vi "Gel Tugging Force Mode_Controller v16.20 DIC.vi"() -> ()   [LabVIEW 2015]
doc: "This example demonstrates how to continuously acquire voltage measurements from a DAQmx device using hardware timed, single point reads using a timed loop structure. The timed loop is controlled by the sample clock of the DAQ device. The device will read data on each tick of the sample clock. If an additional sample clock tick occurs before the current data point is read from the device or if the timed loop does not receive any sample clock ticks, a dialog will indicate that this has happened. \n\nHardware Timed Single Point acquisition works best when using a deterministic operating system (such as LabVIEW Real-Time). Because of the less deterministic nature of general purpose operating systems (such as Microsoft Windows), the software loop will not always take the exact same amount of time to execute, and this may lead to the occasional missed sample clock. \n\nFor instructions on how to connect your signals to the DAQ device, refer to your device documentation."
uses:
  <vilib>/Platform/TimedLoop/XDataNode/timing_clust.ctl
  <vilib>/Platform/TimedLoop/XDataNode/nitl_modes.ctl
  <vilib>/Platform/TimedLoop/XDataNode/wakeup.ctl
  <vilib>/dex/Flush And Wait Empty Condition.ctl
  <vilib>/DAQmx/read.llb/DAQmx Read (Analog 1D DBL NChan 1Samp).vi
  <vilib>/DAQmx/write.llb/DAQmx Write (Analog DBL 1Chan 1Samp).vi
  <vilib>/DAQmx/read.llb/DAQmx Read (Analog 2D DBL NChan NSamp).vi
  <vilib>/Analysis/baseanly.llb/Mean (DBL).vi
  <vilib>/DAQmx/create/channels.llb/DAQmx Create Channel (AI-Voltage-Basic).vi
  <vilib>/DAQmx/create/channels.llb/DAQmx Create Channel (AO-Voltage-Basic).vi
  <vilib>/DAQmx/configure/timing.llb/DAQmx Timing (Sample Clock).vi
  <vilib>/DAQmx/create/timing.llb/DAQmx Create Timing Source (Control Loop From Task).vi
  <vilib>/DAQmx/miscellaneous.llb/DAQmx Fill In Error Info.vi
  <vilib>/addons/control/pid/pid.llb/PID (DBL).vi
  <vilib>/addons/control/pid/pid.llb/PID Gain Schedule (DBL).vi
  <vilib>/platform/TimedLoop/XDataNode/XDataNode.xnode
  <vilib>/Analysis/NI_AALBase.lvlib
  <vilib>/addons/control/pid/NI_PID_pid.lvlib
  <vilib>/Platform/TimedLoop/XDataNode/XDNodeRunTimeDep.lvlib
  <vilib>/ptbypt/NI_PtbyPt.lvlib
panel:
  out "Zero Flux Observed GS":dbl
  in  "Start Null Flux Adjustment":bool=TRUE
  in  "3. Keep Null Flux Running \n       Until Next Step?":bool=TRUE
  in  "2. Adjust Magnetic Flux (GS):":dbl=3.0 min=-350.0 max=350.0 step=0.02 format="%#_13g"
  in  "4. Click Rocker to finish Null Flux Adjustment":bool
  out "Total seconds":dbl format="%.3f"
  out "Loop Index 2":dbl format="%.3f"
  out "Final AO (V)":dbl
  in  "1st OFF Length (s)":dbl=2.0
  out "Calibrating Sensor":bool
  out "Waveform Graph 2":dbl[](graph)
  in  "ON":dbl=3.0
  out "DigitalTrigger":bool
  out "Corrective \nNull Flux (Gs)":dbl
  out "# of Data Points":i64
  out "Loop Index":i32
  in  "Measure Flux Sensor Zero?":bool=TRUE
  out "PID gains ON Chosen":T1
  in  "Keep Null Flux Running \n       Until Next Step? 2":bool
  in  "Start Null Flux Adjustment 2":bool=TRUE
  out "PID gains OFF Chosen":T1
  in  "Tweaked PID gains ON":T1={"proportional gain (Kc)"=0.7, "integral time (Ti, min)"=3.5e-06, "derivative time (Td, min)"=0.0}
  in  "Tweaked PID gains OFF":T1={"proportional gain (Kc)"=0.078, "integral time (Ti, min)"=3.5e-06, "derivative time (Td, min)"=0.0}
  out "Ready?":bool
  in  "4. Aggressiveness:":i32(listbox)
  out "of":i32
  in  "3. PID Parameters:":i32(listbox)
  out "ON Absolute\nFlux Setpoint (Gs)":dbl
  out "Suggested PID gains OFF":T1
  out "Suggested PID gains ON":T1
  out "Measured Magnetic Sensor 1 Zero, Mean (V)":dbl format="%_7g"
  in  "2nd to last\n OFF (s)":dbl=7.0
  out "Round:":i32
  out "Ready?":bool
  out "Ready?":bool
  in  "Proceed with Parameters":bool=TRUE
  out "Final Flux Running at End?":bool
  out "Sensor Sensitivity \n(V/Gs)":dbl
  in  "1. Sensor:":i32(listbox)
  out "Ready?":bool
  in  "2. Needle:":i32(listbox)
  in  "Proceed with Selection":bool=TRUE
  in  "Ready?&\nData Logger Running":bool
  out "Null Flux \nCurrently\nRunning?":bool
  out "Real-Time Flux Control Currently Running?":bool
  out "Ready?":bool
  out "DeGaussing?":bool
  in  "Start DeGaussing":bool
  in  "1. Number of rounds":i32=3
  in  "Post-Wave Null Flux Interval (s)":dbl=7.5 format="%#_13g"
  in  "Pre-Wave Null Flux Interval (s)":dbl format="%#_13g"
  out "Flux Control Sequence Running & Uploading Data?":bool
  in  "Number of Cycles":i32=3
  in  "Flux ON relative setpoint (Gs)":dbl=-175.0 format="%#_13g"
  # "For Gel Tugging Experiments v16.20 (Controlled-Flux or Force Mode: DIC Part)"
  # "WARNING: This program can crash the first 2 or 3 times it runs after the target has been shut down. \nWARNING: Do NOT run the power supply unattended with the needle attached. Always check on the amount of current periodically."
  # "Step 0-1: Place the needle at Z ~ 7000 micron in the field of view. Inclincation Angle= 25º for HyMu80#1 Needle"
  # "(Hit \"Enter\" \nor Toggle)"
  # "Step 0-2: DeGauss Needle:"
  # "Step 0-3: Measure the Value of Flux Sensor \"Zero\"?"
  # "Yes"
  # "No"
  # "(Note: Check if it is around 2.47±0.02 (V)):"
  # "Step 1: Choose Sensor & \nNeedle/PID Parameters\nfor This Experiment:"
  # "Step 2: Adjust Flux: \n(in Real-Time)"
  # "(Hit \"Enter\" \nor Toggle)"
  # "Yes"
  # "No"
  # "Make sure upper side of Rocker\n is pressed down before Program Starts"
  # "Step 3: Specify Control \n     Sequence Parameters:"
  # "1. Pre-Wave Null Flux Interval (s) (choose 0 if none desired):"
  # "2. Length of 1st OFF"
  # "& ON"
  # "segments (s)."
  # "Length of 2nd to last OFF"
  # "Note 1: Use Negative Flux for waves in opposite direction\nNote 2: Linear Range is (±0-175 Gs) for Null Flux + Flux ON Setpoint\nNote 3: Check ON Absolute Flux Setpoint & PID Gains on first run.\nSometimes they can be glitchy. Abort & Re-run"
  # "3. Number of OFF & ON Square-Wave Cycles:"
  # "4. Flux ON relative setpoint (Gs):"
  # "5. Post-Wave Null Flux Inteval (s) (choose 0 if none desired):"
  # "No"
  # "Yes"
  # "Step 4: Do you want to tweak these PID parameters?"
  # "vs."
  # "Step 5: Run Data Logger: Gel Tugging Force Mode_Data Logger v16.10 DIC.vi\n            Needs to be running to start the control sequence"
  # "Step 6-1: Lower the needle to the desired level for the experiment. Z ~ 3400 microns with TI-SH-U stage.\nStep 6-2: Click TRGR or Run Macro in Nikon Elements"
  # "datapoints uploaded"
  # "out of"
  # "seconds elapsed"
  # "out of"
  # "Close the VI and start over. The VI sometimes freezes upon subsequent runs"
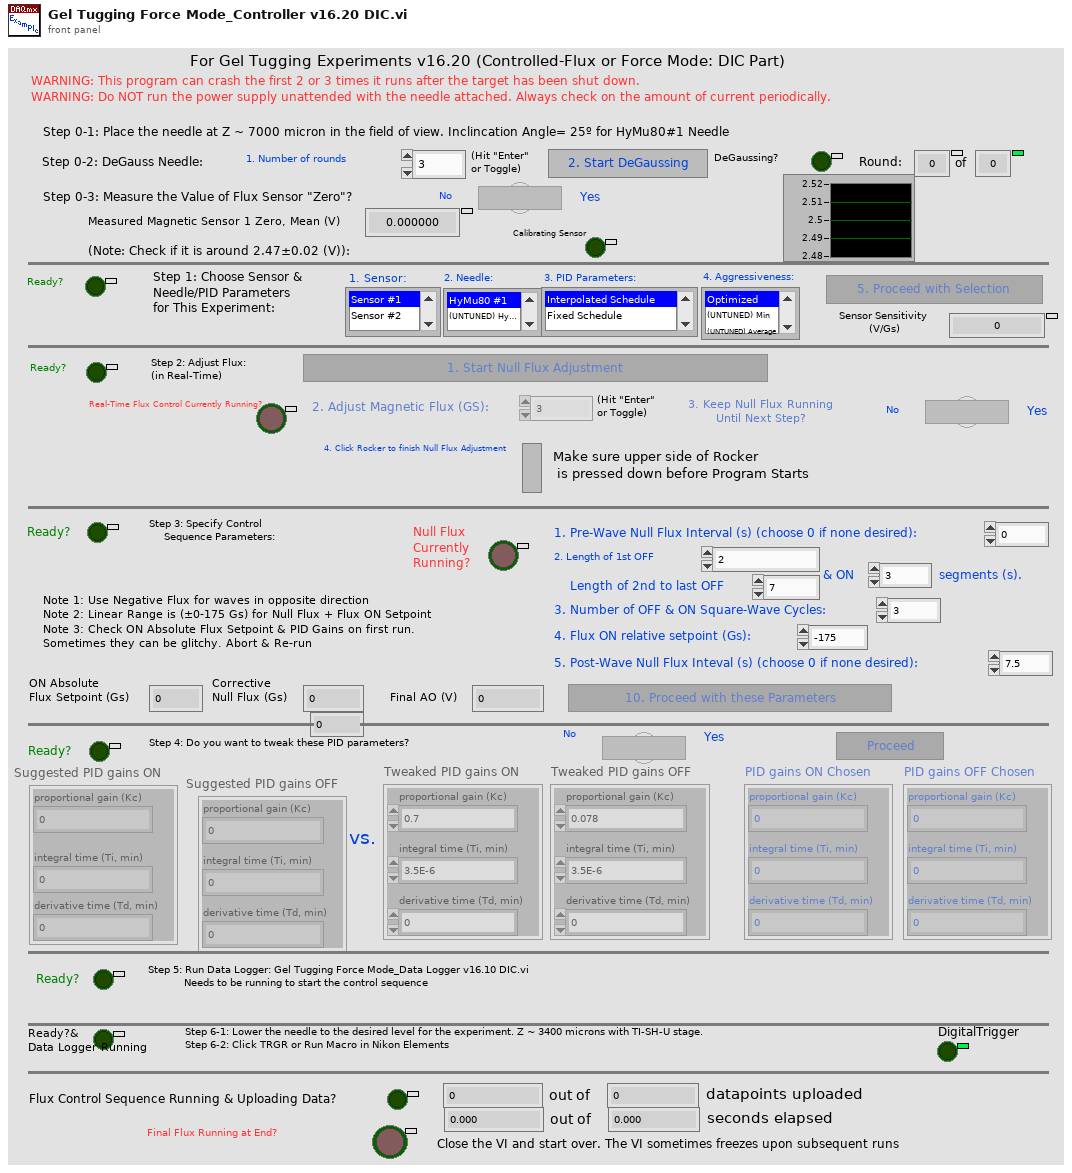
[diagram p1: front panel]
types:
  T1 = cluster{"proportional gain (Kc)":dbl, "integral time (Ti, min)":dbl, "derivative time (Td, min)":dbl}
  T2 = cluster{"PID gains":cluster{"proportional gain (Kc)":dbl, "integral time (Ti, min)":dbl, "derivative time (Td, min)":dbl}, "max value":dbl}[]
  T3 = typedef "XDNodeRunTimeDep.lvlib/timing_clust.ctl" = cluster{"Expected End [f-1]":u64, "Actual End [f-1]":u64, "Finished Late? [f-1]":bool, "Expected End [i-1]":u64, "Actual End [i-1]":u64, "Finished Late? [i-1]":bool, "Expected Start [i]":u64, "Actual Start [i]":u64, "Expected Start [f]":u64, "Actual Start [f]":u64, "Source Name":string, "Structure Name":string, "Period":i64, "Deadline":i64, "Offset":i64, "Start":i64, "Priority":i32, "Timeout":i32, "Mode":T4, "Wakeup Reason":T5, "Error":errorcluster, "Source Type":string, "Secondary Source Type":string, "Global End Time":u64, "Global Start Time":u64, "Frame Duration":u64, "Iteration Duration":u64, "Assigned CPU":i32, "I/O Scan Engine Mode":u32}
  T4 = typedef "XDNodeRunTimeDep.lvlib/nitl_modes.ctl" = enum32{"No Change", "Process missed periods, maintain original phase", "Discard missed periods, maintain original phase", "Process missed periods, ignore original phase", "Discard missed periods, ignore original phase"}
  T5 = typedef "XDNodeRunTimeDep.lvlib/wakeup.ctl" = enum32{"Normal", "Aborted", "Asynchronous wakeup", "Timing source error", "Timed loop error", "Timeout"}
  T6 = cluster{"Max/Min \ncontroller outputs":dbl, "output low":dbl}
  T7 = cluster{"PID gains":cluster{"proportional gain (Kc)":dbl, "integral time (Ti, min)":dbl, "derivative time (Td, min)":dbl}, "max value":dbl}
  T8 = typedef "Flush And Wait Empty Condition.ctl" = u8
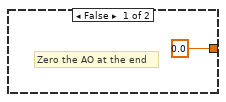
[diagram p2: hidden frame]
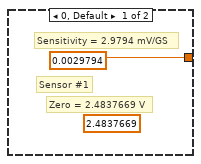
[diagram p4: hidden frame]
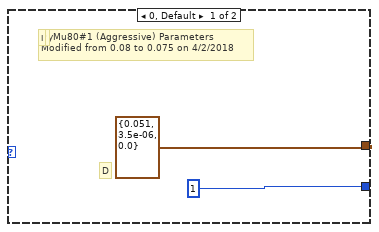
[diagram p5: hidden frame]
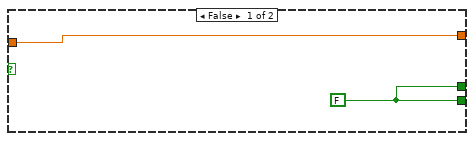
[diagram p6: hidden frame]
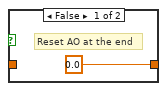
[diagram p7: hidden frame]
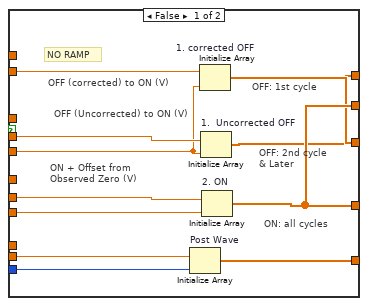
[diagram p9: hidden frame]
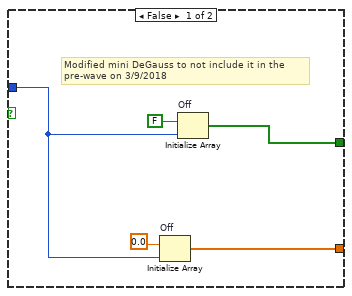
[diagram p11: hidden frame]
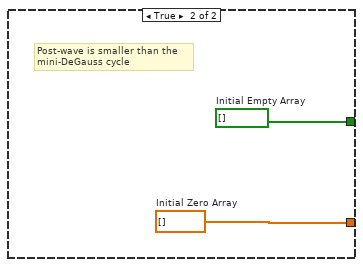
[diagram p12: hidden frame]
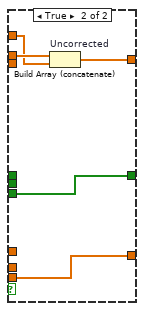
[diagram p14: hidden frame]
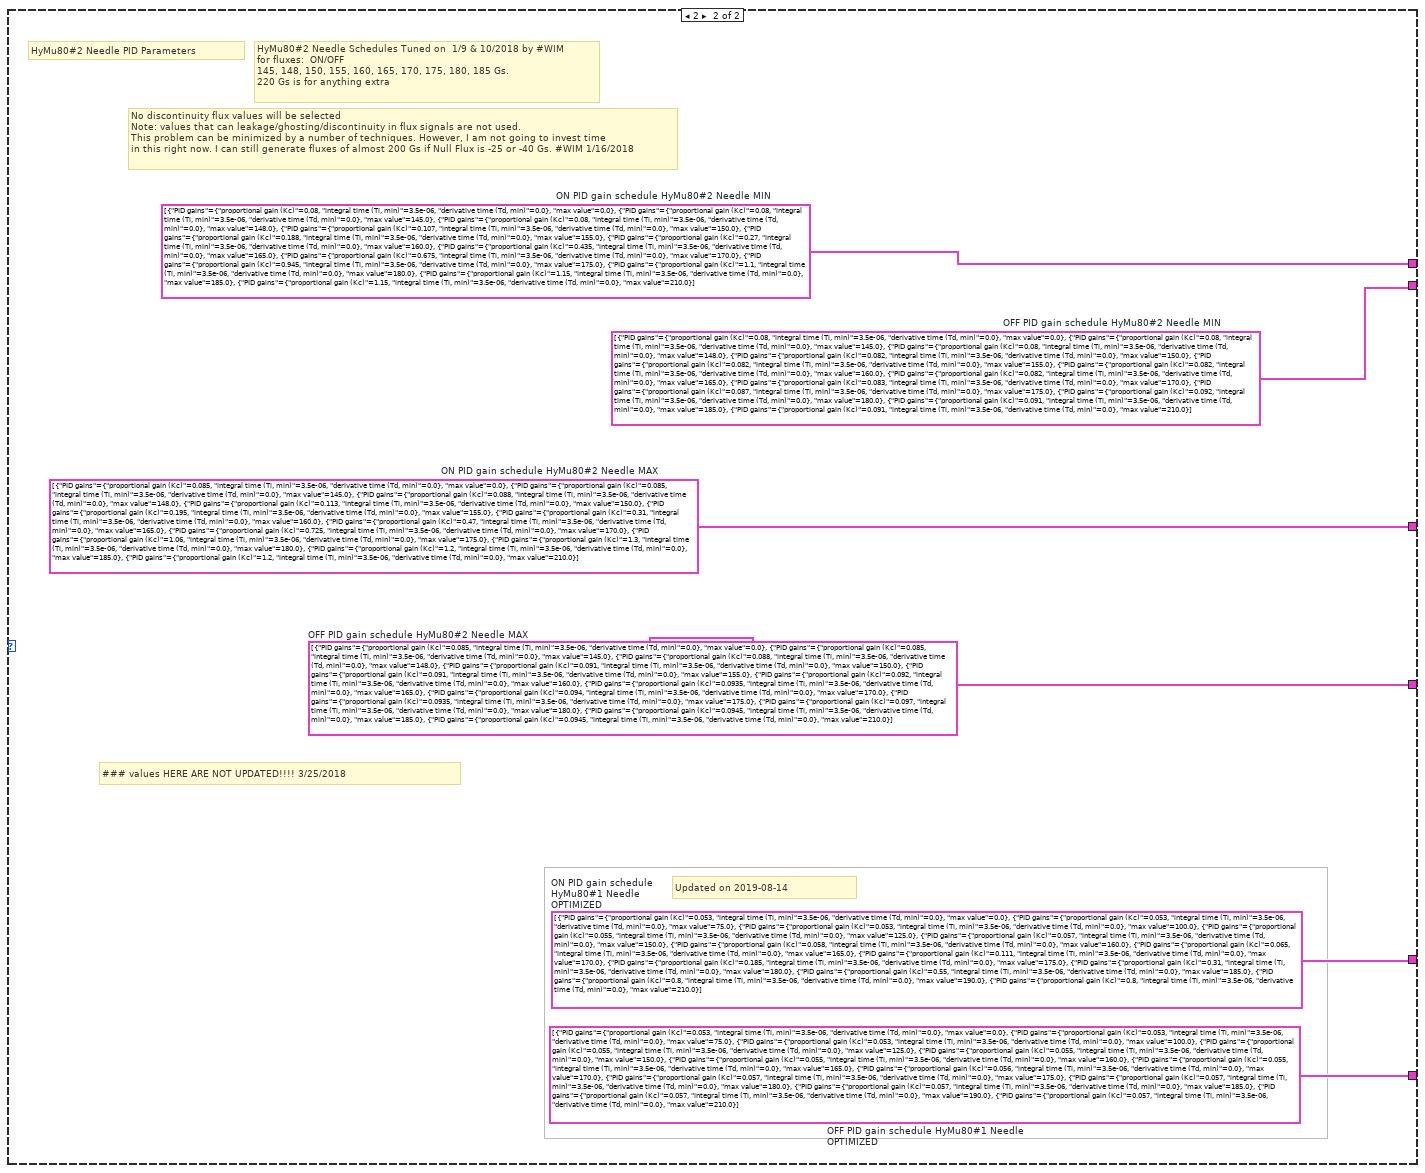
[diagram p18: hidden frame]
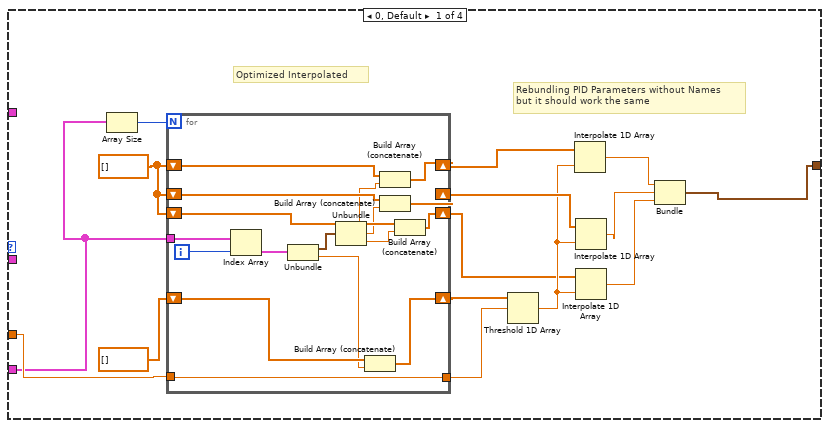
[diagram p19: hidden frame]
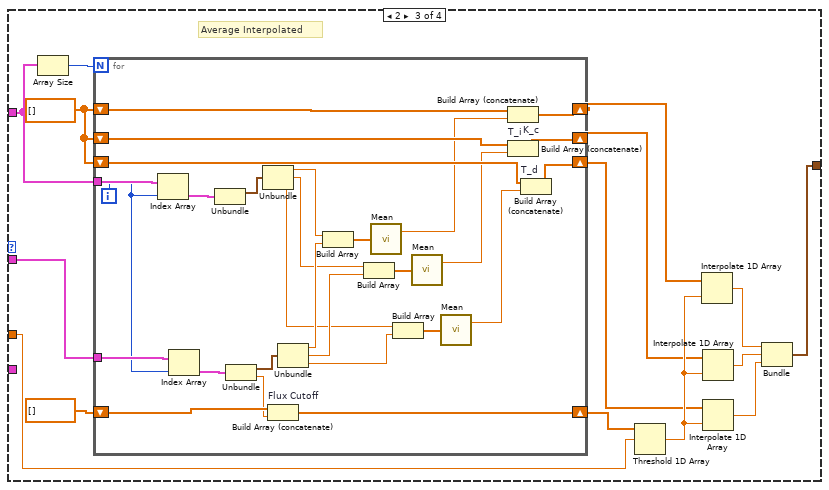
[diagram p20: hidden frame]
diagram:
  (unwired) T2 [{"PID gains"={"proportional gain (Kc)"=0.07, "integral time (Ti, min)"=3.5e-06, "derivative time (Td, min)"=0.0}, "max value"=0.0}, {"PID gains"={"proportional gain (Kc)"=0.07, "integral time (Ti, min)"=3.5e-06, "derivative time (Td, min)"=0.0}, "max value"=143.0}, {"PID gains"={"proportional gain (Kc)"=0.078, "integral time (Ti, min)"=3.5e-06, "derivative time (Td, min)"=0.0}, "max value"=148.0}, {"PID gains"={"proportional gain (Kc)"=0.078, "integral time (Ti, min)"=3.5e-06, "derivative time (Td, min)"=0.0}, "max value"=150.0}, {"PID gains"={"proportional gain (Kc)"=0.078, "integral time (Ti, min)"=3.5e-06, "derivative time (Td, min)"=0.0}, "max value"=155.0}, {"PID gains"={"proportional gain (Kc)"=0.078, "integral time (Ti, min)"=3.5e-06, "derivative time (Td, min)"=0.0}, "max value"=160.0}, {"PID gains"={"proportional gain (Kc)"=0.078, "integral time (Ti, min)"=3.5e-06, "derivative time (Td, min)"=0.0}, "max value"=165.0}, {"PID gains"={"proportional gain (Kc)"=0.078, "integral time (Ti, min)"=3.5e-06, "derivative time (Td, min)"=0.0}, "max value"=170.0}, {"PID gains"={"proportional gain (Kc)"=0.081, "integral time (Ti, min)"=3.5e-06, "derivative time (Td, min)"=0.0}, "max value"=175.0}, {"PID gains"={"proportional gain (Kc)"=0.081, "integral time (Ti, min)"=3.5e-06, "derivative time (Td, min)"=0.0}, "max value"=180.0}, {"PID gains"={"proportional gain (Kc)"=0.085, "integral time (Ti, min)"=3.5e-06, "derivative time (Td, min)"=0.0}, "max value"=185.0}, {"PID gains"={"proportional gain (Kc)"=0.086, "integral time (Ti, min)"=3.5e-06, "derivative time (Td, min)"=0.0}, "max value"=190.0}, {"PID gains"={"proportional gain (Kc)"=0.086, "integral time (Ti, min)"=0.01, "derivative time (Td, min)"=0.0}, "max value"=195.0}, {"PID gains"={"proportional gain (Kc)"=0.086, "integral time (Ti, min)"=0.01, "derivative time (Td, min)"=0.0}, "max value"=220.0}]  # OFF PID gain schedule HyMu80#1 Needle OPTIMIZED
  (unwired) T2 [{"PID gains"={"proportional gain (Kc)"=0.065, "integral time (Ti, min)"=3.5e-06, "derivative time (Td, min)"=0.0}, "max value"=0.0}, {"PID gains"={"proportional gain (Kc)"=0.065, "integral time (Ti, min)"=3.5e-06, "derivative time (Td, min)"=0.0}, "max value"=143.0}, {"PID gains"={"proportional gain (Kc)"=0.083, "integral time (Ti, min)"=3.5e-06, "derivative time (Td, min)"=0.0}, "max value"=148.0}, {"PID gains"={"proportional gain (Kc)"=0.084, "integral time (Ti, min)"=3.5e-06, "derivative time (Td, min)"=0.0}, "max value"=150.0}, {"PID gains"={"proportional gain (Kc)"=0.0875, "integral time (Ti, min)"=3.5e-06, "derivative time (Td, min)"=0.0}, "max value"=155.0}, {"PID gains"={"proportional gain (Kc)"=0.123, "integral time (Ti, min)"=3.5e-06, "derivative time (Td, min)"=0.0}, "max value"=160.0}, {"PID gains"={"proportional gain (Kc)"=0.187, "integral time (Ti, min)"=3.5e-06, "derivative time (Td, min)"=0.0}, "max value"=165.0}, {"PID gains"={"proportional gain (Kc)"=0.315, "integral time (Ti, min)"=3.5e-06, "derivative time (Td, min)"=0.0}, "max value"=170.0}, {"PID gains"={"proportional gain (Kc)"=0.46, "integral time (Ti, min)"=3.5e-06, "derivative time (Td, min)"=0.0}, "max value"=175.0}, {"PID gains"={"proportional gain (Kc)"=0.59, "integral time (Ti, min)"=3.5e-06, "derivative time (Td, min)"=0.0}, "max value"=180.0}, {"PID gains"={"proportional gain (Kc)"=0.8875, "integral time (Ti, min)"=3.5e-06, "derivative time (Td, min)"=0.0}, "max value"=185.0}, {"PID gains"={"proportional gain (Kc)"=1.04, "integral time (Ti, min)"=3.5e-06, "derivative time (Td, min)"=0.0}, "max value"=190.0}, {"PID gains"={"proportional gain (Kc)"=1.04, "integral time (Ti, min)"=0.01, "derivative time (Td, min)"=0.0}, "max value"=195.0}, {"PID gains"={"proportional gain (Kc)"=1.04, "integral time (Ti, min)"=0.01, "derivative time (Td, min)"=0.0}, "max value"=220.0}]  # ON PID gain schedule HyMu80#1 Needle OPTIMIZED
  (unwired) T2 [{"PID gains"={"proportional gain (Kc)"=0.07, "integral time (Ti, min)"=3.5e-06, "derivative time (Td, min)"=0.0}, "max value"=0.0}, {"PID gains"={"proportional gain (Kc)"=0.07, "integral time (Ti, min)"=3.5e-06, "derivative time (Td, min)"=0.0}, "max value"=116.0}, {"PID gains"={"proportional gain (Kc)"=0.078, "integral time (Ti, min)"=3.5e-06, "derivative time (Td, min)"=0.0}, "max value"=117.0}, {"PID gains"={"proportional gain (Kc)"=0.08, "integral time (Ti, min)"=3.5e-06, "derivative time (Td, min)"=0.0}, "max value"=120.0}, {"PID gains"={"proportional gain (Kc)"=0.08, "integral time (Ti, min)"=3.5e-06, "derivative time (Td, min)"=0.0}, "max value"=122.0}, {"PID gains"={"proportional gain (Kc)"=0.08, "integral time (Ti, min)"=3.5e-06, "derivative time (Td, min)"=0.0}, "max value"=125.0}, {"PID gains"={"proportional gain (Kc)"=0.08, "integral time (Ti, min)"=3.5e-06, "derivative time (Td, min)"=0.0}, "max value"=130.0}, {"PID gains"={"proportional gain (Kc)"=0.08, "integral time (Ti, min)"=3.5e-06, "derivative time (Td, min)"=0.0}, "max value"=135.0}, {"PID gains"={"proportional gain (Kc)"=0.08, "integral time (Ti, min)"=3.5e-06, "derivative time (Td, min)"=0.0}, "max value"=140.0}, {"PID gains"={"proportional gain (Kc)"=0.086, "integral time (Ti, min)"=3.5e-06, "derivative time (Td, min)"=0.0}, "max value"=145.0}, {"PID gains"={"proportional gain (Kc)"=0.096, "integral time (Ti, min)"=3.5e-06, "derivative time (Td, min)"=0.0}, "max value"=150.0}, {"PID gains"={"proportional gain (Kc)"=0.096, "integral time (Ti, min)"=3.5e-06, "derivative time (Td, min)"=0.0}, "max value"=200.0}]  # OFF PID gain schedule HyMu80#1 Needle OPTIMIZED
  (unwired) T2 [{"PID gains"={"proportional gain (Kc)"=0.07, "integral time (Ti, min)"=3.5e-06, "derivative time (Td, min)"=0.0}, "max value"=0.0}, {"PID gains"={"proportional gain (Kc)"=0.07, "integral time (Ti, min)"=3.5e-06, "derivative time (Td, min)"=0.0}, "max value"=116.0}, {"PID gains"={"proportional gain (Kc)"=0.08, "integral time (Ti, min)"=3.5e-06, "derivative time (Td, min)"=0.0}, "max value"=117.0}, {"PID gains"={"proportional gain (Kc)"=0.085, "integral time (Ti, min)"=3.5e-06, "derivative time (Td, min)"=0.0}, "max value"=120.0}, {"PID gains"={"proportional gain (Kc)"=0.115, "integral time (Ti, min)"=3.5e-06, "derivative time (Td, min)"=0.0}, "max value"=122.0}, {"PID gains"={"proportional gain (Kc)"=0.18, "integral time (Ti, min)"=3.5e-06, "derivative time (Td, min)"=0.0}, "max value"=125.0}, {"PID gains"={"proportional gain (Kc)"=0.31, "integral time (Ti, min)"=3.5e-06, "derivative time (Td, min)"=0.0}, "max value"=130.0}, {"PID gains"={"proportional gain (Kc)"=0.55, "integral time (Ti, min)"=3.5e-06, "derivative time (Td, min)"=0.0}, "max value"=135.0}, {"PID gains"={"proportional gain (Kc)"=0.95, "integral time (Ti, min)"=3.5e-06, "derivative time (Td, min)"=0.0}, "max value"=140.0}, {"PID gains"={"proportional gain (Kc)"=1.2, "integral time (Ti, min)"=3.5e-06, "derivative time (Td, min)"=0.0}, "max value"=145.0}, {"PID gains"={"proportional gain (Kc)"=1.3, "integral time (Ti, min)"=3.5e-06, "derivative time (Td, min)"=0.0}, "max value"=150.0}, {"PID gains"={"proportional gain (Kc)"=1.3, "integral time (Ti, min)"=3.5e-06, "derivative time (Td, min)"=0.0}, "max value"=200.0}]  # ON PID gain schedule HyMu80#1 Needle OPTIMIZED
  # "Note: Some quirks when running the program are: (as of 2/7/2018):\n1. First time you run it for the day, it will ask if you want to use the newer version instead of the old one already on the Remote Desktop computer\n2. Also, at the end of the first run, it will not stop. You will have to abort it. Some of the data points will be lost near the end. You might have to repeat that run.\n3. Do run the Data Reduction file or any other VIs in the DeGaussing stage. Otherwise, the program will crash."
  # "v15.20 Modified from v15.10 by Waddah Moghram on 2019-08-16 and thereafter:\n*Update based on Calibration_Core Flux Controller v11.00.vi\n\nv15.10 modified from v15.00 by  #Waddah #Moghram on 11/5/2018 and thereafter:\nTo be used with Data Logger v15.00 & Reduction v15.00: \n1. Modified it so that it can select PID gains from inside the loop\n2. Modified some PID gains at 170 Gs and higher.\n3.  Fixed the problem with the Post-wave zero Ramp 11/28/2019. WIM\n\nv 15.00 Modified from v12.00 by #Waddah #Moghram on 10/10/2018 and thereafter. To be used with Data Logger v1500 & Reduction v15.00: \n1. Replaced the Mini-DeGauss Routine with a Force Ramp (Linear vs. Steps?) since a step force function will be difficult to image-track. \n((Please refer to Linear and Step Ramps v1.00.vi for both linear and step ramps).\n*** Amount of step jump is assumed to be from ON-to-OFF and OFF-to-ON. That information is known\n2. Some of the parameters that will be used for the force ramp:\n*** Time interval: Assume that ON-to-OFF and OFF-to-ON ramps will have the same time frames.\n*** If discrete step are chosen. Choose the number of steps that it will take.\n\nv 11.00 Modified from v10.00 by #Waddah #Moghram on 4/26/2018 and thereafter. To be used with Data Logger v11.00 & Reduction v11.00: \n1. Resolve the issue of Digital Trigger automatically being released due to ground loop. Most likely due to construction that is happening around.\n* The Network digital trigger is released from the Master DAQ in the Data Logger, where it will be passed into here as a real-time global variable.\n2. For some reason, the first two runs usually crash, and the program still crashes a lot. I need to find a work around this one. \n\nv 10.00 Modified from v9.60 and v9.40 by #Waddah #Moghram on 4/4/2018 and thereafter: To be used with Data Logger v10.00 & Reduction v10.00\n1. Increased DeGauss Cycle to 2,000 milliseconds from 500 ms.\n2. Corrected the Dialog Boxes\n3. Added a switch for the Corrective Null Flux on the front panel, display it and send it to the Data Logger\n4. Corrected Mini-DeGauss Sampling Glitch where it was wired to the sampling rate directly instead of the one adjusted by the period 4/4/2018\n5. Based on a sigmoidal curve fit 4/18/2018.\nThe Equation is Y = Vmax * X^h /(K_prime + X^h), where Vmax = 10.7369, h = 1.91107, and Kprime = 3499.9. (and K_half = 71.5294))\n\n\nv 9.60 Modified from v9.50 by #Waddah #Moghram on 4/1/2018: \n1. It will correct for the Null Flux shift based on the Sigmoidal Fit that was collected from bead in front of the needle data,\nbased on a sigmoidal curve fit 4/2/2018. Experiments conducted 3/29/2018-4/2/2018. \nThe Equation is Y = Vmax * X^h /(K_prime + X^h), where Vmax = 11.4533, h = 1.69622, and Kprime = 1256.11)\n2. New Global Variable \"FluxObservedZeroGsCorrected\" to be inserted into the Data Logger v9.60\n\nv 9.50 Modified from v9.40 by #Waddah #Moghram on 3/29/2018:\n1. Used AI7 to hook up the 2nd Magnetic Sensor that will be placed in front of the sensor.\n2. Zero of 2nd Sensor is measured in the first step as well. The sensitivity is embedded in the data logger as well. \n3. Accompanies by v9.50 Data Logger.\n4. (GO BACK TO OLDER VERSION and add more details about modifications)\nFixed datapoints lost in the end due to the determinstic loop ending before the other loop. \n\nv 9.40 Modified from v9.20 by #Waddah #Moghram on 3/19/2018\n1. Removed Offset and kept amplitude +/- 10V for MiniDeGauss waveforms from inside the deterrministic loop.\n2. Shuffled the Suggested PID Loop parameters until before the \"Proceed button to allow the user to take a look at them. \n3. 3/22/2018. Reverted back to unshielded magnetic sensor, but with wire propped away from sensor.\nAlso, TI-SH-U is used and the needle is placed at Z~4600 microns for PID tuning with an inclination angle of 20 degrees\n(#OLD: 3. Re-optimized on 3/20/2018 for HyMu80#1 after shielding the sensor. The values were shifted down by 23 Gs   3/20/2018 )\n(#OLD: 4. Relocated PID Gains Selected on the front panel for more clarity 3/21/2018.)\n\nv 9.20 Modified from v9.05 and v9.10 by #Waddah #Moghram on 3/12/2018 and thereafter:\n1. It is back to OFF/ON Sequences, except first OFF segment and pre-waves have no DeGauss. It turns out to be an easy fix. \n2. Modified mini-DeGauss time \n3. Tied variables to make the wave sample properly. See notes for calculations.\n4. Turn OFF \"Null Flux Running Middle\" when control sequence starts. 3/17/2018 WIM \n5. Modified PID Parameters for #Interpolated #Optimized #HyMu80#1. Other parameters will need to be modified later on. \n6. Updated front panel to indicate inclination Angle, and Z-level for both Sensor Zero Measurement and Control Sequence.   3/18/2018\n****It turns out the PID parameters are sensitive to both z-level and inclination angle (which affect the Sensor Zero Measurement).*****\n***NOTE: First run usually does not end by itself. You will have to abort it. It will result in the loss of the last few hundred data points, but that is not too critical. Otherwise, run once, then run again. It should run smoothly every time afterwards. This is one of the quirks of working with LabVIEW. 3/18/2018\n\nv 9.05 Modified from v9.00 by #Waddah #Moghram on 3/12/2018:\n1. Modified Magnitude of Mini-DeGauss cycle from ** Maximum of (AO of Null Flux (AO_nf) or AO of ON (AO_on)) ** to **AO_nf + AO_on**\n2. The mini DeGauss oscillates about AO_nf instead of 0\n\nv 9.00 Modified from v8.40 by #Waddah #Moghram on 3/7/2018 and thereafter:\n1. It will include mini-DeGauss Cycles in the beginning of the OFF segments before PID control kicks back in. This is in an effort to minimize Magnetic Sensor hysteresis at Null Flux Observed\n(Sinusoidally Decaying Waveform Embedded in Control Sequence v1.0.vi is used for initially testing of mini-DeGauss waveforms).\n** So far, the selected waveform is about ~ 15 cycles that exponentially decay under 30 milliseconds. Used a Cosine waveform instead of sine (Sin with 90 degree phase shift).\n** Middle point is AO = 0, Magnitude between max and middle point is AO_last**    (3/12/2018)\n2. Sequence is created externally to minimize Loop calculation time. The AO Mini-DeGauss will only to be multiplied by the amplitude of the last AO out. \n3. Switched #AI6 to #AI3. Some errors with AI6 signal on the DAQ on 3/8/2018\n4. Fixed the glitch where the PID loop overreacted when the PID starts again and the Setpoint point is close to the Process variable. (Kudos to #Dr. #Selby for catching it!). on 3/8/2018\n5. Replaced \"Zero Flux\" with \"Null Flux\" for labels to avoid confusion since it is not really zero\n\nv 8.40 Modified from v8.30 by #Waddah #Moghram on 3/1/2018, and thereafter: \n1. Added a toggle to allow the re-calibration of magnetic sensor Zero or not\n2. Global Variables for DeGauss Cycles Total & Round\n3. Modified Tabbing order on 3/4/2018\n4. Fixed AO 0 initialized before PID loop to keep the value saved from \"keep Null Flux Running\" step on 3/5/2018. It was creating a blip in PID response. However, that does not seem to resolve the problem.\n\nv 8.30 Modified from v8.20 by #Waddah #Moghram on 2/22/2018:\n1. Using the measured magnetic sensor zero to create the control sequence after DeGaussing instead of the one recorded a while back inside a shielded data.\nThis is because it will change a lot over time with thermal drift and so forth. \n2. Reset the value of the sensor zero every time even no deGaussing was done.\n\nv 8.20 Modified from v8.10 by #Waddah #Moghram on 2/2/2018: \n1. This will allow the user to tweak the PID Parameters one more time before the actual experiment. This was found because it turns out that PID parameters can shift with time especially for values in the non-linear range.\n\nv. 8.10 Modified from v8.00 by #Waddah #Moghram on 1/10/2018 and thereafter:\n1. Scrapped fitted PID gains and used interpolated schedules in addition to schedules\n2. Updated PID Values for Gains and so forth.\n\nv 8.00 Modified from v7.40 by #Waddah #Moghram on 1/1/2018 and thereafter:\n1. Used the PID Gains from PID Tuning experiments \n2. Removed Normal vs. Aggressive and now will only use one set of parameters such that only one set of parameters are used\n3. Created a choice of Scheduled vs. Fitted Parameters. 1/8/2018.\n4. Fixed glitch that passed old values of waveform parameters to the global variable 1/8/2018. \n\nv 7.40 Modified from v 7.30 by #Waddah #Moghram on 12/22/2017 to including the following:\n1. Shifting the flux check and current reset only if DeGuassing Cycle required is not equal to zero. Otherwise, skip it, and keep the current running. I did this in case I need more than one run without removing the needle from the sample\n2. corrected total number of data points to allow for more than 2 seconds 1/4/2018 by #WIM\n\nv 7.30 Modified from v 7.20 by #Waddah #Moghram on 12/21/2017 to including the following:\n1. Removed Magnetic Flux Sensor Zero Calibration step, and embedded that value in the sensor section. The idea for doing that is that I want the flux values stated to be absolute. Thermal drift of sensor should not matter since PID should still work regardless of where the zero lies. Moreover, if I am accounting for the Null Flux observed, it should not matter what the absolute flux zero is.\n2. However, I kept the AO reset and used the AI2 to keep it running and also measured sensor values for 2 seconds to make sure that my values are controlled properly.\n3. Steps were re-numbered\n\nv 7.20 Modified from v7.10 by #Waddah #Moghram on 12/18/2017 to include the following:\n1. Custom-Length Waveforms. Data Reduction & Logger will be changed accordingly.\n2. Added Normal (~40 ms response time) vs. Aggressive (~22 ms response time) PID Parameters on 12/20/2017\n\nV 7.10 Modified from v7.00 by #Waddah #Moghram on 12/18/2017 to include the following:\n1. Switch order of DeGaussing & Calibrating Zero of Sensor. First Ensure that there is no residual magnetic. And secondly, reset AO just in case!\n\nv 7.00 Modified from v6.00 by #Waddah #Moghram on 12/18/2017 to include the following:\n1. Calibrated Null Flux at the beginning of the experiment without shielding to account for thermal drifts:\n*** Imported from \"01 Magnetic Sensor Zero Calibration v2.0 - Target.vi\"\n2. Included Second per Cycle\n3. Cleanup interface & Changed Step Numbers.\n\nv 6.00 Modified from v5.22 by #Waddah #Moghram on 12/5/2017 to include the following: \n1. Newer Magnetic Sensor Sensitivities: Sensor 1 is 2.9794 mV/GS and Sensor 2 is 3.0418 mV/GS\n2. Newer Magnetic Sensor Zeroes when unshielded: Sensor 1 is 2.4837669 V and Sensor 2 is 2.4928421 V\nThis program will also be used also to tune the PID in addition Magnetic Needle Choices\nOn 12/13/2017, I overhauled the interface to streamline the proceess and fixed a few glitches that allowed the program to \nchose parameters before clicking on the digital trigger\n\nv 5.22 Modified from v.5.20 by #Waddah #Moghram on 9/25/2017 to include the following:\n1. Remove prompt to calibrate the magnetic sensor and run Null Flux program\n2. Embedded the calibrated Null Flux value into the program, now that the sensor is fixed to the HyMu80 needle #1\n\n\nv5.00 modified from v.3.70 and v.4.10 by #Waddah #Moghram. It should integrate variables from both VIs.\nOther modification include:\n1. User-Defined Pre-experiment Null Flux Period\n2. User-Defined Post-experiment Null Flux Period\nModified on 8/14&15/2017 to streamline the VI even more. Ran into some Ground Loop Issues in the meantime. See Lab Notes for details.\n\nv4.10 Modified on 8/8/2017 to:\n* account for AI5 only for flux sensor values being fed to PID control.\nNotice the PID control scheme process variable is different in that it is not subtracted from the setpoint as in v.3.70 in the first PID Loop\n*modified PID parameters to the optimized ones found (subject to verification)."
  # "Re-optimized on 3/21/2018 for HyMu80#1 after shielding the sensor. The cutoff values were shifted down by ~23-27 Gs\nPreviously Optimized on 3/17/2018 for HyMu80#1 Optimized. The rest will need to be updated later\nAdded 139 Gs to keep fixed values in between 0 and 140 Gs.   Flux at 150 Gs has a response time of ~80 ms. \nAny higher PID gains will result in spike"
  # "Unshielded Previously"
  # "TOTALLY SHIELDED PARAMETERS"
  # "AI"
  # "AO"
  n1 = flat-sequence {
    tunnel: [w335] -> w102
    tunnel: [w334] -> w101
    tunnel: [w333] -> w94
    tunnel: [w332] -> w82
    tunnel: [w347] -> w110
    tunnel: w102 -> [w345]
    tunnel: w101 -> [w344]
    tunnel: w94 -> [w343]
    tunnel: [w343] -> w93
    tunnel: [w342] -> w83
    tunnel: w82 -> [w342]
    tunnel: [w357] -> w111
    tunnel: w110 -> [w357]
    tunnel: w93 -> [w356]
    tunnel: [w356] -> w92
    tunnel: [w355] -> w84
    tunnel: w83 -> [w355]
    tunnel: w111 -> [w361]
    tunnel: [w360] -> w108
    tunnel: [w359] -> w96
    tunnel: w92 -> [w359]
    tunnel: [w358] -> w85
    tunnel: w84 -> [w358]
    tunnel: [w372] -> w117
    tunnel: [w371] -> w116
    tunnel: [w370] -> w115
    tunnel: [w369] -> w109
    tunnel: w108 -> [w369]
    tunnel: w96 -> [w368]
    tunnel: [w368] -> w95
    tunnel: [w366] -> w91
    tunnel: w85 -> [w367]
    tunnel: [w367] -> w81
    tunnel: w117 -> [w414]
    tunnel: w116 -> [w413]
    tunnel: w115 -> [w412]
    tunnel: [w411] -> w114
    tunnel: [w410] -> w113
    tunnel: [w409] -> w112
    tunnel: w109 -> [w401]
    tunnel: [w399] -> w98
    tunnel: w95 -> [w399]
    tunnel: w91 -> [w398]
    tunnel: w81 -> [w397]
    tunnel: [w397] -> w79
    tunnel: [w396] -> w64
    tunnel: [w394] -> w2
    tunnel: w114 -> [w490]
    tunnel: w113 -> [w489]
    tunnel: w112 -> [w488]
    tunnel: w98 -> [w487]
    tunnel: [w487] -> w97
    tunnel: [w486] -> w80
    tunnel: w79 -> [w486]
    tunnel: [w485] -> w65
    tunnel: w64 -> [w485]
    tunnel: [w484] -> w3
    tunnel: w2 -> [w484]
    tunnel: [w499] -> w100
    tunnel: w97 -> [w499]
    tunnel: w80 -> [w498]
    tunnel: [w498] -> w77
    tunnel: w65 -> [w497]
    tunnel: [w497] -> w62
    tunnel: w3 -> [w496]
    tunnel: [w510] -> w107
    tunnel: [w509] -> w106
    tunnel: [w508] -> w105
    tunnel: [w507] -> w104
    tunnel: [w506] -> w103
    tunnel: w100 -> [w505]
    tunnel: [w505] -> w99
    tunnel: [w504] -> w78
    tunnel: w77 -> [w504]
    tunnel: [w503] -> w63
    tunnel: w62 -> [w503]
    tunnel: [w502] -> w17
    tunnel: [w501] -> w16
    tunnel: [w500] -> w1
    tunnel: [w529] -> w89
    tunnel: [w522] -> w90
    tunnel: [w687] -> w88
    tunnel: [w679] -> w87
    tunnel: w107 -> [w608]
    tunnel: w106 -> [w678]
    tunnel: w105 -> [w677]
    tunnel: w104 -> [w676]
    tunnel: w103 -> [w675]
    tunnel: [w674] -> w86
    tunnel: w99 -> [w674]
    tunnel: w78 -> [w673]
    tunnel: [w673] -> w76
    tunnel: w63 -> [w672]
    tunnel: [w672] -> w61
    tunnel: [w658] -> w56
    tunnel: [w644] -> w55
    tunnel: [w623] -> w52
    tunnel: [w617] -> w49
    tunnel: w17 -> [w531]
    tunnel: w16 -> [w603]
    tunnel: [w531] -> w7
    tunnel: w1 -> [w521]
    tunnel: w90 -> [w832]
    tunnel: [w818] -> w75
    tunnel: w89 -> [_]
    tunnel: w88 -> [w829]
    tunnel: [w817] -> w73
    tunnel: [w844] -> w71
    tunnel: w87 -> [w836]
    tunnel: [w835] -> w69
    tunnel: [w843] -> w67
    tunnel: w86 -> [w849]
    tunnel: w76 -> [w848]
    tunnel: w61 -> [w830]
    tunnel: [w830] -> w59
    tunnel: [w837] -> w58
    tunnel: w56 -> [w838]
    tunnel: w55 -> [w834]
    tunnel: [w833] -> w54
    tunnel: w52 -> [w846]
    tunnel: [w846] -> w51
    tunnel: w49 -> [w845]
    tunnel: [w845] -> w48
    tunnel: [w842] -> w15
    tunnel: [w841] -> w14
    tunnel: w7 -> [w840]
    tunnel: w75 -> [w1265]
    tunnel: [w1265] -> w74
    tunnel: w73 -> [w1264]
    tunnel: [w1264] -> w72
    tunnel: w71 -> [w1262]
    tunnel: [w1258] -> w70
    tunnel: w69 -> [w1263]
    tunnel: [w1263] -> w68
    tunnel: w67 -> [w1261]
    tunnel: [w1257] -> w66
    tunnel: [w1256] -> w60
    tunnel: w59 -> [w1256]
    tunnel: w58 -> [w1255]
    tunnel: [w1255] -> w57
    tunnel: w54 -> [w1254]
    tunnel: [w1254] -> w53
    tunnel: w51 -> [w1253]
    tunnel: [w1253] -> w50
    tunnel: w48 -> [w1252]
    tunnel: [w1252] -> w47
    tunnel: w15 -> [w1249]
    tunnel: w14 -> [w1248]
    tunnel: [w1249] -> w13
    tunnel: [w1248] -> w12
    tunnel: w74 -> [w1303]
    tunnel: [w1305] -> w46
    tunnel: [w1306] -> w44
    tunnel: [w1298] -> w42
    tunnel: [w1303] -> w40
    tunnel: [w1287] -> w39
    tunnel: [w1302] -> w38
    tunnel: w72 -> [w1295]
    tunnel: [w1295] -> w36
    tunnel: [w1299] -> w34
    tunnel: w70 -> [w1299]
    tunnel: w68 -> [w1301]
    tunnel: [w1301] -> w32
    tunnel: w66 -> [w1300]
    tunnel: [w1300] -> w31
    tunnel: w60 -> [w1296]
    tunnel: [w1296] -> w30
    tunnel: w57 -> [w1294]
    tunnel: [w1294] -> w28
    tunnel: w53 -> [w1293]
    tunnel: [w1293] -> w26
    tunnel: [w1292] -> w24
    tunnel: w50 -> [w1292]
    tunnel: w47 -> [w1291]
    tunnel: [w1291] -> w23
    tunnel: w13 -> [w1289]
    tunnel: w12 -> [w1290]
    tunnel: [w1290] -> w11
    tunnel: [w1289] -> w10
    tunnel: w46 -> [w1331]
    tunnel: [w1330] -> w45
    tunnel: w44 -> [w1333]
    tunnel: [w1332] -> w43
    tunnel: w42 -> [w1335]
    tunnel: [w1334] -> w41
    tunnel: w40 -> [w1337]
    tunnel: w39 -> [w1339]
    tunnel: w38 -> [w1357]
    tunnel: [w1356] -> w37
    tunnel: w36 -> [w1343]
    tunnel: [w1342] -> w35
    tunnel: w34 -> [w1350]
    tunnel: [w1351] -> w33
    tunnel: w32 -> [w1349]
    tunnel: w31 -> [w1353]
    tunnel: w30 -> [w1355]
    tunnel: [w1354] -> w29
    tunnel: w28 -> [w1347]
    tunnel: [w1346] -> w27
    tunnel: w26 -> [w1345]
    tunnel: [w1344] -> w25
    tunnel: w24 -> [_]
    tunnel: w23 -> [w1341]
    tunnel: [w1340] -> w22
    tunnel: [w1352] -> w21
    tunnel: [w1348] -> w20
    tunnel: [w1338] -> w19
    tunnel: [w1336] -> w18
    tunnel: w11 -> [w1329]
    tunnel: w10 -> [w1328]
    tunnel: [w1327] -> w9
    tunnel: [w1326] -> w8
    tunnel: w45 -> [w1443]
    tunnel: w43 -> [w1444]
    tunnel: w41 -> [w1440]
    tunnel: w37 -> [w1409]
    tunnel: [w1426] -> w6
    tunnel: [w1411] -> w5
    tunnel: w35 -> [w1378]
    tunnel: [w1401] -> w4
    tunnel: w33 -> [w1400]
    tunnel: w29 -> [w1392]
    tunnel: w27 -> [w1399]
    tunnel: w25 -> [w1397]
    tunnel: w22 -> [w1389]
    tunnel: w21 -> [w1405]
    tunnel: w20 -> [w1407]
    tunnel: w19 -> [w1398]
    tunnel: w18 -> [w1436]
    tunnel: w9 -> [w1384]
    tunnel: w8 -> [w1382]
    tunnel: w6 -> [w1670]
    tunnel: w5 -> [w1669]
    tunnel: w4 -> [w1671]
    frame #0 {
      (unwired) "BEFORE YOU START: \n* VERIFY these DAQ-2/Slave cables are connected as the following:\n   * AI5 is connected to Magnetic Flux \"Sensor Output - RAW\" on the Magnetic sensor box.   \n   * AI3 is connected to \"Current Sensor (1A/V)\" on the Load Box.\n   * AI7 is connected to Camera \"Exposure Sensor.\"\n   * Digital Trigger from DAQ-3/Master Output \"PF0.0\" is connected to Digital Trigger Input \"PFI0.\"\n* VERIFY these DAQ-3/Master Cables are connected as the following:\n   * Digital Trigger is connected to \"PF0.0\" BOTH \"PFI0\" on the same board and to \"PFI0\" on DAQ2/Slave.\n  \n* TURN ON power supply for half an hour. TURN ON fan control for load box (if needed).\n           WARNING: Check load is connected at the back of the load box to the back of the  power supply.\n           WARNING: Check if magnetic coil is connected to the load box if the toggle is switched to \"COIL+1OHM RESISTOR\" on the Load Box.\n           WARNING: Do NOT Position Needle in solution/cells just yet.\n           WARNING: Do NOT Position Needle in solution/cells just yet.\nIf you have not done these steps. Stop the program, then run it when ready.\n===============================\nClick OK then follow the steps"
      # "Removed the thermocouple  * AI2 is connected to Thermocouple cable."
      # "Switched Ai6 to AI3 on 3/8/2018 \nSome issues with AI6 on DEV2"
      # "1. SPECIFY the number of DeGaussing Cycle. CLICK \"Start DeGaussing.\"\n2. SPECIFY the Sensor & Needle in use for this experiment."
    }
    frame #1 {
      w121 = 0.0 ("DataRT Index")
      w129 = tag "Dev2/ai4, Dev2/ai5, Dev2/ai6,Dev2/ai7"  # AI2:Dummy,AI3: Current, AI4: Dummy,AI5:Flux, AI7: Camera  Changed Ai5 to Ai1 on 2021-04-13
      w133 = FALSE ("DeGuassing Needle")
      # "Added on 4/24/2018"
      # "RESET VARIABLES"
      n2 = shared-variable ".\\Kopco PS Project Target Variables Library.lvlib\\Data Logger Running RT"(w133) -> ()  [unwired: 1 in, 1 out]
      n3 = shared-variable "NI-GenericDesktopPC-3A84958E\\Kopco PS Project Target Variables Library.lvlib\\Needle Selection Finished"(w133) -> ()  [unwired: 1 in, 1 out]
      n4 = shared-variable "NI-GenericDesktopPC-3A84958E\\Kopco PS Project Target Variables Library.lvlib\\Control Parameters Selected"(w133) -> ()  [unwired: 1 in, 1 out]
      n5 = shared-variable "NI-GenericDesktopPC-3A84958E\\Kopco PS Project Target Variables Library.lvlib\\DeGuassing Finished"(w133) -> ()  [unwired: 1 in, 1 out]
      n6 = shared-variable "NI-GenericDesktopPC-3A84958E\\Kopco PS Project Target Variables Library.lvlib\\DeGuassing Needle"(w133) -> ()  [unwired: 1 in, 1 out]
      n7 = shared-variable "NI-GenericDesktopPC-3A84958E\\Kopco PS Project Target Variables Library.lvlib\\Null Flux Selected"(w133) -> ()  [unwired: 1 in, 1 out]
      n8 = shared-variable ".\\Kopco PS Project Target Variables Library.lvlib\\Data Upload"(w133) -> ()  [unwired: 1 in, 1 out]
      n9 = shared-variable "NI-GenericDesktopPC-3A84958E\\Kopco PS Project Target Variables Library.lvlib\\Flux RT Control"(w133) -> ()  [unwired: 1 in, 1 out]
      n10 = shared-variable "NI-GenericDesktopPC-3A84958E\\Kopco PS Project Target Variables Library.lvlib\\Flux Control Sequence Running"(w133) -> ()  [unwired: 1 in, 1 out]
      n11 = shared-variable "NI-GenericDesktopPC-3A84958E\\Kopco PS Project Target Variables Library.lvlib\\Null Flux Running Middle"(w133) -> ()  [unwired: 1 in, 1 out]
      n12 = shared-variable "NI-GenericDesktopPC-3A84958E\\Kopco PS Project Target Variables Library.lvlib\\Null Flux Running End"(w133) -> ()  [unwired: 1 in, 1 out]
      n13 = shared-variable "NI-GenericDesktopPC-3A84958E\\Kopco PS Project Target Variables Library.lvlib\\Zero Flux Calibrated Found"(w133) -> ()  [unwired: 1 in, 1 out]
      n14 = shared-variable "NI-GenericDesktopPC-3A84958E\\Kopco PS Project Target Variables Library.lvlib\\PID Parameters Selected"(w133) -> ()  [unwired: 1 in, 1 out]
      n15 = shared-variable "NI-GenericDesktopPC-3A84958E\\Kopco PS Project Target Variables Library.lvlib\\Digital Trigger"(w133) -> ()  [unwired: 1 in, 1 out]
      n16 = shared-variable ".\\Kopco PS Project Target Variables Library.lvlib\\Data Logger Running"(w133) -> ()  [unwired: 1 in, 1 out]
      n17 = shared-variable ".\\Kopco PS Project Target Variables Library.lvlib\\Data RT Flux"(w121) -> ()  [unwired: 1 in, 1 out]
      n18 = shared-variable ".\\Kopco PS Project Target Variables Library.lvlib\\Data RT Exposure"(w121) -> ()  [unwired: 1 in, 1 out]
      n19 = shared-variable ".\\Kopco PS Project Target Variables Library.lvlib\\Data RT Current"(w121) -> ()  [unwired: 1 in, 1 out]
      n20 = shared-variable ".\\Kopco PS Project Target Variables Library.lvlib\\Data RT Index"(i64 0 ("DataRT Index")) -> ()  [unwired: 1 in, 1 out]
      n21 = shared-variable ".\\Kopco PS Project Target Variables Library.lvlib\\Last Current AO"(0.0 ("Last Current AO")) -> ()  [unwired: 1 in, 1 out]
      n22 = shared-variable "NI-GenericDesktopPC-3A84958E\\Kopco PS Project Target Variables Library.lvlib\\Flux Setpoint ON Gs Relative"(-175.0 ("Zero Flux Observed GS")) -> ()  [unwired: 1 in, 1 out]
      n23 = shared-variable "NI-GenericDesktopPC-3A84958E\\Kopco PS Project Target Variables Library.lvlib\\Experiment Settings Entered"(w133) -> ()  [unwired: 1 in, 1 out]
      n24 = shared-variable "NI-GenericDesktopPC-3A84958E\\Kopco PS Project Target Variables Library.lvlib\\Sensor Zero Calibrating"(w133) -> ()  [unwired: 1 in, 1 out]
      n25 = shared-variable "NI-GenericDesktopPC-3A84958E\\Kopco PS Project Target Variables Library.lvlib\\Ramp Total Interval (ms)"(i16 0 ("Ramp Total Interval (ms)")) -> ()  [unwired: 1 in, 1 out]
      n26 = shared-variable "NI-GenericDesktopPC-3A84958E\\Kopco PS Project Target Variables Library.lvlib\\Ramp Steps"(i16 0 ("Ramp Steps")) -> ()  [unwired: 1 in, 1 out]
      n27 = shared-variable "NI-GenericDesktopPC-3A84958E\\Kopco PS Project Target Variables Library.lvlib\\Zero Flux Observed GS"(3.0 ("Zero Flux Observed GS")) -> ()  [unwired: 1 in, 1 out]
      n28 = shared-variable "NI-GenericDesktopPC-3A84958E\\Kopco PS Project Target Variables Library.lvlib\\DeGauss Round Num"(i16 0 ("DeGauss Round Num")) -> ()  [unwired: 1 in, 1 out]
      n29 = shared-variable "NI-GenericDesktopPC-3A84958E\\Kopco PS Project Target Variables Library.lvlib\\DeGauss Total"(i16 0 ("DeGauss Total")) -> ()  [unwired: 1 in, 1 out]
      n30 = shared-variable "NI-GenericDesktopPC-3A84958E\\Kopco PS Project Target Variables Library.lvlib\\Cycles"(i16 0 ("Cycles")) -> ()  [unwired: 1 in, 1 out]
      n31 = shared-variable "NI-GenericDesktopPC-3A84958E\\Kopco PS Project Target Variables Library.lvlib\\Channels AI List"(w129) -> ()  [unwired: 1 in, 1 out]
      n32 = shared-variable "NI-GenericDesktopPC-3A84958E\\Kopco PS Project Target Variables Library.lvlib\\Sampling Rate"(30000.0 ("Sampling Rate")) -> ()  [unwired: 1 in, 1 out]
      n33 = shared-variable "NI-GenericDesktopPC-3A84958E\\Kopco PS Project Target Variables Library.lvlib\\Sensor Index Flux Core"(i8 1 ("Sensor Index Flux Core")) -> ()  [unwired: 1 in, 1 out]
      n34 = shared-variable "NI-GenericDesktopPC-3A84958E\\Kopco PS Project Target Variables Library.lvlib\\Sensor Index Camera"(i8 3 ("Sensor Index Flux Core")) -> ()  [unwired: 1 in, 1 out]
      n35 = shared-variable "NI-GenericDesktopPC-3A84958E\\Kopco PS Project Target Variables Library.lvlib\\Sensor Index Current"(i8 0 ("Sensor Index Flux Core")) -> ()  [unwired: 1 in, 1 out]
    }
    frame #2 {
      # "#STEP #0"
      n36 = while {
        tunnel: ["Start DeGaussing"] -> w134
        stop <- "Start DeGaussing" stop-if-true
      }
      n37 = shared-variable "NI-GenericDesktopPC-3A84958E\\Kopco PS Project Target Variables Library.lvlib\\DeGuassing Needle"(w134) -> ()  [unwired: 1 in, 1 out]
    }
    frame #3 {
      # "bound to \n\"DeGaussing Needle\"\nshared global variable"
      # "Bound to \n\"DeGauss Round Num\""
      # "Bound to \"DeGauss Total\""
      n38 = shared-variable "NI-GenericDesktopPC-3A84958E\\Kopco PS Project Target Variables Library.lvlib\\DeGauss Total"("1. Number of rounds") -> ()  [unwired: 1 in, 1 out]
      n39 = for {
        N: "1. Number of rounds" -> [_]
        i -> [w143]
        # "Wait half a second\nbetween repititions \nto allow the system \nto stabilize\n\nAdded by WIM on \n12/18/2017\n\nUpdated to 2 Seconds\nfrom 500 ms"
        # "First Index is 0"
        n40 = Add(x=1, y=w143) -> (x+y=w137:i32)
        n41 = shared-variable "NI-GenericDesktopPC-3A84958E\\Kopco PS Project Target Variables Library.lvlib\\DeGauss Round Num"(w137) -> ()  [unwired: 1 in, 1 out]
        n42 = Wait (ms)(milliseconds to wait=u32 2000) -> ()  [unwired: 1 out]
        n43 = flat-sequence {
          tunnel: [w155] -> w152
          tunnel: [w153] -> w151
          tunnel: w137 -> [w154]
          tunnel: [w154] -> w140
          tunnel: w152 -> [w177]
          tunnel: [w184] -> w150
          tunnel: [w176] -> w149
          tunnel: [w190] -> w148
          tunnel: w151 -> [w175]
          tunnel: [w175] -> w147
          tunnel: w140 -> [w174]
          tunnel: [w174] -> w139
          tunnel: w150 -> [w207]
          tunnel: w149 -> [w208]
          tunnel: w148 -> [w215]
          tunnel: [w214] -> w146
          tunnel: [w213] -> w145
          tunnel: [w212] -> w144
          tunnel: w147 -> [w205]
          tunnel: w139 -> [w203]
          tunnel: [w203] -> w138
          tunnel: w146 -> [w250]
          tunnel: w145 -> [w249]
          tunnel: w144 -> [w245]
          tunnel: w138 -> [_]
          frame #0 {
            w156 = 5  # Time in Seconds
            w155 = 6000  # Sampling Rate (Samples/Seconds)
            # "Step 0 DeGaussing"
            # "Hardware-Time control loop cannot keep up\nwith 50,000 Hz frequence."
            n44 = Multiply(x=w156, y=w155) -> (x*y=w157:i32)
            n45 = for "A Single DeGuassing Waveform" {
              N: w157 -> [_]
              tunnel: w155 -> [w161]
              tunnel: [w158] -> w153 mode=indexing
              i -> [w160]
              (unwired) 0.3 ("y")
              w164 = 1.0  # A_0
              w167 = 1.0  # Lambda
              w171 = 0.0  # No phase
              w172 = 60.0  # Frequency, 60 Hz
              w173 = 10.0  # 4 amps = 10V
              # "Minimized 10 V to 5 V on 3/19/2018\nadd an offset of 0.3V for now"
              # "Lambda = ln(2)/(halflife time)^2"
              n46 = To Double Precision Float(number=w160) -> (double precision float=w162:dbl)
              n47 = Divide "dT"(x=w162, y=w161) -> (x/y=w159:dbl)
              n48 = Square(x=w159) -> (x^2=w165:dbl)
              n49 = Negate(x=w165) -> (-x=w166:dbl)
              n50 = call <vilib>:"Sine Wave PtByPt.vi"("time"=w159, "phase"=w171, "frequency"=w172, "amplitude"=w173) -> ("sine wave"=w170:dbl)
              n51 = Divide(x=w166, y=w167) -> (x/y=w168:dbl)
              n52 = Exponential(1:w168) -> (0:w169:dbl)
              n53 = Multiply(x=w169, y=w164) -> (x*y=w163:dbl)
              n54 = Multiply(x=w170, y=w163) -> (x*y=w158:dbl)
            }
          }
          frame #1 {
            w185 = -1 items=["default"=-1, "RSE"=10083, "NRSE"=10078, "Differential"=10106, "Pseudodifferential"=12529] ("Terminal Configuration")
            w191 = 12522 items=["Finite Samples"=10178, "Continuous Samples"=10123, "Hardware Timed Single Point"=12522]  # Sample Mode
            w198 = 10106 items=["default"=-1, "RSE"=10083, "NRSE"=10078, "Differential"=10106, "Pseudodifferential"=12529] ("Terminal Configuration")
            w201 = 12522 items=["Finite Samples"=10178, "Continuous Samples"=10123, "Hardware Timed Single Point"=12522]  # Sample Mode
            # "Step 0 DeGaussing"
            # "Power Supply Control"
            # "Magnetic Flux Sensor Signals\nOnly initiated to control \ndeterministic loop"
            n55 = call-poly <vilib>:"DAQmx Create Virtual Channel.vi"("maximum value"=5.0 ("Max Voltage"), "minimum value"=0.0 ("Min Voltage"), "input terminal configuration"=w198, "physical channels"="Dev2/ai5") -> ("task out"=w199:refnum<k21>, "error out"=w200:errorcluster)  [unwired: 10 in]
            n56 = call-poly <vilib>:"DAQmx Create Virtual Channel.vi"("maximum value"=10.0, "minimum value"=-10.0, "output terminal configuration"=w185, "physical channels"="Dev2/ao0") -> ("task out"=w195:refnum<k21>, "error out"=w194:errorcluster)  [unwired: 10 in]
            n57 = call-poly <vilib>:"DAQmx Timing.vi"("task/channels in"=w199, "sample mode"=w201, "rate"=w177, "error in"=w200) -> ("task out"=w188:refnum<k21>, "error out"=w183:errorcluster)  [unwired: 10 in]
            n58 = call "Get Terminal Name with Device Prefix.vi"("error in"=w183, "Local Terminal Name"="ai/SampleClock", "task/channels in"=w188) -> ("error out"=w182:errorcluster, "Terminal Name with Device Prefix"=w181:tag, "task out"=w184:refnum<k21>)  [unwired: 6 in]
            n59 = call-poly <vilib>:"DAQmx Timing.vi"("task/channels in"=w195, "sample mode"=w191, "rate"=w177, "source"=w181, "error in"=w194) -> ("task out"=w178:refnum<k21>, "error out"=w179:errorcluster)  [unwired: 9 in]
            n60 = call <vilib>:"DAQmx Start Task.vi"("task/channels in"=w178, "error in"=w179) -> ("task out"=w190:refnum<k21>, "error out"=w189:errorcluster)  [unwired: 12 in]
            n61 = Merge Errors(w182, w189) -> (w176:errorcluster)
          }
          frame #2 {
            # "Step 0 DeGaussing"
            n62 = call-poly <vilib>:"DAQmx Create Timing Source.vi"("task/channels in"=w207, "sleep time (us)"=1.0, "error in"=w208) -> ("task out"=w204:refnum<k21>, "timing source out"=w206:string, "error out"=w202:errorcluster)  [unwired: 10 in]
            n63 = node-c288(w206, w202) -> (w211:T3)  [unwired: 8 in]
            n64 = timed-loop "DeGuassing Control" {
              tunnel: w204 -> [w234]
              tunnel: [w227] -> w213
              tunnel: w215 -> [w217]
              tunnel: [w232] -> w212
              tunnel: w202 -> [w231]
              tunnel: [w230] -> w214
              timing: w211 -> [_]
              timing-out: [_] -> w210
              tunnel: w205 -> [w219]
              i -> [w223]
              stop <- w216 continue-if-true
              # "PS does not turn off unless two values are written."
              # "Offset by 1 to eliminate\nextra datapoint at end"
              n65 = node-c288() -> ()  [unwired: 1 in, 1 out]
              n66 = Array Size(array=w219) -> (size(s)=w224:i32)
              n67 = Index Array "Index Array"(array=w219, index=w223) -> (element=w220:dbl)
              n68 = call-poly <vilib>:"DAQmx Read.vi"("task/channels in"=w234, "error in"=w231) -> ("task out"=w227:refnum<k21>, "error out"=w233:errorcluster)  [unwired: 11 in, 1 out]
              n69 = Less?(x=w223, y=w224) -> (x < y?=w222:bool)
              n70 = Subtract(x=w224, y=10) -> (x-y=w226:i32)
              n71 = Less?(x=w223, y=w226) -> (x < y?=w221:bool)
              n72 = case shown="True" w221 {
                tunnel: [0.0 ("output") w237] -> w218
                tunnel: w220 -> [_ w237]
                frame False {
                  # "Zero the AO at the end"
                }
                frame True {
                }
              }
              n73 = call-poly <vilib>:"DAQmx Write.vi"("task/channels in"=w217, "data"=w218, "error in"=w233) -> ("task out"=w232:refnum<k21>, "error out"=w230:errorcluster)  [unwired: 10 in, 1 out]
              n74 = Unbundle By Name(w230) -> ("status"=w235:bool)  [unwired: 2 out]
              n75 = Not Or(1:FALSE ("Stop"), 2:w235) -> (0:w228:bool)
              n76 = And(x=w228, y=w222) -> (x .and. y?=w216:bool)
              n77 = shared-variable "NI-GenericDesktopPC-3A84958E\\Kopco PS Project Target Variables Library.lvlib\\DeGuassing Needle"(w216) -> ()  [unwired: 1 in, 1 out]
              n78 = node-c288() -> ()  [unwired: 1 in, 1 out]
            }
            n79 = node-c288(w210) -> ()  [unwired: 1 out]
          }
          frame #3 {
            n80 = call <vilib>:"DAQmx Stop Task.vi"("task/channels in"=w249, "error in"=w250) -> ("task out"=w252:refnum<k21>, "error out"=w251:errorcluster)  [unwired: 12 in]
            n81 = call <vilib>:"DAQmx Clear Task.vi"("task in"=w252, "error in"=w251) -> ("error out"=w246:errorcluster)  [unwired: 13 in]
            n82 = call <vilib>:"DAQmx Stop Task.vi"("task/channels in"=w245, "error in"=w246) -> ("task out"=w248:refnum<k21>, "error out"=w247:errorcluster)  [unwired: 12 in]
            n83 = call <vilib>:"DAQmx Clear Task.vi"("task in"=w248, "error in"=w247) -> ()  [unwired: 13 in, 1 out]
          }
        }
      }
    }
    frame #4 {
      # "Step 0 Reset the Magnetic Sensor"
      n84 = case shown="True" "Measure Flux Sensor Zero?" {
        frame False {
        }
        frame True {
          w261 = 12522 items=["Finite Samples"=10178, "Continuous Samples"=10123, "Hardware Timed Single Point"=12522] ("sample mode")
          w275 = 3.0  # Time (s)
          w274 = 10000  # Samples read  per loop
          w294 = -1 items=["default"=-1, "RSE"=10083, "NRSE"=10078, "Differential"=10106, "Pseudodifferential"=12529] ("Terminal Configuration")
          w291 = 12522 items=["Finite Samples"=10178, "Continuous Samples"=10123, "Hardware Timed Single Point"=12522]  # Sample Mode
          w283 = 10106 items=["Default"=-1, "RSE"=10083, "NRSE"=10078, "Differential"=10106, "Pseudodifferential"=12529]  # input terminal configuration
          w286 = 0
          # "Changed on 3/29/2018 to include Sensor 2 placed in front of the needle. Added Global Variable \"Flux Calibrated Zero 2\""
          # "Reset AO to 0. Sometimes it overshoot after DeGaussing\nAdded by #WIM on 12/18/2017"
          # "Power Supply Control"
          n85 = shared-variable "NI-GenericDesktopPC-3A84958E\\Kopco PS Project Target Variables Library.lvlib\\Channels AI List"() -> (w277:string)  [unwired: 1 in, 1 out]
          n86 = shared-variable "NI-GenericDesktopPC-3A84958E\\Kopco PS Project Target Variables Library.lvlib\\Sampling Rate"() -> (w256:dbl)  [unwired: 1 in, 1 out]
          n87 = call-poly <vilib>:"DAQmx Create Virtual Channel.vi"("maximum value"=5.0, "minimum value"=0.0, "input terminal configuration"=w283, "physical channels"=w277) -> ("task out"=w257:refnum<k21>, "error out"=w258:errorcluster)  [unwired: 10 in]
          n88 = call-poly <vilib>:"DAQmx Create Virtual Channel.vi"("maximum value"=10.0, "minimum value"=-10.0, "output terminal configuration"=w294, "physical channels"="Dev2/ao0") -> ("task out"=w288:refnum<k21>, "error out"=w289:errorcluster)  [unwired: 10 in]
          n89 = call-poly <vilib>:"DAQmx Timing.vi"("task/channels in"=w257, "sample mode"=w261, "rate"=w256, "error in"=w258) -> ("task out"=w260:refnum<k21>, "error out"=w259:errorcluster)  [unwired: 10 in]
          n90 = Multiply "Total Samples \nper Channel"(x=w256, y=w275) -> (x*y=w276:dbl)
          n91 = call "Get Terminal Name with Device Prefix.vi"("error in"=w259, "Local Terminal Name"="ai/SampleClock", "task/channels in"=w260) -> ("error out"=w271:errorcluster, "Terminal Name with Device Prefix"=w270:tag, "task out"=w266:refnum<k21>)  [unwired: 6 in]
          n92 = call-poly <vilib>:"DAQmx Timing.vi"("task/channels in"=w288, "sample mode"=w291, "rate"=w256, "source"=w270, "error in"=w289) -> ("task out"=w296:refnum<k21>, "error out"=w295:errorcluster)  [unwired: 9 in]
          n93 = call <vilib>:"DAQmx Start Task.vi"("task/channels in"=w296, "error in"=w295) -> ("task out"=w299:refnum<k21>, "error out"=w298:errorcluster)  [unwired: 12 in]
          n94 = Merge Errors(w271, w298) -> (w264:errorcluster)
          n95 = Subtract "Almost Total"(x=w276, y=w274) -> (x-y=w273:dbl)
          n96 = shared-variable "NI-GenericDesktopPC-3A84958E\\Kopco PS Project Target Variables Library.lvlib\\Sensor Index Flux Core"() -> (w255:i8)  [unwired: 1 in, 1 out]
          n97 = call-poly <vilib>:"DAQmx Create Timing Source.vi"("task/channels in"=w266, "sleep time (us)"=1.0, "error in"=w264) -> ("task out"=w267:refnum<k21>, "timing source out"=w262:string, "error out"=w265:errorcluster)  [unwired: 10 in]
          n98 = Initialize Array(w286, w286) -> (w279:i32[])
          n99 = node-c288(w262) -> (w269:T3)  [unwired: 3 in]
          n100 = timed-loop {
            tunnel: w267 -> [w320]
            tunnel: w265 -> [w315]
            tunnel: [w321] -> w303
            shift-right: [w322] -> _
            shift-left: 0 -> [w323]
            tunnel: [w319] -> w297
            shift-right: [w317] -> w254
            shift-left: w279 -> [w312]
            tunnel: [w312] -> _
            tunnel: w299 -> [w316]
            tunnel: [w311] -> w304
            tunnel: w274 -> [w309]
            tunnel: w273 -> [w308]
            timing: w269 -> [_]
            timing-out: [_] -> w268
            shift-right: [w307] -> _
            shift-left: _ -> [_]
            tunnel: w255 -> [w305]
            i -> [w307]
            stop <- w306 continue-if-true
            w324 = 10.0  # timeout
            # "Magnetic Sensor 2"
            # "Magnetic Sensor 1"
            n101 = node-c288() -> ()  [unwired: 1 in, 1 out]
            n102 = call-poly <vilib>:"DAQmx Write.vi"("task/channels in"=w316, "data"=0.0, "error in"=w315) -> ("task out"=w311:refnum<k21>, "error out"=w314:errorcluster)  [unwired: 10 in, 1 out]
            n103 = call-poly <vilib>:"DAQmx Read.vi"("task/channels in"=w320, "number of samples per channel"=w309, "timeout"=w324, "error in"=w314) -> ("task out"=w319:refnum<k21>, "data"=w310:dbl[][], "error out"=w321:errorcluster)  [unwired: 9 in]
            n104 = Add(x=w323, y=w309) -> (x+y=w322:i32)
            n105 = Unbundle By Name(w321) -> ()  [unwired: 1 out]
            n106 = Less Or Equal?(x=w322, y=w308) -> (x <= y?=w306:bool)
            n107 = Delete From Array(array=w310, index (row)=w305) -> (deleted portion=w318:dbl[])  [unwired: 2 in, 1 out]
            n108 = shared-variable "NI-GenericDesktopPC-3A84958E\\Kopco PS Project Target Variables Library.lvlib\\Sensor Zero Calibrating"(w306) -> ()  [unwired: 1 in, 1 out]
            n109 = Build Array (concatenate)(w312, w318) -> (w317:dbl[])
            n110 = node-c288() -> ()  [unwired: 1 in, 1 out]
          }
          "Waveform Graph 2" <- w254
          n111 = node-c288(w268) -> ()  [unwired: 1 out]
          n112 = call <vilib>:"Std Deviation and Variance.vi"("X"=w254) -> ("mean"=w280:dbl)  [unwired: 1 in, 2 out]
          n113 = call <vilib>:"DAQmx Stop Task.vi"("task/channels in"=w304, "error in"=w303) -> ("task out"=w300:refnum<k21>, "error out"=w301:errorcluster)  [unwired: 12 in]
          n114 = shared-variable "NI-GenericDesktopPC-3A84958E\\Kopco PS Project Target Variables Library.lvlib\\Zero Flux Calibrated Core"(w280) -> ()  [unwired: 1 in, 1 out]
          n115 = call <vilib>:"DAQmx Clear Task.vi"("task in"=w300, "error in"=w301) -> ("error out"=w302:errorcluster)  [unwired: 13 in]
          n116 = call <vilib>:"DAQmx Stop Task.vi"("task/channels in"=w297, "error in"=w302) -> ("task out"=w285:refnum<k21>, "error out"=w284:errorcluster)  [unwired: 12 in]
          n117 = call <vilib>:"DAQmx Clear Task.vi"("task in"=w285, "error in"=w284) -> ("error out"=w278:errorcluster)  [unwired: 13 in]
          n118 = call <vilib>:"General Error Handler.vi"("error in (no error)"=w278) -> ()  [unwired: 10 in, 5 out]
        }
      }
    }
    frame #5 {
      # "Bound to \"Flux Calibrated Zero 2\" \nglobal Variable"
      # "Bound to \"Flux Calibrated Zero\" \nglobal Variable"
      # "Bound to \"DeGaussing Finished\""
      # "Ensure that the correct value is displayed\n(2.49±0.05 (V))"
      n119 = shared-variable "NI-GenericDesktopPC-3A84958E\\Kopco PS Project Target Variables Library.lvlib\\DeGuassing Finished"(TRUE ("DeGuassing Finished")) -> ()  [unwired: 1 in, 1 out]
    }
    frame #6 {
      # "Bound to \"Needle Selection Finished\" \nshared global variable."
      # "Step 1 Selecting Needle & Sensor\n& PID Parameters"
      n120 = while {
        tunnel: ["Proceed with Selection"] -> w336
        tunnel: ["2. Needle:"] -> w335
        tunnel: ["1. Sensor:"] -> w334
        tunnel: ["3. PID Parameters:"] -> w333
        tunnel: ["4. Aggressiveness:"] -> w332
        stop <- "Proceed with Selection" stop-if-true
        # "Added on 1/16/2018"
      }
      n121 = shared-variable "NI-GenericDesktopPC-3A84958E\\Kopco PS Project Target Variables Library.lvlib\\Needle Selection Finished"(w336) -> ()  [unwired: 1 in, 1 out]
    }
    frame #7 {
      # "Step 1 Selecting Needle & Sensor\n& PID Parameters"
      # "1/5/2018\nGot rid of \"normal\" PID Gains, Only kept Aggressive..\n\nFrom now on, that name will be dropped."
      # "Needle Used no needed so far\nbut might be used in future versinos\n12/20/2017"
      # "More precisely measured Magnetic Sensor value for Sensors 1 & 2 on 11/28/2017"
      # "Older Magnetic Sensitivity Measured before 11/2017 for Sensor 2 very crudely\n0.003112 V/GS.\nPreviously sensor 2 zero was 2.4942892 V based on 10-minute experiments on 7/12/2017"
      # "Coupled with Shared Variable Sensor 1"
      n122 = case shown="1" w345 {
        tunnel: [T1 {"proportional gain (Kc)"=0.051, "integral time (Ti, min)"=3.5e-06, "derivative time (Td, min)"=0.0} ("PID gains HyMu80 #1 (Aggressive)") T1 {"proportional gain (Kc)"=0.051, "integral time (Ti, min)"=3.5e-06, "derivative time (Td, min)"=0.0} ("PID gains HyMu80 #2 (Aggressive)")] -> w347
        tunnel: [i8 1 ("Needle Used") i8 2 ("Needle Used")] -> w348
        frame 0, Default {
          # "HyMu80#1 (Aggressive) Parameters\nModified from 0.08 to 0.075 on 4/2/2018"
          # "D"
          # "I"
          # "P"
        }
        frame 1 {
          # "D"
          # "I"
          # "P"
        }
      }
      n123 = case shown="1" w344 {
        tunnel: [0.0029794 0.0030418] -> w346
        frame 0, Default {
          (unwired) 2.4837669
          # "Zero = 2.4837669 V"
          # "Sensor #1"
          # "Sensitivity = 2.9794 mV/GS"
        }
        frame 1 {
          (unwired) 2.4928421
          # "Zero = 2.4928421 V"
          # "Sensor #2"
          # "Sensor 2 = 3.0418 mV/GS"
        }
      }
      n124 = shared-variable "NI-GenericDesktopPC-3A84958E\\Kopco PS Project Target Variables Library.lvlib\\Sensor Sensitivity Core"(w346) -> ()  [unwired: 1 in, 1 out]
      n125 = shared-variable "NI-GenericDesktopPC-3A84958E\\Kopco PS Project Target Variables Library.lvlib\\Needle Used"(w348) -> ()  [unwired: 1 in, 1 out]
    }
    frame #8 {
      (unwired) "1. SET-UP & RUN \"LIVE-FAST\" image acquisition in Nikon Elements. \n2. POSITION the magnetic needle in the glycerol sample within 100 micron of several beads. (Please refer to latest calibration protocol for more details). \n3. Click OK then follow the Steps 3:\n      1. CLICK \"Start Null Flux Adjustment.\"\n      2. Adjust the Magnetic Flux until beads are no longer attacted to the needle.\n      3. Select if you want the flux to stay running until the control sequence is used in Step 4\n      3. CLICK \"FINISH Null Flux Adjustment?\" to Move to Step 4 \n"  # 1. SET-UP & RUN "LIVE-FAST" image acquisition in Nikon Elements.  2. POSITION the magnetic needle in the glycerol sample within 100 micron of several beads. (Please refer to latest calibration protocol for more details).  3. Click OK then follow the Steps 3:       1. CLICK "Start Null Flux Adjustment."       2. Adjust the Magnetic Flux until beads are no longer attacted to the needle.       3. Select if you want the flux to stay running until the control sequence is used in Step 4       3. CLICK "FINISH Null Flux Adjustment?" to Move to Step 4
    }
    frame #9 {
      # "Bound to \"Flux RT Control\" \nglobal shared variable?"
      # "Step 2 Finding Null Flux in Real Time"
      n126 = while {
        tunnel: ["Start Null Flux Adjustment"] -> w362
        tunnel: [w364] -> w360
        tunnel: w361 -> [w364]
        stop <- "Start Null Flux Adjustment" stop-if-true
      }
      n127 = shared-variable "NI-GenericDesktopPC-3A84958E\\Kopco PS Project Target Variables Library.lvlib\\Flux RT Control"(w362) -> ()  [unwired: 1 in, 1 out]
    }
    frame #10 {
      w379 = -1 items=["default"=-1, "RSE"=10083, "NRSE"=10078, "Differential"=10106, "Pseudodifferential"=12529] ("Terminal Configuration")
      w384 = 12522 items=["Finite Samples"=10178, "Continuous Samples"=10123, "Hardware Timed Single Point"=12522]  # Sample Mode
      w390 = 10106 items=["default"=-1, "RSE"=10083, "NRSE"=10078, "Differential"=10106, "Pseudodifferential"=12529] ("Terminal Configuration")
      w393 = 12522 items=["Finite Samples"=10178, "Continuous Samples"=10123, "Hardware Timed Single Point"=12522]  # Sample Mode
      # "Step 2 Finding Null Flux in Real Time"
      # "Hardware-Time control loop cannot keep up\nwith 50,000 Hz frequence."
      # "Power Supply Control"
      # "Magnetic Flux Sensor Signals\nRelayed over three channels."
      n128 = shared-variable "NI-GenericDesktopPC-3A84958E\\Kopco PS Project Target Variables Library.lvlib\\Channels AI List"() -> (w365:string)  [unwired: 1 in, 1 out]
      n129 = shared-variable "NI-GenericDesktopPC-3A84958E\\Kopco PS Project Target Variables Library.lvlib\\Sampling Rate"() -> (w366:dbl)  [unwired: 1 in, 1 out]
      n130 = call-poly <vilib>:"DAQmx Create Virtual Channel.vi"("maximum value"=5.0 ("Max Voltage"), "minimum value"=0.0 ("Min Voltage"), "input terminal configuration"=w390, "physical channels"=w365) -> ("task out"=w391:refnum<k21>, "error out"=w392:errorcluster)  [unwired: 10 in]
      n131 = call-poly <vilib>:"DAQmx Create Virtual Channel.vi"("maximum value"=10.0, "minimum value"=-10.0, "output terminal configuration"=w379, "physical channels"="Dev2/ao0") -> ("task out"=w387:refnum<k21>, "error out"=w386:errorcluster)  [unwired: 10 in]
      n132 = call-poly <vilib>:"DAQmx Timing.vi"("task/channels in"=w391, "sample mode"=w393, "rate"=w366, "error in"=w392) -> ("task out"=w382:refnum<k21>, "error out"=w378:errorcluster)  [unwired: 10 in]
      n133 = call "Get Terminal Name with Device Prefix.vi"("error in"=w378, "Local Terminal Name"="ai/SampleClock", "task/channels in"=w382) -> ("error out"=w375:errorcluster, "Terminal Name with Device Prefix"=w377:tag, "task out"=w372:refnum<k21>)  [unwired: 6 in]
      n134 = call-poly <vilib>:"DAQmx Timing.vi"("task/channels in"=w387, "sample mode"=w384, "rate"=w366, "source"=w377, "error in"=w386) -> ("task out"=w374:refnum<k21>, "error out"=w373:errorcluster)  [unwired: 9 in]
      n135 = call <vilib>:"DAQmx Start Task.vi"("task/channels in"=w374, "error in"=w373) -> ("task out"=w370:refnum<k21>, "error out"=w383:errorcluster)  [unwired: 12 in]
      n136 = Merge Errors(w375, w383) -> (w371:errorcluster)
    }
    frame #11 {
      w406 = 30  # # of samples pushed to PID loop
      # "Bound to \"Null Flux Running Middle\" \nshared global variable."
      # "Bound to \"Null Flux Selected\"\nshared global variable"
      # "Step 2 Finding Null Flux in Real Time"
      # "Step 2 Finding Null Flux in Real Time"
      # "12/13/2017. Cannot turn on flux control sequence inside Real-time loop. That is why I have used the trigger in the Datalogger to turn th is on. \nOtherwise, it will remain off"
      # "PID is 30 times slower"
      n137 = shared-variable "NI-GenericDesktopPC-3A84958E\\Kopco PS Project Target Variables Library.lvlib\\Zero Flux Calibrated Core"() -> (w402:dbl)  [unwired: 1 in, 1 out]
      n138 = shared-variable "NI-GenericDesktopPC-3A84958E\\Kopco PS Project Target Variables Library.lvlib\\Sensor Sensitivity Core"() -> (w400:dbl)  [unwired: 1 in, 1 out]
      n139 = call-poly <vilib>:"DAQmx Create Timing Source.vi"("task/channels in"=w414, "sleep time (us)"=1.0, "error in"=w413) -> ("task out"=w420:refnum<k21>, "timing source out"=w417:string, "error out"=w418:errorcluster)  [unwired: 10 in]
      n140 = shared-variable "NI-GenericDesktopPC-3A84958E\\Kopco PS Project Target Variables Library.lvlib\\Sensor Index Flux Core"() -> (w395:i8)  [unwired: 1 in, 1 out]
      n141 = Reciprocal(x=w398) -> (1/x=w408:dbl)
      n142 = Multiply(x=w406, y=w408) -> (x*y=w407:dbl)
      n143 = Initialize Array "Initialize Array"(0, 0 ("level 3 duration 0.1ms")) -> (w415:i32[])
      n144 = node-c288(w417, w418) -> (w424:T3)  [unwired: 8 in]
      n145 = timed-loop {
        tunnel: w420 -> [w454]
        tunnel: [w449] -> w411
        tunnel: w412 -> [w453]
        tunnel: [w451] -> w410
        tunnel: w418 -> [w450]
        tunnel: [w440] -> w409
        timing: w424 -> [_]
        timing-out: [_] -> w423
        shift-right: [w437] -> _
        shift-left: 0 -> [w446]
        shift-right: [w443] -> _
        shift-left: w415 -> [w444]
        tunnel: w406 -> [w435]
        tunnel: w407 -> [w434]
        tunnel: w402 -> [w433]
        tunnel: w400 -> [w432]
        tunnel: ["2. Adjust Magnetic Flux (GS):"] -> w394
        tunnel: [w431] -> _
        tunnel: [w431] -> w405
        tunnel: [w430] -> w404
        tunnel: w401 -> [w429]
        tunnel: [w428] -> w396
        tunnel: w395 -> [w427]
        stop <- w431 continue-if-true
        # "Observed Flux (V)"
        # "Keep this control inside the loop so that changed in \nreal time under live imaging"
        # "Flux Sensor Calibrated Zero value (V)"
        n146 = node-c288() -> ()  [unwired: 1 in, 1 out]
        n147 = call-poly <vilib>:"DAQmx Read.vi"("task/channels in"=w454, "error in"=w450) -> ("task out"=w449:refnum<k21>, "data"=w441:dbl[], "error out"=w452:errorcluster)  [unwired: 11 in]
        n148 = Delete From Array "Choose 1st Channel"(array=w441, index=w427) -> (deleted portion=w445:dbl)  [unwired: 1 in, 1 out]
        n149 = Build Array (concatenate) "AI Array"(w445, w444) -> (w442:dbl[])
        n150 = Array Size(array=w442) -> (size(s)=w448:i32)
        n151 = Equal?(x=w448, y=w435) -> (x = y?=w447:bool)
        n152 = Multiply(x="2. Adjust Magnetic Flux (GS):", y=w432) -> (x*y=w436:dbl)
        n153 = Add "Zero Offset"(x=w433, y=w436) -> (x+y=w439:dbl)
        n154 = case shown="True" w447 {
          tunnel: w434 -> [_ w467]
          tunnel: w439 -> [_ w472]
          tunnel: [w465 w470] -> w437
          tunnel: w446 -> [w465 _]
          tunnel: w442 -> [w464 w469]
          tunnel: [w464 w468] -> w443
          tunnel: w429 -> [_ w466]
          frame False {
          }
          frame True {
            # "Max/Min controller outputs"
            n155 = call-poly <vilib>:"Mean.vi"("X"=w469) -> ("mean"=w471:dbl)  [unwired: 1 out]
            n156 = call-poly <vilib>:"PID.vi"("reinitialize? (F)"=FALSE, "output range"=cluster{"output high":dbl, "output low":dbl} {"output high"=10.0, "output low"=-10.0}, "dt (s)"=w467, "PID gains"=w466, "process variable"=w471, "setpoint"=w472) -> ("output"=w470:dbl)  [unwired: 4 in, 1 out]
            n157 = Initialize Array(0, 0) -> (w468:i32[])
          }
        }
        n158 = case shown="True" "4. Click Rocker to finish Null Flux Adjustment" {
          tunnel: [w456 TRUE ("y")] -> w438
          tunnel: [w457 w459] -> w428
          tunnel: w437 -> [w457 w460]
          tunnel: [w456 "3. Keep Null Flux Running \n       Until Next Step?"] -> w430
          frame False {
            w456 = FALSE ("y")
          }
          frame True {
            # "A Toggle fixed the problem!"
            n159 = case shown="True" "3. Keep Null Flux Running \n       Until Next Step?" {
              tunnel: [0.0 ("output") w463] -> w459
              tunnel: w460 -> [_ w463]
              frame False {
                # "Reset AO at the end"
              }
              frame True {
                # "Keep Flux the same"
              }
            }
          }
        }
        n160 = call-poly <vilib>:"DAQmx Write.vi"("task/channels in"=w453, "data"=w428, "error in"=w452) -> ("task out"=w451:refnum<k21>, "error out"=w440:errorcluster)  [unwired: 10 in, 1 out]
        n161 = Unbundle By Name(w440) -> ("status"=w455:bool)  [unwired: 2 out]
        n162 = Not Or(1:w438, 2:w455) -> (0:w431:bool)
        n163 = node-c288() -> ()  [unwired: 1 in, 1 out]
      }
      n164 = Not(x=w405) -> (.not. x?=w403:bool)
      n165 = node-c288(w423) -> ()  [unwired: 1 out]
      n166 = shared-variable "NI-GenericDesktopPC-3A84958E\\Kopco PS Project Target Variables Library.lvlib\\Null Flux Running Middle"(w404) -> ()  [unwired: 1 in, 1 out]
      n167 = shared-variable "NI-GenericDesktopPC-3A84958E\\Kopco PS Project Target Variables Library.lvlib\\Null Flux Selected"(w403) -> ()  [unwired: 1 in, 1 out]
      n168 = shared-variable "NI-GenericDesktopPC-3A84958E\\Kopco PS Project Target Variables Library.lvlib\\Flux RT Control"(w405) -> ()  [unwired: 1 in, 1 out]
    }
    frame #12 {
      # "Zeroing the PS Output at the end with a STOP botton.\nReplacing it with a Toggle seemed to do the trick.\n \nSwitch the toggle \"mechanical action\" to \n\"Latch when Released\" so that it will reset to FALSE \nat the end every time."
      n169 = call <vilib>:"DAQmx Stop Task.vi"("task/channels in"=w490, "error in"=w488) -> ("task out"=w495:refnum<k21>, "error out"=w494:errorcluster)  [unwired: 12 in]
      n170 = call <vilib>:"DAQmx Clear Task.vi"("task in"=w495, "error in"=w494) -> ("error out"=w491:errorcluster)  [unwired: 13 in]
      n171 = call <vilib>:"DAQmx Stop Task.vi"("task/channels in"=w489, "error in"=w491) -> ("task out"=w493:refnum<k21>, "error out"=w492:errorcluster)  [unwired: 12 in]
      n172 = call <vilib>:"DAQmx Clear Task.vi"("task in"=w493, "error in"=w492) -> ()  [unwired: 13 in, 1 out]
    }
    frame #13 {
      (unwired) "OK!"
      (unwired) "1. REMOVE the needle from the sample (if needed).\n2. PREPARE for the next experiment.\n3. Click OK in this dialog box!\n4. ENTER the required variables here: (Flux Setpoint & Number of Cycles, & Length of Pre-and Post-Periods of Null Flux). Click \"Proceed with these Parameters.\"\n5. OPEN Data Logger (if you have not done so), ENTER file name, and RUN program. \n6. ADJUST the number of frames in the Fast Timelapse Macro (if a macro is used). Otherwise, skip this step. \n7. RUN the macro (if a macro is used). Otherwise, click \"TRGR\" button in Nikon Elements to initiate Fast Timelapse Image Capture, Data Acquisition, and PID-Controlled Sequence.\n"  # 1. REMOVE the needle from the sample (if needed). 2. PREPARE for the next experiment. 3. Click OK in this dialog box! 4. ENTER the required variables here: (Flux Setpoint & Number of Cycles, & Length of Pre-and Post-Periods of Null Flux). Click "Proceed with these Parameters." 5. OPEN Data Logger (if you have not done so), ENTER file name, and RUN program.  6. ADJUST the number of frames in the Fast Timelapse Macro (if a macro is used). Otherwise, skip this step.  7. RUN the macro (if a macro is used). Otherwise, click "TRGR" button in Nikon Elements to initiate Fast Timelapse Image Capture, Data Acquisition, and PID-Controlled Sequence.
      # "AO values of current"
      n173 = shared-variable "NI-GenericDesktopPC-3A84958E\\Kopco PS Project Target Variables Library.lvlib\\Zero Flux Observed GS"(w496) -> ()  [unwired: 1 in, 1 out]
    }
    frame #14 {
      # "AO values of current"
      # "Bound to \"PID Parameters Selected\"\nshared global variable"
      # "Step 3 Specifying Waveform Parameters"
      # "Step 3 Specifying Waveform Parameters"
      n174 = while {
        tunnel: ["Proceed with Parameters"] -> w511
        tunnel: ["Flux ON relative setpoint (Gs)"] -> w510
        tunnel: [w515] -> w509
        tunnel: ["Number of Cycles"] -> w508
        tunnel: ["Pre-Wave Null Flux Interval (s)"] -> w507
        tunnel: ["Post-Wave Null Flux Interval (s)"] -> w506
        tunnel: ["2nd to last\n OFF (s)"] -> w502
        tunnel: ["ON"] -> w501
        tunnel: [w512] -> w500
        stop <- "Proceed with Parameters" stop-if-true
        # "Updated code on \nto vary ON/OFF cycle"
        # "You can use a #negative #sign to go to the opposite end\nto extend the linear range if neeed."
        # "Changed Cycles type from double\nto integer-16bit on 1/8/2018"
        # "Global variables were moved inside this while loop to resolve\nthe problem of updating them. For whatever reason, LabVIEW\nseems to only pass to the variable the previous values but \nnot the updated ones for variable (but passes the updated version for \nan indicator). Verified on 1/8/2018 by #WIM"
        n175 = shared-variable "NI-GenericDesktopPC-3A84958E\\Kopco PS Project Target Variables Library.lvlib\\Zero Flux Observed GS"() -> (w512:dbl)  [unwired: 1 in, 1 out]
        n176 = shared-variable "NI-GenericDesktopPC-3A84958E\\Kopco PS Project Target Variables Library.lvlib\\Period OFF 2nd Per Cycle"("2nd to last\n OFF (s)") -> ()  [unwired: 1 in, 1 out]
        n177 = shared-variable "NI-GenericDesktopPC-3A84958E\\Kopco PS Project Target Variables Library.lvlib\\Period ON Per Cycle"("ON") -> ()  [unwired: 1 in, 1 out]
        n178 = shared-variable "NI-GenericDesktopPC-3A84958E\\Kopco PS Project Target Variables Library.lvlib\\Cycles"("Number of Cycles") -> ()  [unwired: 1 in, 1 out]
        n179 = Add "Total Period Time (s)"(x="2nd to last\n OFF (s)", y="ON") -> (x+y=w515:dbl)
        n180 = shared-variable "NI-GenericDesktopPC-3A84958E\\Kopco PS Project Target Variables Library.lvlib\\Flux Setpoint ON Gs Relative"("Flux ON relative setpoint (Gs)") -> ()  [unwired: 1 in, 1 out]
        n181 = shared-variable "NI-GenericDesktopPC-3A84958E\\Kopco PS Project Target Variables Library.lvlib\\Null Flux Post Period"("Post-Wave Null Flux Interval (s)") -> ()  [unwired: 1 in, 1 out]
        n182 = shared-variable "NI-GenericDesktopPC-3A84958E\\Kopco PS Project Target Variables Library.lvlib\\Null Flux Pre Period"("Pre-Wave Null Flux Interval (s)") -> ()  [unwired: 1 in, 1 out]
        n183 = shared-variable "NI-GenericDesktopPC-3A84958E\\Kopco PS Project Target Variables Library.lvlib\\Period Per Cycle"(w515) -> ()  [unwired: 1 in, 1 out]
      }
      n184 = shared-variable "NI-GenericDesktopPC-3A84958E\\Kopco PS Project Target Variables Library.lvlib\\Control Parameters Selected"(w511) -> ()  [unwired: 1 in, 1 out]
    }
    frame #15 {
      w544 = u32 490 ("Ramp Total Interval (ms)")
      w545 = u32 7 ("# Ramp Steps")
      (unwired) 1.0 ("Double")
      w569 = 0 ("index")
      w598 = u32 1000  # ms/sec
      w607 = bool[] []  # Initial Empty Array
      w611 = 747.0  # K_Prime
      w614 = 13.91  # V_max
      w615 = 1.9431  # h
      w650 = dbl[] []  # Initial Zero Array
      w632 = 0.031  # Time Length (s)
      w681 = FALSE
      w663 = bool[] []  # Initial Empty Array
      w692 = dbl[] []  # Initial Zero Array
      # "Post Wave might need to be\nfixed with Ramp"
      # "No need for this"
      # "Number of Cycles"
      # "ON per Cycle (s)"
      # "OFF per Cycle (s)"
      # "Corrected Null Flux/OFF Observed (Gs):\n2nd Cycle OFF & Later & Postwave Corrected"
      # "1/4 wave to get the main points of the\n mini DeGauss waveform 3/12/2018"
      # "AO values of current"
      # "Into the Data Logger"
      # "Null Flux Observed:\n2nd Cycle OFF & Later & Postwave Corrected(V)"
      # "Null Flux Observed:\nPrewave & 1st Cycle OFF Uncorrected (V)\nNO CHANGE!"
      # "Initial Null Flux Observed (Gs)"
      # "5. Based on a sigmoidal curve fit 2019-08-08\nThe Equation is Y = Vmax * X^h /(K_prime + X^h), where Vmax = 13.91, h = 1.9431, and Kprime = 747"
      # "# of samples of Mini DeGauss"
      # "Three choices for mini DeGauss\nwaveform? \n0.030 ms @ 500 Hz   (No AI leakage at \nhigher fluxes ~ 200 Gs. Moreoever, flux\nvariation is higher = more atoms are recruited)\n0.030 ms @ 1000 Hz\n0.015 ms @ 1000 Hz"
      # "Added 3/12/2018"
      # "Amplitude will need to be modified later"
      # "OFF = 2 * 1/2 Cycle - samples of ON Mini DeGauss"
      # "30,000 @ 500 Hz\n\n1000 Hz for PID \nsampling rate of 1 ms\ncreate aliasing/roundoff error\n\nSampling at higher rate, and then\nchoose your points of interest"
      # "OFF = - samples of ON Mini DeGauss"
      # "Period per Cycle (s)"
      # "Flux Setpoint/On (V)"
      # "Flux Relative ON Setpoint (Gs)"
      # "Step 3 Building Waveforms for PID control and for mini-DeGauss Cycles"
      # "Step 3 Creating Waveforms"
      # "1/4/2018. It checks the maximum of either the observed zero or the \nsuperimposed ON setpoints for my OFF/ON square wave"
      # "ON/OFF PID Parameters. In order for this to work, the OFF flux needs to be near the linear range."
      # "Note: Max point is included in that given PID Gain schedule. it is the cut-off point"
      # "I was able to build a PID gain schedule by matching the types.\nThis way I will be able to customize the values based on sensor sensitivities\nand so forth 1/2/2017."
      # "Corrected on 1/4/2018"
      # "N cycles of High/Low\nCreate A Control Array in terms \nof flux sensor voltage"
      n185 = shared-variable "NI-GenericDesktopPC-3A84958E\\Kopco PS Project Target Variables Library.lvlib\\Sampling Rate"() -> (w530:dbl)  [unwired: 1 in, 1 out]
      n186 = To Quad Integer(1:w530) -> (0:w529:i64)
      n187 = Absolute Value(x=w608) -> (abs(x)=w606:dbl)
      n188 = shared-variable "NI-GenericDesktopPC-3A84958E\\Kopco PS Project Target Variables Library.lvlib\\Sensor Sensitivity Core"() -> (w547:dbl)  [unwired: 1 in, 1 out]
      n189 = Divide "ms to sec"(x=w544, y=w598) -> (x/y=w597:dbl)
      n190 = shared-variable "NI-GenericDesktopPC-3A84958E\\Kopco PS Project Target Variables Library.lvlib\\Zero Flux Observed GS"() -> (w592:dbl)  [unwired: 1 in, 1 out]
      n191 = Power Of X "X^h"(1:w606, 2:w615) -> (0:w612:dbl)
      n192 = shared-variable "NI-GenericDesktopPC-3A84958E\\Kopco PS Project Target Variables Library.lvlib\\Ramp Total Interval (ms)"(w544) -> ()  [unwired: 1 in, 1 out]
      n193 = shared-variable "NI-GenericDesktopPC-3A84958E\\Kopco PS Project Target Variables Library.lvlib\\Ramp Steps"(w545) -> ()  [unwired: 1 in, 1 out]
      n194 = Multiply(x=w614, y=w612) -> (x*y=w613:dbl)
      n195 = Add(x=w612, y=w611) -> (x+y=w610:dbl)
      n196 = shared-variable "NI-GenericDesktopPC-3A84958E\\Kopco PS Project Target Variables Library.lvlib\\Flux Setpoint ON Gs Relative"() -> (w579:dbl)  [unwired: 1 in, 1 out]
      n197 = Divide "Shift in Null Flux Observed (Gs)"(x=w613, y=w610) -> (x/y=w609:dbl)
      n198 = shared-variable "NI-GenericDesktopPC-3A84958E\\Kopco PS Project Target Variables Library.lvlib\\Sensor Sensitivity Core"() -> (w548:dbl)  [unwired: 1 in, 1 out]
      n199 = Add "Correcting Null Flux Observed (Gs)"(x=w609, y=w521) -> (x+y=w593:dbl)
      n200 = shared-variable "NI-GenericDesktopPC-3A84958E\\Kopco PS Project Target Variables Library.lvlib\\Zero Flux Observed Gs Corrected"(w593) -> ()  [unwired: 1 in, 1 out]
      n201 = Multiply "# Total ramp\nSamples"(x=w597, y=w529) -> (x*y=w601:dbl)
      n202 = Multiply "# of Samples"(x=w632, y=w529) -> (x*y=w622:dbl)
      n203 = Divide(x=750.0, y=900.0) -> (x/y=w621:dbl)
      n204 = To Unsigned Long Integer(number=w622) -> (unsigned 32bit integer=w616:u32)
      n205 = To Unsigned Long Integer "# total ramp\nsamples (int)"(number=w601) -> (unsigned 32bit integer=w582:u32)
      n206 = Multiply(x=w622, y=w621) -> (x*y=w618:dbl)
      n207 = Subtract "Uncorrected to Corrected\n OFF Shift (Gs)"(x=w593, y=w592) -> (x-y=w580:dbl)
      n208 = for "One Mini DeGauss Cycle" {
        N: w616 -> [_]
        tunnel: w529 -> [w746]
        tunnel: [w762] -> w642 mode=indexing
        tunnel: w632 -> [w747]
        tunnel: [w746] -> w631
        tunnel: [w745] -> w630
        i -> [w761]
        w750 = 7.5  # amplitude
        w752 = 1.0  # Starting Amplitude
        w766 = 90.0  # Phase, Deg
        w745 = u64 480  # Frequency, Hz
        # "It seems 0.3 * Time will give \na decay around 20 ms."
        # "samples/sec"
        n209 = To Double Precision Float(number=w761) -> (double precision float=w763:dbl)
        n210 = Multiply(x=w747, y=0.3) -> (x*y=w748:dbl)
        n211 = Divide(x=w763, y=w746) -> (x/y=w757:dbl)
        n212 = Square(x=w757) -> (x^2=w759:dbl)
        n213 = Square(x=w748) -> (x^2=w755:dbl)
        n214 = Natural Logarithm(1:2.0 ("x")) -> (0:w753:dbl)
        n215 = Divide(x=w753, y=w755) -> (x/y=w754:dbl)
        n216 = Negate(x=w759) -> (-x=w758:dbl)
        n217 = Multiply(x=w758, y=w754) -> (x*y=w764:dbl)
        n218 = call <vilib>:"Sine Wave PtByPt.vi"("time"=w757, "phase"=w766, "frequency"=w745, "amplitude"=w750) -> ("sine wave"=w751:dbl)
        n219 = Exponential "Exp(-t^2*k)"(1:w764) -> (0:w765:dbl)
        n220 = Multiply(x=w765, y=w752) -> (x*y=w760:dbl)
        n221 = Multiply(x=w751, y=w760) -> (x*y=w762:dbl)
      }
      n222 = Increment "Make one extra to trim"(x=w545) -> (x+1=w591:u32)
      n223 = To Unsigned Long Integer(number=w618) -> (unsigned 32bit integer=w617:u32)
      n224 = Multiply "OFF (Corrected)\nGs to V"(x=w593, y=w547) -> (x*y=w604:dbl)
      n225 = Multiply "OFF (Uncorrected) \nGs to V"(x=w521, y=w547) -> (x*y=w594:dbl)
      n226 = Divide "Jump/Step \nON to Uncorrected \nOFF (Gs)"(x=w579, y=w545) -> (x/y=w581:dbl)
      n227 = Multiply "ON\nGs to V"(x=w608, y=w547) -> (x*y=w671:dbl)
      n228 = Quotient & Remainder "Samples # \nper step"(x=w582, y=w545) -> (floor(x/y)=w576:u32)  [unwired: 1 out]
      n229 = Add "ON + Offset from \nObserved Zero (V)"(x=w594, y=w671) -> (x+y=w691:dbl)
      n230 = case "Correct Null \nFlux?" shown="False" TRUE ("7. Correct Null Flux after Cycle #1?") {
        tunnel: [w735 w737] -> w538
        tunnel: w604 -> [_ w737]
        tunnel: w594 -> [w735 _]
        tunnel: [w734 w736] -> w596
        tunnel: w521 -> [w734 _]
        tunnel: w593 -> [_ w736]
        frame False {
          # "ON"
          # "OFF"
          # "Uncorrected"
        }
        frame True {
          # "Corrected"
        }
      }
      "Corrective \nNull Flux (Gs)" <- w596
      n231 = Subtract "Jump ON to \nCorrected OFF (Gs)"(x=w579, y=w580) -> (x-y=w577:dbl)
      n232 = Divide "Jump/Step\nON to Corrected\nOFF (Gs)"(x=w577, y=w545) -> (x/y=w578:dbl)
      n233 = for "Create Ramp Steps" {
        N: w591 -> [_]
        shift-right: [w731] -> w570
        shift-left: dbl[] [] -> [w733]
        tunnel: w593 -> [w717]
        tunnel: w592 -> [w716]
        tunnel: w548 -> [w723]
        shift-right: [w728] -> w575
        shift-left: dbl[] [] -> [w727]
        tunnel: [w722] -> w568
        tunnel: w576 -> [w722]
        tunnel: w581 -> [w721]
        tunnel: w578 -> [w720]
        i -> [w724]
        n234 = To Double Precision Float(number=w724) -> (double precision float=w726:dbl)
        n235 = Multiply "Going thru\nSteps"(x=w726, y=w720) -> (x*y=w725:dbl)
        n236 = Multiply "Going thru\nSteps"(x=w726, y=w721) -> (x*y=w730:dbl)
        n237 = Add "UnCorrected Null flux Offset"(x=w730, y=w716) -> (x+y=w719:dbl)
        n238 = Add "Corrected Null Flux\nOffset"(x=w725, y=w717) -> (x+y=w718:dbl)
        n239 = Multiply "V to Gs"(x=w719, y=w723) -> (x*y=w715:dbl)
        n240 = Multiply "V to Gs"(x=w723, y=w718) -> (x*y=w714:dbl)
        n241 = Initialize Array "Current \nStep"(w715, w722) -> (w732:dbl[])
        n242 = Initialize Array "Current \nStep"(w714, w722) -> (w729:dbl[])
        n243 = Build Array (concatenate) "Uncorrected OFF\n to ON Ramp (V)"(w733, w732) -> (w731:dbl[])
        n244 = Build Array (concatenate) "Corrected OFF \nto ON Ramp (V)"(w727, w729) -> (w728:dbl[])
      }
      n245 = Multiply "# samples: OFF"(x=w529, y=w531) -> (x*y=w586:dbl)
      n246 = Multiply "# samples ON"(x=w529, y=w603) -> (x*y=w590:dbl)
      n247 = Multiply "Pre-wave Zero Inteval Samples"(x=w676, y=w529) -> (x*y=w689:dbl)
      n248 = Multiply "Post-wave Zero Interval Samples"(x=w675, y=w529) -> (x*y=w537:dbl)
      n249 = Reciprocal "period (s)"(x=w630) -> (1/x=w627:dbl)
      n250 = To Quad Integer(1:w537) -> (0:w535:i64)
      n251 = To Quad Integer(1:w689) -> (0:w536:i64)
      n252 = Multiply "Samples/wave"(x=w631, y=w627) -> (x*y=w628:dbl)
      n253 = Quotient & Remainder "1/4 wave"(x=w628, y=u8 4) -> (floor(x/y)=w624:dbl)  [unwired: 1 out]
      n254 = To Unsigned Long Integer(number=w624) -> (unsigned 32bit integer=w623:u32)
      n255 = Reverse 1D Array "ON to Uncorrected OFF"(array=w570) -> (reversed array=w574:dbl[])
      n256 = Reverse 1D Array "ON to corrected OFF"(array=w575) -> (reversed array=w573:dbl[])
      n257 = Delete From Array "Remove ON"(array=w574, length=w568, index=w569) -> (array with subset deleted=w559:dbl[])  [unwired: 1 out]
      n258 = Delete From Array "Remove ON"(array=w573, length=w568, index=w569) -> (array with subset deleted=w541:dbl[])  [unwired: 1 out]
      n259 = Delete From Array "Remove First \ncorrected OFF step\nto ON"(array=w575, length=w568, index=w569) -> (array with subset deleted=w560:dbl[])  [unwired: 1 out]
      n260 = Delete From Array "Remove First \nUncorrected OFF step\nto ON"(array=w570, length=w568, index=w569) -> (array with subset deleted=w567:dbl[])  [unwired: 1 out]
      n261 = Array Size(array=w567) -> (size(s)=w584:i32)
      n262 = Array Size(array=w541) -> (size(s)=w563:i32)
      n263 = Array Size(array=w560) -> (size(s)=w566:i32)
      n264 = Array Size(array=w559) -> (size(s)=w561:i32)
      n265 = Decrement "last item"(x=w584) -> (x-1=w583:i32)
      n266 = Array Size "Size ON Ramp"(array=w541) -> (size(s)=w562:i32)
      n267 = Array Size "Size OFF Ramp"(array=w560) -> (size(s)=w543:i32)
      n268 = Decrement "last item"(x=w566) -> (x-1=w565:i32)
      n269 = Decrement "last item"(x=w563) -> (x-1=w555:i32)
      n270 = Decrement "last item"(x=w561) -> (x-1=w556:i32)
      n271 = Index Array "ON"(array=w567, index=w583) -> (element=w589:dbl)
      n272 = Index Array "ON"(array=w560, index=w565) -> (element=w588:dbl)
      n273 = Index Array "Corrected OFF"(array=w541, index=w555) -> (element=w539:dbl)
      n274 = Index Array "Uncorrected OFF"(array=w559, index=w556) -> (element=w587:dbl)
      n275 = Subtract "OFF Ramp Samples #"(x=w586, y=w543) -> (x-y=w572:dbl)
      n276 = Subtract "ON Ramp Samples #"(x=w590, y=w562) -> (x-y=w571:dbl)
      n277 = Subtract "Post-Wave OFF Sample #"(x=w535, y=w543) -> (x-y=w540:i64)
      n278 = Initialize Array "Extend PostOFF"(w539, w540) -> (w542:dbl[])
      n279 = Initialize Array "Extend OFF"(w539, w572) -> (w557:dbl[])
      n280 = Initialize Array "Extend ON"(w589, w571) -> (w585:dbl[])
      n281 = Initialize Array "Extend OFF"(w587, w572) -> (w558:dbl[])
      n282 = Initialize Array "Extend ON"(w588, w571) -> (w564:dbl[])
      n283 = Build Array (concatenate) "ON to Corrected OFF (V) First Step Removed\nPost-Wave"(w541, w542) -> (w532:dbl[])
      n284 = Build Array (concatenate) "UnCorrected OFF\n to ON (V)\nFirst Step Removed"(w567, w585) -> (w551:dbl[])
      n285 = Build Array (concatenate) "ON to UnCorrected OFF (V)\nFirst Step Removed"(w559, w558) -> ()  [unwired: 1 out]
      n286 = Build Array (concatenate) "Corrected OFF\n to ON (V)\nFirst Step Removed"(w560, w564) -> (w550:dbl[])
      n287 = Build Array (concatenate) "ON to Corrected OFF (V)\nFirst Step Removed"(w541, w557) -> (w533:dbl[])
      n288 = case "Force Step Ramps" shown="True" TRUE ("9.            Step(s) Force Ramp in              (ms)?") {
        tunnel: [w700 w710] -> w554
        tunnel: w691 -> [w703 _]
        tunnel: [w701 w709] -> w552
        tunnel: [w699 w713] -> w553
        tunnel: w594 -> [w705 w708]
        tunnel: w538 -> [w706 _]
        tunnel: w590 -> [w702 _]
        tunnel: w586 -> [w704 w712]
        tunnel: w550 -> [_ w709]
        tunnel: w551 -> [_ w711]
        tunnel: w533 -> [_ w710]
        tunnel: [w701 w711] -> w549
        tunnel: w532 -> [_ w707]
        tunnel: w538 -> [w698 _]
        tunnel: w535 -> [w697 _]
        tunnel: [w696 w707] -> w534
        frame False {
          # "OFF: 1st cycle"
          # "ON: all cycles"
          # "OFF: 2nd cycle\n& Later"
          # "NO RAMP"
          # "OFF (corrected) to ON (V)"
          # "OFF (Uncorrected) to ON (V)"
          # "ON + Offset from \nObserved Zero (V)"
          n289 = Initialize Array "Post Wave"(w698, w697) -> (w696:dbl[])
          n290 = Initialize Array "1. corrected OFF"(w706, w704) -> (w700:dbl[])
          n291 = Initialize Array "1.  Uncorrected OFF"(w705, w704) -> (w699:dbl[])
          n292 = Initialize Array "2. ON"(w703, w702) -> (w701:dbl[])
        }
        frame True {
          # "OFF: Post-wave Zero"
          # "OFF: 1st cycle"
          # "OFF: 2nd Cycle & Later"
          # "ON: 2nd Cycle & Later"
          # "ON: 1st cycle"
          # "2. On to corrected OFF (V)"
          # "1. uncorrected OFF to ON (V)"
          # "WITH Steps RAMP"
          # "1. corrected OFF to ON (V)"
          n293 = Initialize Array "1. Uncorrected OFF"(w708, w712) -> (w713:dbl[])
        }
      }
      n294 = Subtract(x=w586, y=w616) -> (x-y=w651:dbl)
      n295 = Initialize Array "1. Off"(FALSE, w586) -> (w686:bool[])
      n296 = Initialize Array "2. On"(TRUE, w590) -> (w685:bool[])
      n297 = Initialize Array "2. Off"(0.0 ("dimension size"), w651) -> (w653:dbl[])
      n298 = Initialize Array "2. Off"(FALSE, w651) -> (w669:bool[])
      n299 = Initialize Array "2. Off"(FALSE, w586) -> (w639:bool[])
      n300 = Initialize Array "1. On"(TRUE, w590) -> (w670:bool[])
      n301 = Initialize Array "2. Off"(0.0 ("dimension size"), w586) -> (w637:dbl[])
      n302 = Build Array (concatenate) "1st Cycle\nOne cycle: OFF/ON"(w553, w549) -> (w528:dbl[])
      n303 = Build Array (concatenate) "2nd Cycle & later\nOne Cycle: OFF/ON"(w554, w552) -> (w527:dbl[])
      n304 = Build Array (concatenate) "Magnetic Flux Control\nWaveform OFF/ON? Array"(w686, w685) -> (w682:bool[])
      n305 = Build Array (concatenate) "Mini DeGauss\nAO Waveform Array"(w642, w653) -> (w641:dbl[])
      n306 = To Quad Integer(1:w536) -> (0:w636:i64)
      n307 = Build Array (concatenate) "Mini DeGauss\nWaveform OFF/ON? Array"(w670, w669) -> (w666:bool[])
      n308 = Less?(x=w535, y=w616) -> (x < y?=w654:bool)
      n309 = Less?(x=w636, y=w616) -> (x < y?=w635:bool)
      n310 = case "Pre-Mini DeGauss?" shown="True" w635 {
        tunnel: [w738 w744] -> w634
        tunnel: w636 -> [w739 _]
        tunnel: [w740 w743] -> w633
        frame False {
          # "Modified mini DeGauss to not include it in the \npre-wave on 3/9/2018"
          n311 = Initialize Array "Off"(0.0 ("dimension size"), w739) -> (w740:dbl[])
          n312 = Initialize Array "Off"(FALSE, w739) -> (w738:bool[])
        }
        frame True {
          w743 = dbl[] []  # Initial Zero Array
          w744 = bool[] []  # Initial Empty Array
          # "Pre-wave is smaller than the \nmini-DeGauss cycle"
        }
      }
      n313 = case "Post-Mini DeGauss" shown="False" w654 {
        tunnel: [w774 w780] -> w662
        tunnel: w535 -> [w773 _]
        tunnel: w616 -> [w772 _]
        tunnel: w642 -> [w769 _]
        tunnel: [w767 w779] -> w643
        frame False {
          n314 = Subtract(x=w773, y=w772) -> (x-y=w768:i64)
          n315 = Initialize Array "2. Off"(0.0 ("dimension size"), w768) -> (w771:dbl[])
          n316 = Initialize Array "1. On"(TRUE, w772) -> (w778:bool[])
          n317 = Initialize Array "2. Off"(FALSE, w768) -> (w777:bool[])
          n318 = Build Array (concatenate) "Mini DeGauss\nWaveform OFF/ON? Array"(w769, w771) -> (w767:dbl[])
          n319 = Build Array (concatenate) "Post-Mini DeGauss\nWave"(w778, w777) -> (w774:bool[])
        }
        frame True {
          w779 = dbl[] []  # Initial Zero Array
          w780 = bool[] []  # Initial Empty Array
          # "Post-wave is smaller than the \nmini-DeGauss cycle"
        }
      }
      n320 = for "Building N Cycles of OFF/ON Wavefform" {
        N: w677 -> [_]
        tunnel: w527 -> [w787]
        shift-right: [w785] -> w546
        shift-left: w692 -> [w788]
        shift-right: [w800] -> w680
        shift-left: w663 -> [w802]
        tunnel: w682 -> [w801]
        shift-right: [w799] -> w655
        shift-left: w607 -> [w798]
        tunnel: w666 -> [w797]
        shift-right: [w796] -> w649
        shift-left: w650 -> [w794]
        tunnel: w641 -> [w795]
        tunnel: w639 -> [w790]
        tunnel: w637 -> [w789]
        tunnel: w528 -> [w786]
        i -> [w793]
        n321 = Equal? "First Cycle?"(x=0, y=w793) -> (x = y?=w791:bool)
        n322 = case "First Cycle?" shown="False" w791 {
          tunnel: [w811 w816] -> w799
          tunnel: w798 -> [w810 _]
          tunnel: w797 -> [w809 _]
          tunnel: [w808 w815] -> w796
          tunnel: w795 -> [w807 _]
          tunnel: w794 -> [w806 _]
          tunnel: w790 -> [_ w816]
          tunnel: w789 -> [_ w815]
          tunnel: w788 -> [w805 w814]
          tunnel: [w804 w812] -> w785
          tunnel: w787 -> [w803 _]
          tunnel: w786 -> [_ w813]
          frame False {
            n323 = Build Array (concatenate) "Build Array"(w810, w809) -> (w811:bool[])
            n324 = Build Array (concatenate) "Corrected"(w805, w803) -> (w804:dbl[])
            n325 = Build Array (concatenate) "Build Array"(w806, w807) -> (w808:dbl[])
          }
          frame True {
            n326 = Build Array (concatenate) "Uncorrected"(w814, w813) -> (w812:dbl[])
          }
        }
        n327 = Build Array (concatenate) "Build Array"(w802, w801) -> (w800:bool[])
      }
      n328 = Initialize Array "Pre-Wave"(w594, w636) -> (w602:dbl[])
      n329 = Initialize Array "Pre-Wave Zero"(w681, w636) -> (w665:bool[])
      n330 = Initialize Array "Post Wave Zero"(w681, w535) -> (w664:bool[])
      n331 = Build Array (concatenate) "Mini-DeGauss  \n Waveform OFF/ON? Array"(w634, w655, w662) -> (w659:bool[])
      n332 = Build Array (concatenate) "Mini-DeGauss  \n Waveform AO Sequence"(w633, w649, w643) -> (w647:dbl[])
      n333 = Build Array (concatenate) "Magnetic Flux \nControl Waveform OFF/ON? Array"(w665, w680, w664) -> (w679:bool[])
      n334 = Array Size(array=w647) -> (size(s)=w648:i32)
      n335 = Multiply "Samples/cycle"(x=w529, y=w678) -> (x*y=w690:dbl)
      n336 = Array Size(array=w659) -> (size(s)=w660:i32)
      n337 = Add "Pre & Post Samples"(x=w636, y=w535) -> (x+y=w688:i64)
      n338 = Build Array (concatenate) "Magnetic Flux \nControl Array"(w602, w546, w534) -> (w522:dbl[])
      n339 = Array Size(array=w522) -> (size(s)=w524:i32)
      n340 = for {
        N: w524 -> [_]
        shift-right: [w693] -> w525
        shift-left: i32[] [] -> [w695]
        i -> [w694]
        n341 = Build Array (concatenate)(w695, w694) -> (w693:i32[])
      }
      n342 = Initialize Array "1. Off"(0.0, w648) -> (w645:dbl[])
      n343 = Initialize Array "1. Off"(FALSE, w660) -> (w657:bool[])
      n344 = Multiply "Total Number of OFF/ON Samples"(x=w690, y=w677) -> (x*y=w626:dbl)
      n345 = To Unsigned Long Integer(number=w626) -> (unsigned 32bit integer=w625:u32)
      n346 = case "Mini DeGauss? YES/NO?" shown="False" FALSE ("6. Mini DeGauss cycles in OFF segments?") {
        tunnel: w659 -> [_ w784]
        tunnel: [w782 w784] -> w658
        tunnel: w657 -> [w782 _]
        tunnel: w647 -> [_ w783]
        tunnel: w645 -> [w781 _]
        tunnel: [w781 w783] -> w644
        frame False {
          # "NO mini\nDeGauss \ncycles"
        }
        frame True {
          # "Mini DeGauss\ncycles"
        }
      }
      n347 = Divide(x=w525, y=w524) -> (x/y=w523:dbl[])
      n348 = Bundle(w523, w522) -> ()  [unwired: 1 in, 1 out]
      n349 = Add "Total # of Samples"(x=w625, y=w688) -> (x+y=w687:i64)
      "Zero Flux Observed GS" <- w521
    }
    frame #16 {
      # "1/4 wave to get the main points of the\n mini DeGauss waveform 3/12/2018"
      # "# of samples of Mini DeGauss"
      # "Flux ON/OFF Logical"
      # "Sampling Rate"
      # "Flux Control Sequence"
      # "Mini DeGauss AO Sequence, Normalized"
      # "Mini DeGauss Logical"
      # "AO values of current"
      # "1 for #1\n2 for #2"
      # "#WIM 1/16/2018\nPID Aggressiveness\n0 = Optimized\n1 = Minimum\n2 = Average\n3 = Maximum"
      # "Step 4 Specifying PID Parameters"
      # "Total Number of Samples"
      # "#WIM 1/10/2018\nPID Parameters List Selection:\n0 = Fixed Schedule\n1 = Interpolated Schedule"
      n350 = shared-variable "NI-GenericDesktopPC-3A84958E\\Kopco PS Project Target Variables Library.lvlib\\Needle Used"() -> (w847:i8)  [unwired: 1 in, 1 out]
      n351 = shared-variable "NI-GenericDesktopPC-3A84958E\\Kopco PS Project Target Variables Library.lvlib\\Period OFF 1st Per Cycle"("1st OFF Length (s)") -> ()  [unwired: 1 in, 1 out]
      n352 = shared-variable "NI-GenericDesktopPC-3A84958E\\Kopco PS Project Target Variables Library.lvlib\\Sampling Rate"() -> (w839:dbl)  [unwired: 1 in, 1 out]
      n353 = case "Needle Chosen: #1 or #2" shown="1, Default" w847 {
        tunnel: [w885 w891] -> w853
        tunnel: [w884 w890] -> w852
        tunnel: [w883 w886] -> w851
        tunnel: [w882 w889] -> w850
        tunnel: [w881 w887] -> w842
        tunnel: [w880 w888] -> w841
        frame 1, Default {
          w880 = T2 [{"PID gains"={"proportional gain (Kc)"=0.053, "integral time (Ti, min)"=3.5e-06, "derivative time (Td, min)"=0.0}, "max value"=0.0}, {"PID gains"={"proportional gain (Kc)"=0.053, "integral time (Ti, min)"=3.5e-06, "derivative time (Td, min)"=0.0}, "max value"=75.0}, {"PID gains"={"proportional gain (Kc)"=0.053, "integral time (Ti, min)"=3.5e-06, "derivative time (Td, min)"=0.0}, "max value"=100.0}, {"PID gains"={"proportional gain (Kc)"=0.055, "integral time (Ti, min)"=3.5e-06, "derivative time (Td, min)"=0.0}, "max value"=125.0}, {"PID gains"={"proportional gain (Kc)"=0.055, "integral time (Ti, min)"=3.5e-06, "derivative time (Td, min)"=0.0}, "max value"=150.0}, {"PID gains"={"proportional gain (Kc)"=0.055, "integral time (Ti, min)"=3.5e-06, "derivative time (Td, min)"=0.0}, "max value"=160.0}, {"PID gains"={"proportional gain (Kc)"=0.056, "integral time (Ti, min)"=3.5e-06, "derivative time (Td, min)"=0.0}, "max value"=165.0}, {"PID gains"={"proportional gain (Kc)"=0.056, "integral time (Ti, min)"=3.5e-06, "derivative time (Td, min)"=0.0}, "max value"=170.0}, {"PID gains"={"proportional gain (Kc)"=0.058, "integral time (Ti, min)"=3.5e-06, "derivative time (Td, min)"=0.0}, "max value"=175.0}, {"PID gains"={"proportional gain (Kc)"=0.058, "integral time (Ti, min)"=3.5e-06, "derivative time (Td, min)"=0.0}, "max value"=180.0}, {"PID gains"={"proportional gain (Kc)"=0.058, "integral time (Ti, min)"=3.5e-06, "derivative time (Td, min)"=0.0}, "max value"=185.0}, {"PID gains"={"proportional gain (Kc)"=0.058, "integral time (Ti, min)"=3.5e-06, "derivative time (Td, min)"=0.0}, "max value"=190.0}, {"PID gains"={"proportional gain (Kc)"=0.058, "integral time (Ti, min)"=3.5e-06, "derivative time (Td, min)"=0.0}, "max value"=210.0}]  # OFF PID gain schedule HyMu80#1 Needle OPTIMIZED
          w881 = T2 [{"PID gains"={"proportional gain (Kc)"=0.053, "integral time (Ti, min)"=3.5e-06, "derivative time (Td, min)"=0.0}, "max value"=0.0}, {"PID gains"={"proportional gain (Kc)"=0.053, "integral time (Ti, min)"=3.5e-06, "derivative time (Td, min)"=0.0}, "max value"=75.0}, {"PID gains"={"proportional gain (Kc)"=0.053, "integral time (Ti, min)"=3.5e-06, "derivative time (Td, min)"=0.0}, "max value"=100.0}, {"PID gains"={"proportional gain (Kc)"=0.055, "integral time (Ti, min)"=3.5e-06, "derivative time (Td, min)"=0.0}, "max value"=125.0}, {"PID gains"={"proportional gain (Kc)"=0.057, "integral time (Ti, min)"=3.5e-06, "derivative time (Td, min)"=0.0}, "max value"=150.0}, {"PID gains"={"proportional gain (Kc)"=0.058, "integral time (Ti, min)"=3.5e-06, "derivative time (Td, min)"=0.0}, "max value"=160.0}, {"PID gains"={"proportional gain (Kc)"=0.065, "integral time (Ti, min)"=3.5e-06, "derivative time (Td, min)"=0.0}, "max value"=165.0}, {"PID gains"={"proportional gain (Kc)"=0.111, "integral time (Ti, min)"=3.5e-06, "derivative time (Td, min)"=0.0}, "max value"=170.0}, {"PID gains"={"proportional gain (Kc)"=0.27, "integral time (Ti, min)"=3.5e-06, "derivative time (Td, min)"=0.0}, "max value"=175.0}, {"PID gains"={"proportional gain (Kc)"=0.32, "integral time (Ti, min)"=3.5e-06, "derivative time (Td, min)"=0.0}, "max value"=180.0}, {"PID gains"={"proportional gain (Kc)"=0.72, "integral time (Ti, min)"=3.5e-06, "derivative time (Td, min)"=0.0}, "max value"=185.0}, {"PID gains"={"proportional gain (Kc)"=0.8, "integral time (Ti, min)"=3.5e-06, "derivative time (Td, min)"=0.0}, "max value"=190.0}, {"PID gains"={"proportional gain (Kc)"=0.8, "integral time (Ti, min)"=3.5e-06, "derivative time (Td, min)"=0.0}, "max value"=210.0}]  # ON PID gain schedule HyMu80#1 Needle OPTIMIZED
          w882 = T2 [{"PID gains"={"proportional gain (Kc)"=0.08, "integral time (Ti, min)"=3.5e-06, "derivative time (Td, min)"=0.0}, "max value"=0.0}, {"PID gains"={"proportional gain (Kc)"=0.08, "integral time (Ti, min)"=3.5e-06, "derivative time (Td, min)"=0.0}, "max value"=145.0}, {"PID gains"={"proportional gain (Kc)"=0.075, "integral time (Ti, min)"=3.5e-06, "derivative time (Td, min)"=0.0}, "max value"=148.0}, {"PID gains"={"proportional gain (Kc)"=0.075, "integral time (Ti, min)"=3.5e-06, "derivative time (Td, min)"=0.0}, "max value"=150.0}, {"PID gains"={"proportional gain (Kc)"=0.075, "integral time (Ti, min)"=3.5e-06, "derivative time (Td, min)"=0.0}, "max value"=155.0}, {"PID gains"={"proportional gain (Kc)"=0.075, "integral time (Ti, min)"=3.5e-06, "derivative time (Td, min)"=0.0}, "max value"=160.0}, {"PID gains"={"proportional gain (Kc)"=0.078, "integral time (Ti, min)"=3.5e-06, "derivative time (Td, min)"=0.0}, "max value"=165.0}, {"PID gains"={"proportional gain (Kc)"=0.078, "integral time (Ti, min)"=3.5e-06, "derivative time (Td, min)"=0.0}, "max value"=170.0}, {"PID gains"={"proportional gain (Kc)"=0.081, "integral time (Ti, min)"=3.5e-06, "derivative time (Td, min)"=0.0}, "max value"=175.0}, {"PID gains"={"proportional gain (Kc)"=0.08, "integral time (Ti, min)"=3.5e-06, "derivative time (Td, min)"=0.0}, "max value"=180.0}, {"PID gains"={"proportional gain (Kc)"=0.085, "integral time (Ti, min)"=3.5e-06, "derivative time (Td, min)"=0.0}, "max value"=185.0}, {"PID gains"={"proportional gain (Kc)"=0.086, "integral time (Ti, min)"=3.5e-06, "derivative time (Td, min)"=0.0}, "max value"=190.0}, {"PID gains"={"proportional gain (Kc)"=0.086, "integral time (Ti, min)"=3.5e-06, "derivative time (Td, min)"=0.0}, "max value"=195.0}, {"PID gains"={"proportional gain (Kc)"=0.086, "integral time (Ti, min)"=3.5e-06, "derivative time (Td, min)"=0.0}, "max value"=220.0}]  # OFF PID gain schedule HyMu80#1 Needle MAX
          w883 = T2 [{"PID gains"={"proportional gain (Kc)"=0.08, "integral time (Ti, min)"=3.5e-06, "derivative time (Td, min)"=0.0}, "max value"=0.0}, {"PID gains"={"proportional gain (Kc)"=0.08, "integral time (Ti, min)"=3.5e-06, "derivative time (Td, min)"=0.0}, "max value"=145.0}, {"PID gains"={"proportional gain (Kc)"=0.075, "integral time (Ti, min)"=3.5e-06, "derivative time (Td, min)"=0.0}, "max value"=148.0}, {"PID gains"={"proportional gain (Kc)"=0.075, "integral time (Ti, min)"=3.5e-06, "derivative time (Td, min)"=0.0}, "max value"=150.0}, {"PID gains"={"proportional gain (Kc)"=0.075, "integral time (Ti, min)"=3.5e-06, "derivative time (Td, min)"=0.0}, "max value"=155.0}, {"PID gains"={"proportional gain (Kc)"=0.075, "integral time (Ti, min)"=3.5e-06, "derivative time (Td, min)"=0.0}, "max value"=160.0}, {"PID gains"={"proportional gain (Kc)"=0.078, "integral time (Ti, min)"=3.5e-06, "derivative time (Td, min)"=0.0}, "max value"=165.0}, {"PID gains"={"proportional gain (Kc)"=0.078, "integral time (Ti, min)"=3.5e-06, "derivative time (Td, min)"=0.0}, "max value"=170.0}, {"PID gains"={"proportional gain (Kc)"=0.081, "integral time (Ti, min)"=3.5e-06, "derivative time (Td, min)"=0.0}, "max value"=175.0}, {"PID gains"={"proportional gain (Kc)"=0.08, "integral time (Ti, min)"=3.5e-06, "derivative time (Td, min)"=0.0}, "max value"=180.0}, {"PID gains"={"proportional gain (Kc)"=0.085, "integral time (Ti, min)"=3.5e-06, "derivative time (Td, min)"=0.0}, "max value"=185.0}, {"PID gains"={"proportional gain (Kc)"=0.086, "integral time (Ti, min)"=3.5e-06, "derivative time (Td, min)"=0.0}, "max value"=190.0}, {"PID gains"={"proportional gain (Kc)"=0.086, "integral time (Ti, min)"=3.5e-06, "derivative time (Td, min)"=0.0}, "max value"=195.0}, {"PID gains"={"proportional gain (Kc)"=0.086, "integral time (Ti, min)"=3.5e-06, "derivative time (Td, min)"=0.0}, "max value"=220.0}]  # OFF PID gain schedule HyMu80#1 Needle MIN
          w884 = T2 [{"PID gains"={"proportional gain (Kc)"=0.08, "integral time (Ti, min)"=3.5e-06, "derivative time (Td, min)"=0.0}, "max value"=0.0}, {"PID gains"={"proportional gain (Kc)"=0.08, "integral time (Ti, min)"=3.5e-06, "derivative time (Td, min)"=0.0}, "max value"=145.0}, {"PID gains"={"proportional gain (Kc)"=0.083, "integral time (Ti, min)"=3.5e-06, "derivative time (Td, min)"=0.0}, "max value"=148.0}, {"PID gains"={"proportional gain (Kc)"=0.085, "integral time (Ti, min)"=3.5e-06, "derivative time (Td, min)"=0.0}, "max value"=150.0}, {"PID gains"={"proportional gain (Kc)"=0.0875, "integral time (Ti, min)"=3.5e-06, "derivative time (Td, min)"=0.0}, "max value"=155.0}, {"PID gains"={"proportional gain (Kc)"=0.123, "integral time (Ti, min)"=3.5e-06, "derivative time (Td, min)"=0.0}, "max value"=160.0}, {"PID gains"={"proportional gain (Kc)"=0.207, "integral time (Ti, min)"=3.5e-06, "derivative time (Td, min)"=0.0}, "max value"=165.0}, {"PID gains"={"proportional gain (Kc)"=0.315, "integral time (Ti, min)"=3.5e-06, "derivative time (Td, min)"=0.0}, "max value"=170.0}, {"PID gains"={"proportional gain (Kc)"=0.46, "integral time (Ti, min)"=3.5e-06, "derivative time (Td, min)"=0.0}, "max value"=175.0}, {"PID gains"={"proportional gain (Kc)"=0.65, "integral time (Ti, min)"=3.5e-06, "derivative time (Td, min)"=0.0}, "max value"=180.0}, {"PID gains"={"proportional gain (Kc)"=0.925, "integral time (Ti, min)"=3.5e-06, "derivative time (Td, min)"=0.0}, "max value"=185.0}, {"PID gains"={"proportional gain (Kc)"=1.04, "integral time (Ti, min)"=3.5e-06, "derivative time (Td, min)"=0.0}, "max value"=190.0}, {"PID gains"={"proportional gain (Kc)"=1.04, "integral time (Ti, min)"=3.5e-06, "derivative time (Td, min)"=0.0}, "max value"=195.0}, {"PID gains"={"proportional gain (Kc)"=1.04, "integral time (Ti, min)"=3.5e-06, "derivative time (Td, min)"=0.0}, "max value"=220.0}]  # ON PID gain schedule HyMu80#1 Needle MAX
          w885 = T2 [{"PID gains"={"proportional gain (Kc)"=0.075, "integral time (Ti, min)"=3.5e-06, "derivative time (Td, min)"=0.0}, "max value"=0.0}, {"PID gains"={"proportional gain (Kc)"=0.075, "integral time (Ti, min)"=3.5e-06, "derivative time (Td, min)"=0.0}, "max value"=145.0}, {"PID gains"={"proportional gain (Kc)"=0.075, "integral time (Ti, min)"=3.5e-06, "derivative time (Td, min)"=0.0}, "max value"=148.0}, {"PID gains"={"proportional gain (Kc)"=0.075, "integral time (Ti, min)"=3.5e-06, "derivative time (Td, min)"=0.0}, "max value"=150.0}, {"PID gains"={"proportional gain (Kc)"=0.0775, "integral time (Ti, min)"=3.5e-06, "derivative time (Td, min)"=0.0}, "max value"=155.0}, {"PID gains"={"proportional gain (Kc)"=0.117, "integral time (Ti, min)"=3.5e-06, "derivative time (Td, min)"=0.0}, "max value"=160.0}, {"PID gains"={"proportional gain (Kc)"=0.187, "integral time (Ti, min)"=3.5e-06, "derivative time (Td, min)"=0.0}, "max value"=165.0}, {"PID gains"={"proportional gain (Kc)"=0.28, "integral time (Ti, min)"=3.5e-06, "derivative time (Td, min)"=0.0}, "max value"=170.0}, {"PID gains"={"proportional gain (Kc)"=0.425, "integral time (Ti, min)"=3.5e-06, "derivative time (Td, min)"=0.0}, "max value"=175.0}, {"PID gains"={"proportional gain (Kc)"=0.615, "integral time (Ti, min)"=3.5e-06, "derivative time (Td, min)"=0.0}, "max value"=180.0}, {"PID gains"={"proportional gain (Kc)"=0.85, "integral time (Ti, min)"=3.5e-06, "derivative time (Td, min)"=0.0}, "max value"=185.0}, {"PID gains"={"proportional gain (Kc)"=1.0, "integral time (Ti, min)"=3.5e-06, "derivative time (Td, min)"=0.0}, "max value"=190.0}, {"PID gains"={"proportional gain (Kc)"=1.0, "integral time (Ti, min)"=3.5e-06, "derivative time (Td, min)"=0.0}, "max value"=195.0}, {"PID gains"={"proportional gain (Kc)"=1.0, "integral time (Ti, min)"=3.5e-06, "derivative time (Td, min)"=0.0}, "max value"=220.0}]  # ON PID gain schedule HyMu80#1 Needle MIN
          # "Updated on 2019-08-27"
          # "11/5/2018. Modified the PID gains for values 170 Gs and higher to make it more aggressive near the end."
          # "### values ABOVE ARE NOT UPDATED!!!! 3/25/2018"
          # "No discontinuity flux values will be selected\nNote: values that can leakage/ghosting/discontinuity in flux signals are not used.\nThis problem can be minimized by a number of techniques. However, I am not going to invest time \nin this right now. I can still generate fluxes of almost 200 Gs if Null Flux is -25 or -40 Gs. #WIM 1/16/2018"
          # "HyMu80#1 Needle Schedules Tuned on  1/11 & 12/2018 by #WIM\nfor fluxes:  ON/OFF\n145, 148, 150, 155, 160, 165, 170, 175, 180, 185, 190, 195 Gs\n220 Gs is for anything extra"
          # "HyMu80#1 Needle PID Parameters"
        }
        frame 2 {
          w888 = T2 [{"PID gains"={"proportional gain (Kc)"=0.053, "integral time (Ti, min)"=3.5e-06, "derivative time (Td, min)"=0.0}, "max value"=0.0}, {"PID gains"={"proportional gain (Kc)"=0.053, "integral time (Ti, min)"=3.5e-06, "derivative time (Td, min)"=0.0}, "max value"=75.0}, {"PID gains"={"proportional gain (Kc)"=0.053, "integral time (Ti, min)"=3.5e-06, "derivative time (Td, min)"=0.0}, "max value"=100.0}, {"PID gains"={"proportional gain (Kc)"=0.055, "integral time (Ti, min)"=3.5e-06, "derivative time (Td, min)"=0.0}, "max value"=125.0}, {"PID gains"={"proportional gain (Kc)"=0.055, "integral time (Ti, min)"=3.5e-06, "derivative time (Td, min)"=0.0}, "max value"=150.0}, {"PID gains"={"proportional gain (Kc)"=0.055, "integral time (Ti, min)"=3.5e-06, "derivative time (Td, min)"=0.0}, "max value"=160.0}, {"PID gains"={"proportional gain (Kc)"=0.055, "integral time (Ti, min)"=3.5e-06, "derivative time (Td, min)"=0.0}, "max value"=165.0}, {"PID gains"={"proportional gain (Kc)"=0.056, "integral time (Ti, min)"=3.5e-06, "derivative time (Td, min)"=0.0}, "max value"=170.0}, {"PID gains"={"proportional gain (Kc)"=0.057, "integral time (Ti, min)"=3.5e-06, "derivative time (Td, min)"=0.0}, "max value"=175.0}, {"PID gains"={"proportional gain (Kc)"=0.057, "integral time (Ti, min)"=3.5e-06, "derivative time (Td, min)"=0.0}, "max value"=180.0}, {"PID gains"={"proportional gain (Kc)"=0.057, "integral time (Ti, min)"=3.5e-06, "derivative time (Td, min)"=0.0}, "max value"=185.0}, {"PID gains"={"proportional gain (Kc)"=0.057, "integral time (Ti, min)"=3.5e-06, "derivative time (Td, min)"=0.0}, "max value"=190.0}, {"PID gains"={"proportional gain (Kc)"=0.057, "integral time (Ti, min)"=3.5e-06, "derivative time (Td, min)"=0.0}, "max value"=210.0}]  # OFF PID gain schedule HyMu80#1 Needle OPTIMIZED
          w887 = T2 [{"PID gains"={"proportional gain (Kc)"=0.053, "integral time (Ti, min)"=3.5e-06, "derivative time (Td, min)"=0.0}, "max value"=0.0}, {"PID gains"={"proportional gain (Kc)"=0.053, "integral time (Ti, min)"=3.5e-06, "derivative time (Td, min)"=0.0}, "max value"=75.0}, {"PID gains"={"proportional gain (Kc)"=0.053, "integral time (Ti, min)"=3.5e-06, "derivative time (Td, min)"=0.0}, "max value"=100.0}, {"PID gains"={"proportional gain (Kc)"=0.055, "integral time (Ti, min)"=3.5e-06, "derivative time (Td, min)"=0.0}, "max value"=125.0}, {"PID gains"={"proportional gain (Kc)"=0.057, "integral time (Ti, min)"=3.5e-06, "derivative time (Td, min)"=0.0}, "max value"=150.0}, {"PID gains"={"proportional gain (Kc)"=0.058, "integral time (Ti, min)"=3.5e-06, "derivative time (Td, min)"=0.0}, "max value"=160.0}, {"PID gains"={"proportional gain (Kc)"=0.065, "integral time (Ti, min)"=3.5e-06, "derivative time (Td, min)"=0.0}, "max value"=165.0}, {"PID gains"={"proportional gain (Kc)"=0.111, "integral time (Ti, min)"=3.5e-06, "derivative time (Td, min)"=0.0}, "max value"=170.0}, {"PID gains"={"proportional gain (Kc)"=0.185, "integral time (Ti, min)"=3.5e-06, "derivative time (Td, min)"=0.0}, "max value"=175.0}, {"PID gains"={"proportional gain (Kc)"=0.31, "integral time (Ti, min)"=3.5e-06, "derivative time (Td, min)"=0.0}, "max value"=180.0}, {"PID gains"={"proportional gain (Kc)"=0.55, "integral time (Ti, min)"=3.5e-06, "derivative time (Td, min)"=0.0}, "max value"=185.0}, {"PID gains"={"proportional gain (Kc)"=0.8, "integral time (Ti, min)"=3.5e-06, "derivative time (Td, min)"=0.0}, "max value"=190.0}, {"PID gains"={"proportional gain (Kc)"=0.8, "integral time (Ti, min)"=3.5e-06, "derivative time (Td, min)"=0.0}, "max value"=210.0}]  # ON PID gain schedule HyMu80#1 Needle OPTIMIZED
          w889 = T2 [{"PID gains"={"proportional gain (Kc)"=0.085, "integral time (Ti, min)"=3.5e-06, "derivative time (Td, min)"=0.0}, "max value"=0.0}, {"PID gains"={"proportional gain (Kc)"=0.085, "integral time (Ti, min)"=3.5e-06, "derivative time (Td, min)"=0.0}, "max value"=145.0}, {"PID gains"={"proportional gain (Kc)"=0.088, "integral time (Ti, min)"=3.5e-06, "derivative time (Td, min)"=0.0}, "max value"=148.0}, {"PID gains"={"proportional gain (Kc)"=0.091, "integral time (Ti, min)"=3.5e-06, "derivative time (Td, min)"=0.0}, "max value"=150.0}, {"PID gains"={"proportional gain (Kc)"=0.091, "integral time (Ti, min)"=3.5e-06, "derivative time (Td, min)"=0.0}, "max value"=155.0}, {"PID gains"={"proportional gain (Kc)"=0.092, "integral time (Ti, min)"=3.5e-06, "derivative time (Td, min)"=0.0}, "max value"=160.0}, {"PID gains"={"proportional gain (Kc)"=0.0935, "integral time (Ti, min)"=3.5e-06, "derivative time (Td, min)"=0.0}, "max value"=165.0}, {"PID gains"={"proportional gain (Kc)"=0.094, "integral time (Ti, min)"=3.5e-06, "derivative time (Td, min)"=0.0}, "max value"=170.0}, {"PID gains"={"proportional gain (Kc)"=0.0935, "integral time (Ti, min)"=3.5e-06, "derivative time (Td, min)"=0.0}, "max value"=175.0}, {"PID gains"={"proportional gain (Kc)"=0.097, "integral time (Ti, min)"=3.5e-06, "derivative time (Td, min)"=0.0}, "max value"=180.0}, {"PID gains"={"proportional gain (Kc)"=0.0945, "integral time (Ti, min)"=3.5e-06, "derivative time (Td, min)"=0.0}, "max value"=185.0}, {"PID gains"={"proportional gain (Kc)"=0.0945, "integral time (Ti, min)"=3.5e-06, "derivative time (Td, min)"=0.0}, "max value"=210.0}]  # OFF PID gain schedule HyMu80#2 Needle MAX
          w886 = T2 [{"PID gains"={"proportional gain (Kc)"=0.08, "integral time (Ti, min)"=3.5e-06, "derivative time (Td, min)"=0.0}, "max value"=0.0}, {"PID gains"={"proportional gain (Kc)"=0.08, "integral time (Ti, min)"=3.5e-06, "derivative time (Td, min)"=0.0}, "max value"=145.0}, {"PID gains"={"proportional gain (Kc)"=0.08, "integral time (Ti, min)"=3.5e-06, "derivative time (Td, min)"=0.0}, "max value"=148.0}, {"PID gains"={"proportional gain (Kc)"=0.082, "integral time (Ti, min)"=3.5e-06, "derivative time (Td, min)"=0.0}, "max value"=150.0}, {"PID gains"={"proportional gain (Kc)"=0.082, "integral time (Ti, min)"=3.5e-06, "derivative time (Td, min)"=0.0}, "max value"=155.0}, {"PID gains"={"proportional gain (Kc)"=0.082, "integral time (Ti, min)"=3.5e-06, "derivative time (Td, min)"=0.0}, "max value"=160.0}, {"PID gains"={"proportional gain (Kc)"=0.082, "integral time (Ti, min)"=3.5e-06, "derivative time (Td, min)"=0.0}, "max value"=165.0}, {"PID gains"={"proportional gain (Kc)"=0.083, "integral time (Ti, min)"=3.5e-06, "derivative time (Td, min)"=0.0}, "max value"=170.0}, {"PID gains"={"proportional gain (Kc)"=0.087, "integral time (Ti, min)"=3.5e-06, "derivative time (Td, min)"=0.0}, "max value"=175.0}, {"PID gains"={"proportional gain (Kc)"=0.092, "integral time (Ti, min)"=3.5e-06, "derivative time (Td, min)"=0.0}, "max value"=180.0}, {"PID gains"={"proportional gain (Kc)"=0.091, "integral time (Ti, min)"=3.5e-06, "derivative time (Td, min)"=0.0}, "max value"=185.0}, {"PID gains"={"proportional gain (Kc)"=0.091, "integral time (Ti, min)"=3.5e-06, "derivative time (Td, min)"=0.0}, "max value"=210.0}]  # OFF PID gain schedule HyMu80#2 Needle MIN
          w890 = T2 [{"PID gains"={"proportional gain (Kc)"=0.085, "integral time (Ti, min)"=3.5e-06, "derivative time (Td, min)"=0.0}, "max value"=0.0}, {"PID gains"={"proportional gain (Kc)"=0.085, "integral time (Ti, min)"=3.5e-06, "derivative time (Td, min)"=0.0}, "max value"=145.0}, {"PID gains"={"proportional gain (Kc)"=0.088, "integral time (Ti, min)"=3.5e-06, "derivative time (Td, min)"=0.0}, "max value"=148.0}, {"PID gains"={"proportional gain (Kc)"=0.113, "integral time (Ti, min)"=3.5e-06, "derivative time (Td, min)"=0.0}, "max value"=150.0}, {"PID gains"={"proportional gain (Kc)"=0.195, "integral time (Ti, min)"=3.5e-06, "derivative time (Td, min)"=0.0}, "max value"=155.0}, {"PID gains"={"proportional gain (Kc)"=0.31, "integral time (Ti, min)"=3.5e-06, "derivative time (Td, min)"=0.0}, "max value"=160.0}, {"PID gains"={"proportional gain (Kc)"=0.47, "integral time (Ti, min)"=3.5e-06, "derivative time (Td, min)"=0.0}, "max value"=165.0}, {"PID gains"={"proportional gain (Kc)"=0.725, "integral time (Ti, min)"=3.5e-06, "derivative time (Td, min)"=0.0}, "max value"=170.0}, {"PID gains"={"proportional gain (Kc)"=1.06, "integral time (Ti, min)"=3.5e-06, "derivative time (Td, min)"=0.0}, "max value"=175.0}, {"PID gains"={"proportional gain (Kc)"=1.3, "integral time (Ti, min)"=3.5e-06, "derivative time (Td, min)"=0.0}, "max value"=180.0}, {"PID gains"={"proportional gain (Kc)"=1.2, "integral time (Ti, min)"=3.5e-06, "derivative time (Td, min)"=0.0}, "max value"=185.0}, {"PID gains"={"proportional gain (Kc)"=1.2, "integral time (Ti, min)"=3.5e-06, "derivative time (Td, min)"=0.0}, "max value"=210.0}]  # ON PID gain schedule HyMu80#2 Needle MAX
          w891 = T2 [{"PID gains"={"proportional gain (Kc)"=0.08, "integral time (Ti, min)"=3.5e-06, "derivative time (Td, min)"=0.0}, "max value"=0.0}, {"PID gains"={"proportional gain (Kc)"=0.08, "integral time (Ti, min)"=3.5e-06, "derivative time (Td, min)"=0.0}, "max value"=145.0}, {"PID gains"={"proportional gain (Kc)"=0.08, "integral time (Ti, min)"=3.5e-06, "derivative time (Td, min)"=0.0}, "max value"=148.0}, {"PID gains"={"proportional gain (Kc)"=0.107, "integral time (Ti, min)"=3.5e-06, "derivative time (Td, min)"=0.0}, "max value"=150.0}, {"PID gains"={"proportional gain (Kc)"=0.188, "integral time (Ti, min)"=3.5e-06, "derivative time (Td, min)"=0.0}, "max value"=155.0}, {"PID gains"={"proportional gain (Kc)"=0.27, "integral time (Ti, min)"=3.5e-06, "derivative time (Td, min)"=0.0}, "max value"=160.0}, {"PID gains"={"proportional gain (Kc)"=0.435, "integral time (Ti, min)"=3.5e-06, "derivative time (Td, min)"=0.0}, "max value"=165.0}, {"PID gains"={"proportional gain (Kc)"=0.675, "integral time (Ti, min)"=3.5e-06, "derivative time (Td, min)"=0.0}, "max value"=170.0}, {"PID gains"={"proportional gain (Kc)"=0.945, "integral time (Ti, min)"=3.5e-06, "derivative time (Td, min)"=0.0}, "max value"=175.0}, {"PID gains"={"proportional gain (Kc)"=1.1, "integral time (Ti, min)"=3.5e-06, "derivative time (Td, min)"=0.0}, "max value"=180.0}, {"PID gains"={"proportional gain (Kc)"=1.15, "integral time (Ti, min)"=3.5e-06, "derivative time (Td, min)"=0.0}, "max value"=185.0}, {"PID gains"={"proportional gain (Kc)"=1.15, "integral time (Ti, min)"=3.5e-06, "derivative time (Td, min)"=0.0}, "max value"=210.0}]  # ON PID gain schedule HyMu80#2 Needle MIN
          # "Updated on 2019-08-14"
          # "### values HERE ARE NOT UPDATED!!!! 3/25/2018"
          # "No discontinuity flux values will be selected\nNote: values that can leakage/ghosting/discontinuity in flux signals are not used.\nThis problem can be minimized by a number of techniques. However, I am not going to invest time \nin this right now. I can still generate fluxes of almost 200 Gs if Null Flux is -25 or -40 Gs. #WIM 1/16/2018"
          # "HyMu80#2 Needle Schedules Tuned on  1/9 & 10/2018 by #WIM\nfor fluxes:  ON/OFF\n145, 148, 150, 155, 160, 165, 170, 175, 180, 185 Gs. \n220 Gs is for anything extra"
          # "HyMu80#2 Needle PID Parameters"
        }
      }
      n354 = Greater?(x=w840, y="1st OFF Length (s)") -> (0:w831:bool)
      n355 = shared-variable "NI-GenericDesktopPC-3A84958E\\Kopco PS Project Target Variables Library.lvlib\\Flux Setpoint ON Gs Relative"() -> (w854:dbl)  [unwired: 1 in, 1 out]
      n356 = case shown="True" w831 {
        tunnel: "1st OFF Length (s)" -> [_ w879]
        tunnel: w840 -> [_ w878]
        tunnel: w839 -> [_ w876]
        tunnel: w838 -> [w862 w872]
        tunnel: [w862 w873] -> w837
        tunnel: [w861 w874] -> w835
        tunnel: w836 -> [w861 w875]
        tunnel: w834 -> [w860 w870]
        tunnel: [w860 w871] -> w833
        tunnel: w832 -> [w859 w868]
        tunnel: [w859 w869] -> w818
        tunnel: w829 -> [w858 w866]
        tunnel: [w858 w865] -> _
        frame False {
        }
        frame True {
          w867 = 0 ("index")
          n357 = Subtract(x=w878, y=w879) -> (x-y=w877:dbl)
          n358 = Multiply(x=w876, y=w877) -> (x*y=w864:dbl)
          n359 = To Quad Integer(1:w864) -> (0:w863:i64)
          n360 = Subtract(x=w866, y=w863) -> (x-y=w865:i64)
          n361 = Delete From Array(array=w872, length=w863, index=w867) -> (array with subset deleted=w873:bool[])  [unwired: 1 out]
          n362 = Delete From Array(array=w870, length=w863, index=w867) -> (array with subset deleted=w871:dbl[])  [unwired: 1 out]
          n363 = Delete From Array(array=w868, length=w863, index=w867) -> (array with subset deleted=w869:dbl[])  [unwired: 1 out]
          n364 = Delete From Array(array=w875, length=w863, index=w867) -> (array with subset deleted=w874:bool[])  [unwired: 1 out]
        }
      }
      n365 = shared-variable "NI-GenericDesktopPC-3A84958E\\Kopco PS Project Target Variables Library.lvlib\\Zero Flux Observed GS"() -> (w855:dbl)  [unwired: 1 in, 1 out]
      n366 = Add(x=w854, y=w855) -> (x+y=w819:dbl)
      "ON Absolute\nFlux Setpoint (Gs)" <- w819
      n367 = Array Size(array=w818) -> (size(s)=w817:i32)
      n368 = Absolute Value(x=w819) -> (abs(x)=w825:dbl)
      n369 = shared-variable "NI-GenericDesktopPC-3A84958E\\Kopco PS Project Target Variables Library.lvlib\\Samples Total"(w817) -> ()  [unwired: 1 in, 1 out]
      n370 = shared-variable "NI-GenericDesktopPC-3A84958E\\Kopco PS Project Target Variables Library.lvlib\\Flux Setpoint ON Gs Absolute"(w819) -> ()  [unwired: 1 in, 1 out]
      n371 = Array Size(array=w818) -> (size(s)=w823:i32)
      n372 = Decrement(x=w823) -> (x-1=w822:i32)
      n373 = case "OFF Flux PID Gain Parameters: Interpolated vs. Fixed" shown="0, Default" w849 {
        tunnel: w825 -> [w895 w1040]
        tunnel: [w897 w1042] -> w843
        tunnel: w851 -> [w896 w1039]
        tunnel: w850 -> [w894 w1041]
        tunnel: w848 -> [w893 w1038]
        tunnel: w841 -> [w892 w1037]
        frame 0, Default {
          # "Interpolated Schedule"
          n374 = case "PID Paramter Aggressiveness" shown="1" w893 {
            tunnel: [w900 w932 w966 w1007] -> w897
            tunnel: w896 -> [_ w930 w963 _]
            tunnel: w895 -> [w899 w931 w962 w1006]
            tunnel: w894 -> [_ _ w964 w1005]
            tunnel: w892 -> [w898 _ _ _]
            frame 0, Default {
              w910 = dbl[] []
              # "Rebundling PID Parameters without Names\nbut it should work the same"
              # "Optimized Interpolated"
              n375 = Array Size(array=w898) -> (size(s)=w912:i32)
              n376 = for {
                N: w912 -> [_]
                tunnel: w899 -> [w928]
                shift-right: [w926] -> w909
                shift-left: dbl[] [] -> [w927]
                tunnel: [w928] -> w902
                shift-right: [w924] -> w906
                shift-left: w910 -> [w925]
                shift-right: [w922] -> w908
                shift-left: w910 -> [w921]
                shift-right: [w923] -> w901
                shift-left: w910 -> [w920]
                tunnel: w898 -> [w919]
                i -> [w929]
                n377 = Index Array(array=w919, index=w929) -> (element=w918:T7)
                n378 = Unbundle(w918) -> ("PID gains"=w916:T1, "max value"=w917:dbl)
                n379 = Unbundle(w916) -> ("proportional gain (Kc)"=w913:dbl, "integral time (Ti, min)"=w915:dbl, "derivative time (Td, min)"=w914:dbl)
                n380 = Build Array (concatenate)(w927, w917) -> (w926:dbl[])
                n381 = Build Array (concatenate)(w925, w913) -> (w924:dbl[])
                n382 = Build Array (concatenate)(w921, w915) -> (w922:dbl[])
                n383 = Build Array (concatenate)(w920, w914) -> (w923:dbl[])
              }
              n384 = Threshold 1D Array(2:w902, 3:w909) -> (0:w907:dbl)  [unwired: 1 in]
              n385 = Interpolate 1D Array(1:w907, 2:w906) -> (0:w905:dbl)
              n386 = Interpolate 1D Array(1:w907, 2:w908) -> (0:w904:dbl)
              n387 = Interpolate 1D Array(1:w907, 2:w901) -> (0:w903:dbl)
              n388 = Bundle(w905, w904, w903) -> (w900:cluster{dbl, dbl, dbl})  [unwired: 1 in]
            }
            frame 1 {
              w942 = dbl[] []
              # "Rebundling PID Parameters without Names\nbut it should work the same"
              # "Minimum Interpolated"
              n389 = Array Size(array=w930) -> (size(s)=w944:i32)
              n390 = for {
                N: w944 -> [_]
                tunnel: w931 -> [w960]
                shift-right: [w958] -> w941
                shift-left: dbl[] [] -> [w959]
                tunnel: [w960] -> w934
                shift-right: [w956] -> w938
                shift-left: w942 -> [w957]
                shift-right: [w954] -> w940
                shift-left: w942 -> [w953]
                shift-right: [w955] -> w933
                shift-left: w942 -> [w952]
                tunnel: w930 -> [w951]
                i -> [w961]
                n391 = Index Array(array=w951, index=w961) -> (element=w950:T7)
                n392 = Unbundle(w950) -> ("PID gains"=w948:T1, "max value"=w949:dbl)
                n393 = Unbundle(w948) -> ("proportional gain (Kc)"=w945:dbl, "integral time (Ti, min)"=w947:dbl, "derivative time (Td, min)"=w946:dbl)
                n394 = Build Array (concatenate)(w959, w949) -> (w958:dbl[])
                n395 = Build Array (concatenate)(w957, w945) -> (w956:dbl[])
                n396 = Build Array (concatenate)(w953, w947) -> (w954:dbl[])
                n397 = Build Array (concatenate)(w952, w946) -> (w955:dbl[])
              }
              n398 = Threshold 1D Array(2:w934, 3:w941) -> (0:w939:dbl)  [unwired: 1 in]
              n399 = Interpolate 1D Array(1:w939, 2:w938) -> (0:w937:dbl)
              n400 = Interpolate 1D Array(1:w939, 2:w940) -> (0:w936:dbl)
              n401 = Interpolate 1D Array(1:w939, 2:w933) -> (0:w935:dbl)
              n402 = Bundle(w937, w936, w935) -> (w932:cluster{dbl, dbl, dbl})  [unwired: 1 in]
            }
            frame 2 {
              w974 = dbl[] []
              # "Average Interpolated"
              n403 = Array Size(array=w963) -> (size(s)=w976:i32)
              n404 = for {
                N: w976 -> [_]
                tunnel: w963 -> [w1004]
                shift-right: [w1000] -> w972
                shift-left: dbl[] [] -> [w1001]
                shift-right: [w998] -> w969
                shift-left: w974 -> [w999]
                shift-right: [w996] -> w970
                shift-left: w974 -> [w995]
                shift-right: [w997] -> w971
                shift-left: w974 -> [w994]
                tunnel: w964 -> [w991]
                i -> [w990]
                n405 = Index Array(array=w1004, index=w990) -> (element=w1003:T7)
                n406 = Index Array(array=w991, index=w990) -> (element=w993:T7)
                n407 = Unbundle(w1003) -> ("PID gains"=w1002:T1)  [unwired: 1 out]
                n408 = Unbundle(w993) -> ("PID gains"=w989:T1, "max value"=w992:dbl)
                n409 = Unbundle(w1002) -> ("proportional gain (Kc)"=w987:dbl, "integral time (Ti, min)"=w983:dbl, "derivative time (Td, min)"=w981:dbl)
                n410 = Build Array (concatenate) "Flux Cutoff"(w1001, w992) -> (w1000:dbl[])
                n411 = Unbundle(w989) -> ("proportional gain (Kc)"=w988:dbl, "integral time (Ti, min)"=w982:dbl, "derivative time (Td, min)"=w978:dbl)
                n412 = Build Array(w987, w988) -> (w986:dbl[])
                n413 = Build Array(w983, w982) -> (w985:dbl[])
                n414 = call-poly <vilib>:"Mean.vi"("X"=w986) -> ("mean"=w977:dbl)  [unwired: 1 out]
                n415 = Build Array(w981, w978) -> (w984:dbl[])
                n416 = call-poly <vilib>:"Mean.vi"("X"=w985) -> ("mean"=w980:dbl)  [unwired: 1 out]
                n417 = call-poly <vilib>:"Mean.vi"("X"=w984) -> ("mean"=w979:dbl)  [unwired: 1 out]
                n418 = Build Array (concatenate) "K_c"(w999, w977) -> (w998:dbl[])
                n419 = Build Array (concatenate) "T_i"(w995, w980) -> (w996:dbl[])
                n420 = Build Array (concatenate) "T_d"(w994, w979) -> (w997:dbl[])
              }
              n421 = Threshold 1D Array(2:w962, 3:w972) -> (0:w973:dbl)  [unwired: 1 in]
              n422 = Interpolate 1D Array(1:w973, 2:w969) -> (0:w968:dbl)
              n423 = Interpolate 1D Array(1:w973, 2:w970) -> (0:w967:dbl)
              n424 = Interpolate 1D Array(1:w973, 2:w971) -> (0:w965:dbl)
              n425 = Bundle(w968, w967, w965) -> (w966:cluster{dbl, dbl, dbl})  [unwired: 1 in]
            }
            frame 3 {
              w1017 = dbl[] []
              # "Maximum Interpolated"
              # "Rebundling PID Parameters without Names\nbut it should work the same"
              n426 = Array Size(array=w1005) -> (size(s)=w1019:i32)
              n427 = for {
                N: w1019 -> [_]
                tunnel: w1006 -> [w1035]
                shift-right: [w1033] -> w1016
                shift-left: dbl[] [] -> [w1034]
                tunnel: [w1035] -> w1009
                shift-right: [w1031] -> w1013
                shift-left: w1017 -> [w1032]
                shift-right: [w1029] -> w1015
                shift-left: w1017 -> [w1028]
                shift-right: [w1030] -> w1008
                shift-left: w1017 -> [w1027]
                tunnel: w1005 -> [w1026]
                i -> [w1036]
                n428 = Index Array(array=w1026, index=w1036) -> (element=w1025:T7)
                n429 = Unbundle(w1025) -> ("PID gains"=w1023:T1, "max value"=w1024:dbl)
                n430 = Unbundle(w1023) -> ("proportional gain (Kc)"=w1020:dbl, "integral time (Ti, min)"=w1022:dbl, "derivative time (Td, min)"=w1021:dbl)
                n431 = Build Array (concatenate)(w1034, w1024) -> (w1033:dbl[])
                n432 = Build Array (concatenate)(w1032, w1020) -> (w1031:dbl[])
                n433 = Build Array (concatenate)(w1028, w1022) -> (w1029:dbl[])
                n434 = Build Array (concatenate)(w1027, w1021) -> (w1030:dbl[])
              }
              n435 = Threshold 1D Array(2:w1009, 3:w1016) -> (0:w1014:dbl)  [unwired: 1 in]
              n436 = Interpolate 1D Array(1:w1014, 2:w1013) -> (0:w1012:dbl)
              n437 = Interpolate 1D Array(1:w1014, 2:w1015) -> (0:w1011:dbl)
              n438 = Interpolate 1D Array(1:w1014, 2:w1008) -> (0:w1010:dbl)
              n439 = Bundle(w1012, w1011, w1010) -> (w1007:cluster{dbl, dbl, dbl})  [unwired: 1 in]
            }
          }
        }
        frame 1 {
          # "Fixed Schedule"
          n440 = case "PID Paramter Aggressiveness" shown="2" w1038 {
            tunnel: [w1045 w1048 w1052 w1069] -> w1042
            tunnel: w1041 -> [_ _ w1050 w1068]
            tunnel: w1040 -> [w1044 w1047 w1049 w1067]
            tunnel: w1039 -> [_ w1046 w1051 _]
            tunnel: w1037 -> [w1043 _ _ _]
            frame 0, Default {
              # "Optimized Fixed"
              n441 = call-poly <vilib>:"PID Gain Schedule.vi"("PID gain schedule"=w1043, "gain scheduling value"=w1044) -> ("PID gains out"=w1045:T1)  [unwired: 2 in, 1 out]
            }
            frame 1 {
              # "Minimum Fixed"
              n442 = call-poly <vilib>:"PID Gain Schedule.vi"("PID gain schedule"=w1046, "gain scheduling value"=w1047) -> ("PID gains out"=w1048:T1)  [unwired: 2 in, 1 out]
            }
            frame 2 {
              # "Averaged Fixed"
              n443 = call-poly <vilib>:"PID Gain Schedule.vi"("PID gain schedule"=w1051, "gain scheduling value"=w1049) -> ("PID gains out"=w1057:T1)  [unwired: 2 in, 1 out]
              n444 = call-poly <vilib>:"PID Gain Schedule.vi"("PID gain schedule"=w1050, "gain scheduling value"=w1049) -> ("PID gains out"=w1056:T1)  [unwired: 2 in, 1 out]
              n445 = Unbundle(w1057) -> ("proportional gain (Kc)"=w1065:dbl, "integral time (Ti, min)"=w1061:dbl, "derivative time (Td, min)"=w1059:dbl)
              n446 = Unbundle(w1056) -> ("proportional gain (Kc)"=w1066:dbl, "integral time (Ti, min)"=w1060:dbl, "derivative time (Td, min)"=w1058:dbl)
              n447 = Build Array(w1065, w1066) -> (w1064:dbl[])
              n448 = Build Array(w1061, w1060) -> (w1063:dbl[])
              n449 = call-poly <vilib>:"Mean.vi"("X"=w1064) -> ("mean"=w1053:dbl)  [unwired: 1 out]
              n450 = Build Array(w1059, w1058) -> (w1062:dbl[])
              n451 = call-poly <vilib>:"Mean.vi"("X"=w1063) -> ("mean"=w1055:dbl)  [unwired: 1 out]
              n452 = call-poly <vilib>:"Mean.vi"("X"=w1062) -> ("mean"=w1054:dbl)  [unwired: 1 out]
              n453 = Bundle("mean"=w1053, "mean"=w1055, "mean"=w1054) -> (w1052:cluster{"mean":dbl, "mean":dbl, "mean":dbl})  [unwired: 1 in]
            }
            frame 3 {
              # "Maximum Fixed"
              n454 = call-poly <vilib>:"PID Gain Schedule.vi"("PID gain schedule"=w1068, "gain scheduling value"=w1067) -> ("PID gains out"=w1069:T1)  [unwired: 2 in, 1 out]
            }
          }
        }
      }
      "Suggested PID gains OFF" <- w843
      n455 = case "ON Flux PID Gain Parameters: Interpolated vs. Fixed" shown="1" w849 {
        tunnel: w825 -> [w1072 w1217]
        tunnel: [w1074 w1219] -> w844
        tunnel: w848 -> [w1075 w1220]
        tunnel: w853 -> [w1073 w1216]
        tunnel: w852 -> [w1071 w1218]
        tunnel: w842 -> [w1070 w1215]
        frame 0, Default {
          # "Interpolated Schedule"
          n456 = case "PID Paramter Aggressiveness" shown="0, Default" w1075 {
            tunnel: [w1078 w1110 w1144 w1185] -> w1074
            tunnel: w1073 -> [_ w1108 w1141 _]
            tunnel: w1072 -> [w1077 w1109 w1140 w1184]
            tunnel: w1071 -> [_ _ w1142 w1183]
            tunnel: w1070 -> [w1076 _ _ _]
            frame 0, Default {
              w1088 = dbl[] []
              # "Rebundling PID Parameters without Names\nbut it should work the same"
              # "Optimized Interpolated"
              n457 = Array Size(array=w1076) -> (size(s)=w1090:i32)
              n458 = for {
                N: w1090 -> [_]
                tunnel: w1077 -> [w1106]
                shift-right: [w1104] -> w1087
                shift-left: dbl[] [] -> [w1105]
                tunnel: [w1106] -> w1080
                shift-right: [w1102] -> w1084
                shift-left: w1088 -> [w1103]
                shift-right: [w1100] -> w1086
                shift-left: w1088 -> [w1099]
                shift-right: [w1101] -> w1079
                shift-left: w1088 -> [w1098]
                tunnel: w1076 -> [w1097]
                i -> [w1107]
                n459 = Index Array(array=w1097, index=w1107) -> (element=w1096:T7)
                n460 = Unbundle(w1096) -> ("PID gains"=w1094:T1, "max value"=w1095:dbl)
                n461 = Unbundle(w1094) -> ("proportional gain (Kc)"=w1091:dbl, "integral time (Ti, min)"=w1093:dbl, "derivative time (Td, min)"=w1092:dbl)
                n462 = Build Array (concatenate)(w1105, w1095) -> (w1104:dbl[])
                n463 = Build Array (concatenate)(w1103, w1091) -> (w1102:dbl[])
                n464 = Build Array (concatenate)(w1099, w1093) -> (w1100:dbl[])
                n465 = Build Array (concatenate)(w1098, w1092) -> (w1101:dbl[])
              }
              n466 = Threshold 1D Array(2:w1080, 3:w1087) -> (0:w1085:dbl)  [unwired: 1 in]
              n467 = Interpolate 1D Array(1:w1085, 2:w1084) -> (0:w1083:dbl)
              n468 = Interpolate 1D Array(1:w1085, 2:w1086) -> (0:w1082:dbl)
              n469 = Interpolate 1D Array(1:w1085, 2:w1079) -> (0:w1081:dbl)
              n470 = Bundle(w1083, w1082, w1081) -> (w1078:cluster{dbl, dbl, dbl})  [unwired: 1 in]
            }
            frame 1 {
              w1120 = dbl[] []
              # "Rebundling PID Parameters without Names\nbut it should work the same"
              # "Minimum Interpolated"
              n471 = Array Size(array=w1108) -> (size(s)=w1122:i32)
              n472 = for {
                N: w1122 -> [_]
                tunnel: w1109 -> [w1138]
                shift-right: [w1136] -> w1119
                shift-left: dbl[] [] -> [w1137]
                tunnel: [w1138] -> w1112
                shift-right: [w1134] -> w1116
                shift-left: w1120 -> [w1135]
                shift-right: [w1132] -> w1118
                shift-left: w1120 -> [w1131]
                shift-right: [w1133] -> w1111
                shift-left: w1120 -> [w1130]
                tunnel: w1108 -> [w1129]
                i -> [w1139]
                n473 = Index Array(array=w1129, index=w1139) -> (element=w1128:T7)
                n474 = Unbundle(w1128) -> ("PID gains"=w1126:T1, "max value"=w1127:dbl)
                n475 = Unbundle(w1126) -> ("proportional gain (Kc)"=w1123:dbl, "integral time (Ti, min)"=w1125:dbl, "derivative time (Td, min)"=w1124:dbl)
                n476 = Build Array (concatenate)(w1137, w1127) -> (w1136:dbl[])
                n477 = Build Array (concatenate)(w1135, w1123) -> (w1134:dbl[])
                n478 = Build Array (concatenate)(w1131, w1125) -> (w1132:dbl[])
                n479 = Build Array (concatenate)(w1130, w1124) -> (w1133:dbl[])
              }
              n480 = Threshold 1D Array(2:w1112, 3:w1119) -> (0:w1117:dbl)  [unwired: 1 in]
              n481 = Interpolate 1D Array(1:w1117, 2:w1116) -> (0:w1115:dbl)
              n482 = Interpolate 1D Array(1:w1117, 2:w1118) -> (0:w1114:dbl)
              n483 = Interpolate 1D Array(1:w1117, 2:w1111) -> (0:w1113:dbl)
              n484 = Bundle(w1115, w1114, w1113) -> (w1110:cluster{dbl, dbl, dbl})  [unwired: 1 in]
            }
            frame 2 {
              w1152 = dbl[] []
              # "Average Interpolated"
              n485 = Array Size(array=w1141) -> (size(s)=w1154:i32)
              n486 = for {
                N: w1154 -> [_]
                tunnel: w1141 -> [w1182]
                shift-right: [w1178] -> w1150
                shift-left: dbl[] [] -> [w1179]
                shift-right: [w1176] -> w1147
                shift-left: w1152 -> [w1177]
                shift-right: [w1174] -> w1148
                shift-left: w1152 -> [w1173]
                shift-right: [w1175] -> w1149
                shift-left: w1152 -> [w1172]
                tunnel: w1142 -> [w1169]
                i -> [w1168]
                n487 = Index Array(array=w1182, index=w1168) -> (element=w1181:T7)
                n488 = Index Array(array=w1169, index=w1168) -> (element=w1171:T7)
                n489 = Unbundle(w1181) -> ("PID gains"=w1180:T1)  [unwired: 1 out]
                n490 = Unbundle(w1171) -> ("PID gains"=w1167:T1, "max value"=w1170:dbl)
                n491 = Unbundle(w1180) -> ("proportional gain (Kc)"=w1165:dbl, "integral time (Ti, min)"=w1161:dbl, "derivative time (Td, min)"=w1159:dbl)
                n492 = Build Array (concatenate) "Flux Cutoff"(w1179, w1170) -> (w1178:dbl[])
                n493 = Unbundle(w1167) -> ("proportional gain (Kc)"=w1166:dbl, "integral time (Ti, min)"=w1160:dbl, "derivative time (Td, min)"=w1156:dbl)
                n494 = Build Array(w1165, w1166) -> (w1164:dbl[])
                n495 = Build Array(w1161, w1160) -> (w1163:dbl[])
                n496 = call-poly <vilib>:"Mean.vi"("X"=w1164) -> ("mean"=w1155:dbl)  [unwired: 1 out]
                n497 = Build Array(w1159, w1156) -> (w1162:dbl[])
                n498 = call-poly <vilib>:"Mean.vi"("X"=w1163) -> ("mean"=w1158:dbl)  [unwired: 1 out]
                n499 = call-poly <vilib>:"Mean.vi"("X"=w1162) -> ("mean"=w1157:dbl)  [unwired: 1 out]
                n500 = Build Array (concatenate) "K_c"(w1177, w1155) -> (w1176:dbl[])
                n501 = Build Array (concatenate) "T_i"(w1173, w1158) -> (w1174:dbl[])
                n502 = Build Array (concatenate) "T_d"(w1172, w1157) -> (w1175:dbl[])
              }
              n503 = Threshold 1D Array(2:w1140, 3:w1150) -> (0:w1151:dbl)  [unwired: 1 in]
              n504 = Interpolate 1D Array(1:w1151, 2:w1147) -> (0:w1146:dbl)
              n505 = Interpolate 1D Array(1:w1151, 2:w1148) -> (0:w1145:dbl)
              n506 = Interpolate 1D Array(1:w1151, 2:w1149) -> (0:w1143:dbl)
              n507 = Bundle(w1146, w1145, w1143) -> (w1144:cluster{dbl, dbl, dbl})  [unwired: 1 in]
            }
            frame 3 {
              w1195 = dbl[] []
              # "Maximum Interpolated"
              # "Rebundling PID Parameters without Names\nbut it should work the same"
              n508 = Array Size(array=w1183) -> (size(s)=w1197:i32)
              n509 = for {
                N: w1197 -> [_]
                tunnel: w1184 -> [w1213]
                shift-right: [w1211] -> w1194
                shift-left: dbl[] [] -> [w1212]
                tunnel: [w1213] -> w1187
                shift-right: [w1209] -> w1191
                shift-left: w1195 -> [w1210]
                shift-right: [w1207] -> w1193
                shift-left: w1195 -> [w1206]
                shift-right: [w1208] -> w1186
                shift-left: w1195 -> [w1205]
                tunnel: w1183 -> [w1204]
                i -> [w1214]
                n510 = Index Array(array=w1204, index=w1214) -> (element=w1203:T7)
                n511 = Unbundle(w1203) -> ("PID gains"=w1201:T1, "max value"=w1202:dbl)
                n512 = Unbundle(w1201) -> ("proportional gain (Kc)"=w1198:dbl, "integral time (Ti, min)"=w1200:dbl, "derivative time (Td, min)"=w1199:dbl)
                n513 = Build Array (concatenate)(w1212, w1202) -> (w1211:dbl[])
                n514 = Build Array (concatenate)(w1210, w1198) -> (w1209:dbl[])
                n515 = Build Array (concatenate)(w1206, w1200) -> (w1207:dbl[])
                n516 = Build Array (concatenate)(w1205, w1199) -> (w1208:dbl[])
              }
              n517 = Threshold 1D Array(2:w1187, 3:w1194) -> (0:w1192:dbl)  [unwired: 1 in]
              n518 = Interpolate 1D Array(1:w1192, 2:w1191) -> (0:w1190:dbl)
              n519 = Interpolate 1D Array(1:w1192, 2:w1193) -> (0:w1189:dbl)
              n520 = Interpolate 1D Array(1:w1192, 2:w1186) -> (0:w1188:dbl)
              n521 = Bundle(w1190, w1189, w1188) -> (w1185:cluster{dbl, dbl, dbl})  [unwired: 1 in]
            }
          }
        }
        frame 1 {
          # "Fixed Schedule"
          n522 = case "PID Paramter Aggressiveness" shown="2" w1220 {
            tunnel: [w1221 w1226 w1230 w1247] -> w1219
            tunnel: w1218 -> [_ _ w1227 w1246]
            tunnel: w1217 -> [w1222 w1225 w1228 w1245]
            tunnel: w1216 -> [_ w1224 w1229 _]
            tunnel: w1215 -> [w1223 _ _ _]
            frame 0 {
              # "Optimized Fixed"
              n523 = call-poly <vilib>:"PID Gain Schedule.vi"("PID gain schedule"=w1223, "gain scheduling value"=w1222) -> ("PID gains out"=w1221:T1)  [unwired: 2 in, 1 out]
            }
            frame 1, Default {
              # "Minimum Fixed"
              n524 = call-poly <vilib>:"PID Gain Schedule.vi"("PID gain schedule"=w1224, "gain scheduling value"=w1225) -> ("PID gains out"=w1226:T1)  [unwired: 2 in, 1 out]
            }
            frame 2 {
              # "Averaged Fixed"
              n525 = call-poly <vilib>:"PID Gain Schedule.vi"("PID gain schedule"=w1229, "gain scheduling value"=w1228) -> ("PID gains out"=w1235:T1)  [unwired: 2 in, 1 out]
              n526 = call-poly <vilib>:"PID Gain Schedule.vi"("PID gain schedule"=w1227, "gain scheduling value"=w1228) -> ("PID gains out"=w1234:T1)  [unwired: 2 in, 1 out]
              n527 = Unbundle(w1235) -> ("proportional gain (Kc)"=w1243:dbl, "integral time (Ti, min)"=w1239:dbl, "derivative time (Td, min)"=w1237:dbl)
              n528 = Unbundle(w1234) -> ("proportional gain (Kc)"=w1244:dbl, "integral time (Ti, min)"=w1238:dbl, "derivative time (Td, min)"=w1236:dbl)
              n529 = Build Array(w1243, w1244) -> (w1242:dbl[])
              n530 = Build Array(w1239, w1238) -> (w1241:dbl[])
              n531 = call-poly <vilib>:"Mean.vi"("X"=w1242) -> ("mean"=w1231:dbl)  [unwired: 1 out]
              n532 = Build Array(w1237, w1236) -> (w1240:dbl[])
              n533 = call-poly <vilib>:"Mean.vi"("X"=w1241) -> ("mean"=w1233:dbl)  [unwired: 1 out]
              n534 = call-poly <vilib>:"Mean.vi"("X"=w1240) -> ("mean"=w1232:dbl)  [unwired: 1 out]
              n535 = Bundle("mean"=w1231, "mean"=w1233, "mean"=w1232) -> (w1230:cluster{"mean":dbl, "mean":dbl, "mean":dbl})  [unwired: 1 in]
            }
            frame 3 {
              # "Maximum Fixed"
              n536 = call-poly <vilib>:"PID Gain Schedule.vi"("PID gain schedule"=w1246, "gain scheduling value"=w1245) -> ("PID gains out"=w1247:T1)  [unwired: 2 in, 1 out]
            }
          }
        }
      }
      "Suggested PID gains ON" <- w844
      n537 = Array Subset(array=w818, index=w822, length=1) -> (w821:dbl[])
      n538 = Delete From Array "Last Point\n AO (V)"(array=w821) -> (deleted portion=w820:dbl)  [unwired: 2 in, 1 out]
      "Final AO (V)" <- w820
      n539 = shared-variable "NI-GenericDesktopPC-3A84958E\\Kopco PS Project Target Variables Library.lvlib\\FinalAOV"(w820) -> ()  [unwired: 1 in, 1 out]
      n540 = shared-variable "NI-GenericDesktopPC-3A84958E\\Kopco PS Project Target Variables Library.lvlib\\Digital Trigger"() -> (w828:bool)  [unwired: 1 in, 1 out]
      n541 = shared-variable "NI-GenericDesktopPC-3A84958E\\Kopco PS Project Target Variables Library.lvlib\\Data Upload"() -> (w827:bool)  [unwired: 1 in, 1 out]
      n542 = case shown="True" w828 {
        frame False {
        }
        frame True {
          n543 = shared-variable "NI-GenericDesktopPC-3A84958E\\Kopco PS Project Target Variables Library.lvlib\\Digital Trigger"(FALSE ("Digital Trigger")) -> ()  [unwired: 1 in, 1 out]
        }
      }
      n544 = case shown="True" w827 {
        frame False {
        }
        frame True {
          n545 = shared-variable "NI-GenericDesktopPC-3A84958E\\Kopco PS Project Target Variables Library.lvlib\\Data Upload"(FALSE ("Digital Trigger")) -> ()  [unwired: 1 in, 1 out]
        }
      }
    }
    frame #17 {
      # "Bound to \"PID Parameters Selected\"\nshared global variable"
      # "Bound to \"Data Logger Running\"\nshared global variable."
      # "Flux ON/OFF Logical"
      # "AO values of current"
      # "Sampling Rate"
      # "Flux Control Sequence"
      # "Mini DeGauss AO Sequence, Normalized"
      # "Mini DeGauss Logical"
      # "Ask if you want to tweak the current parameters. This is useful in \ninterpolation cases, and when values change over time"
      # "Step 4 Specifying PID Parameters"
      n546 = flat-sequence {
        tunnel: w1261 -> [w1266]
        tunnel: w1262 -> [w1269]
        tunnel: [w1270] -> w1259
        tunnel: [w1268] -> w1251
        tunnel: [w1267] -> w1250
        tunnel: [w1280] -> w1260
        tunnel: [w1278] -> w1258
        tunnel: [w1277] -> w1257
        tunnel: w1259 -> [w1276]
        tunnel: w1251 -> [w1279]
        tunnel: w1250 -> [w1275]
        frame #0 {
          n547 = while {
            tunnel: ["Start Null Flux Adjustment 2"] -> _
            tunnel: ["Keep Null Flux Running \n       Until Next Step? 2"] -> w1270
            tunnel: w1269 -> [w1272]
            tunnel: [w1272] -> w1268
            tunnel: [w1271] -> w1267
            tunnel: w1266 -> [w1271]
            stop <- "Start Null Flux Adjustment 2" stop-if-true
          }
        }
        frame #1 {
          n548 = case shown="False" w1276 {
            tunnel: [TRUE TRUE] -> w1280
            tunnel: w1279 -> [w1281 _]
            tunnel: [w1281 "Tweaked PID gains ON"] -> w1278
            tunnel: [w1282 "Tweaked PID gains OFF"] -> w1277
            tunnel: w1275 -> [w1282 _]
            frame False {
              # "No Change in PID Parameters"
            }
            frame True {
            }
          }
        }
      }
      n549 = shared-variable "NI-GenericDesktopPC-3A84958E\\Kopco PS Project Target Variables Library.lvlib\\PID Parameters Selected"(w1260) -> ()  [unwired: 1 in, 1 out]
      "PID gains ON Chosen" <- w1258
      "PID gains OFF Chosen" <- w1257
    }
    frame #18 {
      w1312 = -1 items=["default"=-1, "RSE"=10083, "NRSE"=10078, "Differential"=10106, "Pseudodifferential"=12529] ("Terminal Configuration")
      w1317 = "Dev2/ao0"  # Power Supply Control
      w1316 = 12522 items=["Finite Samples"=10178, "Continuous Samples"=10123, "Hardware Timed Single Point"=12522]  # Sample Mode
      w1322 = 10106 items=["default"=-1, "RSE"=10083, "NRSE"=10078, "Differential"=10106, "Pseudodifferential"=12529] ("Terminal Configuration")
      w1325 = 12522 items=["Finite Samples"=10178, "Continuous Samples"=10123, "Hardware Timed Single Point"=12522]  # Sample Mode
      # "1/4 wave to get the main points of the\n mini DeGauss waveform 3/12/2018"
      # "Reversed order of AI7 & AI3 on 4/11/2018 to \nminimize leakage to Channel 7"
      # "# of samples of Mini DeGauss"
      # "Fixed by WIM on 3/5/2018 to keep the old AO value"
      # "Step 5 Preparing DAQ for Waveform"
      # "Total Number of Samples"
      n550 = shared-variable "NI-GenericDesktopPC-3A84958E\\Kopco PS Project Target Variables Library.lvlib\\Channels AI List"() -> (w1288:string)  [unwired: 1 in, 1 out]
      n551 = shared-variable "NI-GenericDesktopPC-3A84958E\\Kopco PS Project Target Variables Library.lvlib\\Sampling Rate"() -> (w1287:dbl)  [unwired: 1 in, 1 out]
      n552 = call-poly <vilib>:"DAQmx Create Virtual Channel.vi"("maximum value"=5.0 ("Max Voltage"), "minimum value"=0.0 ("Min Voltage"), "input terminal configuration"=w1322, "physical channels"=w1288) -> ("task out"=w1323:refnum<k21>, "error out"=w1324:errorcluster)  [unwired: 10 in]
      n553 = call-poly <vilib>:"DAQmx Create Virtual Channel.vi"("maximum value"=10.0, "minimum value"=-10.0, "output terminal configuration"=w1312, "physical channels"=w1317) -> ("task out"=w1319:refnum<k21>, "error out"=w1318:errorcluster)  [unwired: 10 in]
      n554 = shared-variable "NI-GenericDesktopPC-3A84958E\\Kopco PS Project Target Variables Library.lvlib\\Zero Flux Calibrated Core"() -> (w1302:dbl)  [unwired: 1 in, 1 out]
      n555 = call-poly <vilib>:"DAQmx Timing.vi"("task/channels in"=w1323, "sample mode"=w1325, "rate"=w1287, "error in"=w1324) -> ("task out"=w1315:refnum<k21>, "error out"=w1311:errorcluster)  [unwired: 10 in]
      n556 = call "Get Terminal Name with Device Prefix.vi"("error in"=w1311, "Local Terminal Name"="ai/SampleClock", "task/channels in"=w1315) -> ("error out"=w1304:errorcluster, "Terminal Name with Device Prefix"=w1310:tag, "task out"=w1305:refnum<k21>)  [unwired: 6 in]
      n557 = call-poly <vilib>:"DAQmx Timing.vi"("task/channels in"=w1319, "sample mode"=w1316, "rate"=w1287, "source"=w1310, "error in"=w1318) -> ("task out"=w1307:refnum<k21>, "error out"=w1308:errorcluster)  [unwired: 9 in]
      n558 = call <vilib>:"DAQmx Start Task.vi"("task/channels in"=w1307, "error in"=w1308) -> ("task out"=w1298:refnum<k21>, "error out"=w1297:errorcluster)  [unwired: 12 in]
      n559 = Merge Errors(w1304, w1297) -> (w1306:errorcluster)
    }
    frame #19 {
      # "1/4 wave to get the main points of the mini DeGauss waveform 3/12/2018"
      n560 = while "Digital Trigger from Master Data Logger" {
        tunnel: [w1374] -> w1356
        tunnel: w1357 -> [w1374]
        tunnel: w1355 -> [w1373]
        tunnel: [w1373] -> w1354
        tunnel: w1353 -> [w1372]
        tunnel: [w1372] -> w1352
        tunnel: [w1371] -> w1351
        tunnel: w1350 -> [w1371]
        tunnel: w1349 -> [w1370]
        tunnel: [w1370] -> w1348
        tunnel: w1347 -> [w1369]
        tunnel: [w1369] -> w1346
        tunnel: w1345 -> [w1368]
        tunnel: [w1368] -> w1344
        tunnel: w1343 -> [w1367]
        tunnel: [w1367] -> w1342
        tunnel: w1341 -> [w1366]
        tunnel: [w1366] -> w1340
        tunnel: w1339 -> [w1365]
        tunnel: [w1365] -> w1338
        tunnel: w1337 -> [w1364]
        tunnel: [w1364] -> w1336
        tunnel: w1335 -> [w1363]
        tunnel: [w1363] -> w1334
        tunnel: w1333 -> [w1362]
        tunnel: [w1362] -> w1332
        tunnel: w1331 -> [w1361]
        tunnel: [w1361] -> w1330
        tunnel: w1329 -> [w1358]
        tunnel: w1328 -> [w1359]
        tunnel: [w1359] -> w1327
        tunnel: [w1358] -> w1326
        stop <- w1375 stop-if-true
        # "Bound to Digital Trigger Real-Time Shared Variable"
        n561 = shared-variable "NI-GenericDesktopPC-3A84958E\\Kopco PS Project Target Variables Library.lvlib\\Digital Trigger"() -> (w1375:bool)  [unwired: 1 in, 1 out]
        "DigitalTrigger" <- w1375
        n562 = Wait (ms)(milliseconds to wait=u32 1) -> ()  [unwired: 1 out]
      }
    }
    frame #20 {
      w1391 = 0  # Last Current AO Index
      w1396 = 0  # 0-14 Mini DeGauss Sample Counter Initialized
      w1415 = T8 1 items=["All Elements Read From Stream", "All Elements Available for Reading"] ("wait condition")
      w1395 = 30  # # of samples pushed  to PID loop
      w1439 = 0  # 0-29 PID Sample Counter Initialized
      # "Reset Digital trigger in case program gets stuck"
      # "Moved Outside 3/31/2018"
      # "# of samples of Mini DeGauss"
      # "Bound to \"DataUpload\" shared variable"
      # "Abs(AO_nf) + Abs(AO_on,last)"
      # "AO_Last"
      # "Set PID \nReinitialize as true\ninitialially"
      # "Mini DeGauss AO Sequence, Normalized"
      # "Mini DeGauss PID CTRL ON/OFF Logical"
      # "AO,last"
      # "Step 5 Pushing Data to Datalogger"
      # "Step 5 Carrying out Waveform"
      # "ON PID Gain"
      # "OFF PID Gains"
      # "Flux ON/OFF CTRL Setpoint Sequence Logical"
      # "Increased buffer size to 100Mil on 1/1/2018"
      # "For 2 minutes"
      # "Calibrated Zero"
      # "PID Sampling interval, dt"
      # "Total Number of Samples"
      # "Note 1: Even though the parameters can be\nbrought into the loop \nand changed in real time. We want to avoid this\nNote 2: These parameters are for control in the linear range 0-175 GS absolute.\nFor non-linear range, you will need PID Gain Scheduling VI"
      # "Sample Rate (Hz or s^-1)\nor Step Duration (Each step is one second)"
      # "Offset by 1 removed \non 8/3/2017.\nIt solved problem. All\nData is there!"
      # "PS does not turn off unless two values are written."
      # "Maybe use it to replace the last value?"
      # "Removed Digital Trigger DAQmx and replaced\nwith real-time global variable before that"
      # "Flux Control Setpoint Sequence"
      n563 = shared-variable "NI-GenericDesktopPC-3A84958E\\Kopco PS Project Target Variables Library.lvlib\\Digital Trigger"(FALSE ("DigitalTrigger")) -> ()  [unwired: 1 in, 1 out]
      n564 = Unbundle(w1405) -> ("proportional gain (Kc)"=w1404:dbl, "integral time (Ti, min)"=w1403:dbl, "derivative time (Td, min)"=w1402:dbl)
      n565 = Build Array "PID Parameters OFF"(w1404, w1403, w1402) -> (w1406:dbl[])
      n566 = Unbundle(w1400) -> ("proportional gain (Kc)"=w1434:dbl, "integral time (Ti, min)"=w1433:dbl, "derivative time (Td, min)"=w1432:dbl)
      n567 = Build Array "PID Parameters ON"(w1434, w1433, w1432, w1395, w1398) -> (w1431:dbl[])
      n568 = Reciprocal "Sample interval"(x=w1398) -> (1/x=w1435:dbl)
      n569 = shared-variable "NI-GenericDesktopPC-3A84958E\\Kopco PS Project Target Variables Library.lvlib\\PID Parameters OFF"(w1406) -> ()  [unwired: 1 in, 1 out]
      n570 = shared-variable "NI-GenericDesktopPC-3A84958E\\Kopco PS Project Target Variables Library.lvlib\\PID Parameters ON"(w1431) -> ()  [unwired: 1 in, 1 out]
      n571 = call-poly <vilib>:"DAQmx Create Timing Source.vi"("task/channels in"=w1443, "sleep time (us)"=1.0, "error in"=w1444) -> ("task out"=w1410:refnum<k21>, "timing source out"=w1383:string, "error out"=w1427:errorcluster)  [unwired: 10 in]
      n572 = Multiply "PID Sampling Interval, dt"(x=w1395, y=w1435) -> (x*y=w1430:dbl)
      n573 = shared-variable "NI-GenericDesktopPC-3A84958E\\Kopco PS Project Target Variables Library.lvlib\\Sampling Rate"() -> (w1379:dbl)  [unwired: 1 in, 1 out]
      n574 = Create Network Stream Writer Endpoint(7:100000000 ("writer buffer size"), 9:0.0 ("Double"), 11:"FluxWriter" ("writer name")) -> (0:w1419:errorcluster, 3:w1418:refnum<k21>)  [unwired: 4 in]
      n575 = Initialize Array "Initialize Array\nof samples to PID"(0.0 ("sleep time (us)"), w1395) -> (w1428:dbl[])
      n576 = shared-variable "NI-GenericDesktopPC-3A84958E\\Kopco PS Project Target Variables Library.lvlib\\Sensor Sensitivity Core"() -> (w1381:dbl)  [unwired: 1 in, 1 out]
      n577 = Array Size(array=w1436) -> (size(s)=w1437:i32)
      n578 = Divide(x=w1378, y=w1379) -> (x/y=→"Total seconds":dbl)
      n579 = Subtract(x=w1437, y=0) -> (x-y=w1429:i32)
      n580 = shared-variable "NI-GenericDesktopPC-3A84958E\\Kopco PS Project Target Variables Library.lvlib\\Sensor Index Flux Core"() -> ()  [unwired: 1 in, 2 out]
      n581 = shared-variable "NI-GenericDesktopPC-3A84958E\\Kopco PS Project Target Variables Library.lvlib\\Sensor Index Camera"() -> ()  [unwired: 1 in, 2 out]
      n582 = node-c288(w1383) -> (w1424:T3)  [unwired: 3 in]
      n583 = Quotient & Remainder(x=w1395, y=2) -> (floor(x/y)=w1390:i32)  [unwired: 1 out]
      n584 = timed-loop "Lower priority deterministic Code for Data Collection to Data Logger" {
        timing: w1424 -> [_]
        timing-out: [_] -> w1423
        tunnel: w1378 -> [w1449]
        tunnel: w1419 -> [w1466]
        tunnel: [w1457] -> w1376
        tunnel: [w1464] -> w1377
        tunnel: w1418 -> [w1465]
        shift-right: [w1456] -> _
        shift-left: -1 ("y") -> [w1458]
        tunnel: [w1448] -> _
        tunnel: w1379 -> [w1455]
        i -> [w1448]
        stop <- w1447 stop-if-true
        # "Switch OFF Null Flux currently running indicator. Placed in non-deterministic loop so as not to"
        # "Using variable bound\nto the toggle generate the error message\nthat remote endpoint is destroyed."
        n585 = node-c288() -> ()  [unwired: 1 in, 1 out]
        n586 = shared-variable ".\\Kopco PS Project Target Variables Library.lvlib\\Last Current AO"() -> (w1456:dbl)  [unwired: 1 in, 1 out]
        n587 = shared-variable ".\\Kopco PS Project Target Variables Library.lvlib\\Data RT Current"() -> (w1462:dbl)  [unwired: 1 in, 1 out]
        n588 = shared-variable ".\\Kopco PS Project Target Variables Library.lvlib\\Data RT Exposure"() -> (w1461:dbl)  [unwired: 1 in, 1 out]
        n589 = shared-variable "NI-GenericDesktopPC-3A84958E\\Kopco PS Project Target Variables Library.lvlib\\Null Flux Running Middle"(FALSE ("Null Flux Running Middle")) -> ()  [unwired: 1 in, 1 out]
        n590 = shared-variable ".\\Kopco PS Project Target Variables Library.lvlib\\Data RT Flux"() -> (w1463:dbl)  [unwired: 1 in, 1 out]
        n591 = Greater?(x=w1448, y=w1458) -> ()  [unwired: 1 out]
        n592 = Greater Or Equal?(x=w1448, y=w1449) -> (x >= y?=w1447:bool)
        n593 = Build Array(w1456, w1463, w1462, w1461) -> (w1460:dbl[])
        n594 = shared-variable-write(w1465, w1466, w1460) -> (w1464:refnum<k21>, w1457:errorcluster)  [unwired: 1 in, 1 out]
        n595 = Quotient & Remainder(x=w1448, y=10000) -> (x-y*floor(x/y)=w1453:i32)  [unwired: 1 out]
        n596 = Equal To 0?(x=w1453) -> (x = 0?=w1452:bool)
        n597 = Equal?(x=w1448, y=w1449) -> (x = y?=w1450:bool)
        n598 = Or(x=w1450, y=w1452) -> (x .or. y?=w1451:bool)
        n599 = case shown="True" w1451 {
          tunnel: w1455 -> [_ w1468]
          tunnel: w1448 -> [_ w1467]
          frame False {
          }
          frame True {
            n600 = Divide(x=w1467, y=w1468) -> (x/y=→"Loop Index 2":dbl)
            "Loop Index" <- w1467
          }
        }
        n601 = Not(x=w1447) -> (.not. x?=w1446:bool)
        n602 = shared-variable ".\\Kopco PS Project Target Variables Library.lvlib\\Data Upload"(w1446) -> ()  [unwired: 1 in, 1 out]
        n603 = node-c288() -> ()  [unwired: 1 in, 1 out]
      }
      n604 = node-c288(w1383) -> (w1442:T3)  [unwired: 9 in]
      n605 = timed-loop "PID Control Loop" {
        tunnel: [w1530] -> _
        tunnel: w1440 -> [w1533]
        tunnel: [w1517] -> w1426
        tunnel: w1436 -> [w1531]
        timing: w1442 -> [_]
        timing-out: [_] -> w1441
        shift-right: [w1479] -> _
        shift-left: w1392 -> [w1510]
        shift-right: [w1528] -> _
        shift-left: w1428 -> [w1526]
        tunnel: w1428 -> [w1525]
        shift-right: [w1524] -> _
        shift-left: w1439 -> [w1523]
        tunnel: w1437 -> [w1527]
        tunnel: w1429 -> [_]
        tunnel: w1395 -> [w1508]
        tunnel: w1400 -> [w1514]
        tunnel: w1430 -> [w1520]
        tunnel: w1427 -> [w1519]
        tunnel: [w1518] -> w1413
        tunnel: [w1517] -> w1401
        tunnel: w1410 -> [w1516]
        tunnel: w1409 -> [w1515]
        tunnel: w1407 -> [w1513]
        tunnel: w1405 -> [w1512]
        tunnel: w1399 -> [w1511]
        tunnel: w1397 -> [w1509]
        shift-right: [w1506] -> _
        shift-left: w1396 -> [w1504]
        tunnel: w1390 -> [w1505]
        shift-right: [w1502] -> _
        shift-left: TRUE -> [w1501]
        tunnel: w1392 -> [w1500]
        shift-right: [w1498] -> _
        shift-left: w1392 -> [w1499]
        shift-right: [w1496] -> _
        shift-left: w1391 -> [w1497]
        tunnel: w1389 -> [w1495]
        tunnel: [w1491] -> w1387
        tunnel: TRUE ("8. Keep Final Flux Running at End?") -> [w1490]
        tunnel: w1384 -> [w1483]
        tunnel: w1382 -> [w1482]
        tunnel: w1381 -> [w1481]
        i -> [w1492]
        stop <- w1493 continue-if-true
        # "Reversed order of AI7 & AI3 on 4/11/2018 to \nminimize leakage to Channel 7"
        # "No PID Control/DeGauss\nwhen control sequence is exceeded 3/31/2018"
        # "Stop this loop once data is uploaded"
        # "Calibrated Zero"
        # "AO_Null Flux"
        # "Rewrite to AO for now to see what it actually outputs.,  3/8/2018."
        # "AO last"
        # "AO"
        # "PID Sampling interval, dt"
        # "Number of samples pushed to PID\nper time"
        # "Current Flux\nSetpoint Value"
        # "Flux AI Reading"
        # "Array size"
        n606 = node-c288() -> ()  [unwired: 1 in, 1 out]
        n607 = Index Array "Current\nFlux Setpoint"(array=w1531, index=w1492) -> (element=w1529:dbl)
        n608 = Less Or Equal? "Less than 30 Samples"(x=w1523, y=w1508) -> (x <= y?=w1485:bool)
        n609 = call-poly <vilib>:"DAQmx Read.vi"("task/channels in"=w1516, "error in"=w1519) -> ("task out"=w1530:refnum<k21>, "data"=w1522:dbl[], "error out"=w1532:errorcluster)  [unwired: 11 in]
        n610 = Less Or Equal? "Less than 15 Samples"(x=w1504, y=w1505) -> (x <= y?=w1507:bool)
        n611 = Greater Or Equal? "Exceeded Datapoints?"(x=w1492, y=w1527) -> (x >= y?=w1484:bool)
        n612 = Delete From Array "AI5 Flux \nChannel"(array=w1522, index=1) -> (deleted portion=w1521:dbl)  [unwired: 1 in, 1 out]
        n613 = Delete From Array "AI7 Exposure\n Channel"(array=w1522, index=3) -> (deleted portion=w1480:dbl)  [unwired: 1 in, 1 out]
        n614 = Index Array "Mini-DeGauss \nON/OFF Status?"(array=w1511, index=w1492) -> (element=w1489:bool)
        n615 = case "DeGauss Sequence ON/OFF?" shown="False" w1489 {
          tunnel: w1529 -> [w1568 _]
          tunnel: w1510 -> [w1567 _]
          tunnel: [w1566 w1627] -> w1528
          tunnel: w1485 -> [w1543 _]
          tunnel: w1526 -> [w1565 w1626]
          tunnel: w1525 -> [w1564 w1625]
          tunnel: [w1546 w1629] -> w1524
          tunnel: w1523 -> [w1563 _]
          tunnel: w1521 -> [w1562 _]
          tunnel: w1520 -> [w1561 _]
          tunnel: [w1547 w1623] -> w1503
          tunnel: w1515 -> [w1560 _]
          tunnel: w1492 -> [w1550 w1617]
          tunnel: w1514 -> [w1559 _]
          tunnel: w1513 -> [w1558 _]
          tunnel: w1512 -> [w1557 _]
          tunnel: w1509 -> [_ w1624]
          tunnel: w1507 -> [_ w1622]
          tunnel: [w1556 w1621] -> w1506
          tunnel: w1504 -> [_ w1620]
          tunnel: [w1554 TRUE] -> w1502
          tunnel: w1501 -> [w1555 _]
          tunnel: w1500 -> [w1553 w1618]
          tunnel: [w1550 w1614] -> w1496
          tunnel: w1499 -> [w1545 w1616]
          tunnel: [w1551 w1613] -> w1498
          tunnel: w1497 -> [_ w1615]
          tunnel: w1495 -> [_ w1612]
          tunnel: w1484 -> [_ w1611]
          tunnel: w1484 -> [w1544 _]
          tunnel: w1483 -> [w1541 _]
          tunnel: w1482 -> [w1540 _]
          tunnel: w1481 -> [w1538 _]
          frame False {
            w1556 = 0  # Reset Mini DeGausss Sample Counter
            # "Update Last Current AO Index with \nCurrent Sample Index"
            # "Change the Magnitude\nof miniDeGauss:\nAbs(AO_nf) + Abs(AO_on,last) \nUse Max between that and the \ndifference. Difference will be\nminimal in OFF segments, but\nmaximal in ON segments."
            # "Loop Index"
            n616 = Index Array "Flux ON/OFF \nStatus?"(array=w1558, index=w1550) -> (element=w1549:bool)
            n617 = case "Control Sequence Exceeded?" shown="True" w1544 {
              tunnel: [w1569 TRUE] -> w1542
              tunnel: w1543 -> [w1569 _]
              frame False {
              }
              frame True {
                # "No PID Control"
              }
            }
            n618 = case "PID Gain Selector" shown="True" w1549 {
              tunnel: [w1579 w1581] -> w1537
              tunnel: w1559 -> [_ w1581]
              tunnel: w1557 -> [w1579 _]
              tunnel: w1541 -> [_ w1580]
              tunnel: w1540 -> [w1578 _]
              tunnel: [w1578 w1580] -> w1539
              frame False {
                # "Off Sequence"
              }
              frame True {
                # "ON Sequence"
              }
            }
            n619 = case "PID Control ON/OFF?" shown="False" w1542 {
              tunnel: w1561 -> [w1596 _]
              tunnel: w1568 -> [w1595 _]
              tunnel: [w1594 w1610] -> w1548
              tunnel: w1567 -> [_ w1610]
              tunnel: [w1601 w1608] -> w1566
              tunnel: w1565 -> [w1598 w1607]
              tunnel: w1564 -> [w1600 _]
              tunnel: [w1599 w1609] -> w1546
              tunnel: w1563 -> [_ w1606]
              tunnel: w1562 -> [_ w1605]
              tunnel: w1560 -> [w1587 _]
              tunnel: w1555 -> [w1592 w1604]
              tunnel: [FALSE w1604] -> w1554
              tunnel: w1553 -> [w1590 w1603]
              tunnel: [w1590 w1603] -> w1552
              tunnel: w1539 -> [w1589 _]
              tunnel: w1538 -> [w1586 _]
              tunnel: w1537 -> [_ _]
              frame False {
                w1599 = 0  # PID Sample Counter
                # "Offset was added to AO output\nby PID to eliminate the problem of\noutputing 0V for AO when there is \nlittle to no change in PV, which caused\na dip in response until PID recovers."
                # "Tried adding AO 0 to PID AO output. It works find with Null Flux, but \nnot with the anything where AO is not zero. It becomes like a run-away reaction. \nIt turns out that was because I added the indexed Flux value instead of the Null Flux AO.\nProblem Solved"
                # "flux setpoint"
                # "dt"
                # "Reset Array"
                n620 = call-poly <vilib>:"Mean.vi"("X"=w1598) -> ("mean"=w1588:dbl)  [unwired: 1 out]
                n621 = Subtract "PV-SP"(x=w1588, y=w1587) -> (x-y=w1584:dbl)
                n622 = Absolute Value(x=w1584) -> (abs(x)=w1582:dbl)
                n623 = Divide(x=w1582, y=w1586) -> (x/y=w1585:dbl)
                n624 = call-poly <vilib>:"PID Gain Schedule.vi"("PID gain schedule"=w1589, "gain scheduling value"=w1585) -> ("PID gains out"=w1583:T1)  [unwired: 2 in, 1 out]
                n625 = call-poly <vilib>:"PID.vi"("reinitialize? (F)"=w1592, "output range"=T6 {"Max/Min \ncontroller outputs"=10.0, "output low"=-10.0}, "dt (s)"=w1596, "PID gains"=w1583, "process variable"=w1584, "setpoint"=w1595) -> ("output"=w1593:dbl)  [unwired: 4 in, 1 out]
                n626 = Replace Array Subset "Reset Flux Array \nfed to PID"(array=w1598, new element=w1600, index=0) -> (w1601:dbl[])
                n627 = Add "Offset"(x=w1590, y=w1593) -> (x+y=w1594:dbl)
              }
              frame True {
                # "PID Sample Counter Index"
                # "AO last"
                # "Flux AI Reading"
                n628 = Increment "Increment\nto next\nindex"(x=w1606) -> (x+1=w1609:i32)
                n629 = Replace Array Subset "Replace ith item \nin Array fed to PID"(array=w1607, new element=w1605, index=w1606) -> (w1608:dbl[])
              }
            }
            n630 = case "Mini DeGauss Magnitude\nSelector" shown="True" w1549 {
              tunnel: w1552 -> [_ w1577]
              tunnel: [w1572 w1574] -> w1551
              tunnel: [w1571 w1573] -> w1547
              tunnel: w1548 -> [w1571 w1573]
              tunnel: w1545 -> [w1572 _]
              frame False {
              }
              frame True {
                n631 = Absolute Value "Abs[AO_on,last]"(x=w1573) -> (abs(x)=w1576:dbl)
                n632 = Absolute Value "Abs[AO_nf]"(x=w1577) -> (abs(x)=w1575:dbl)
                n633 = Add(x=w1576, y=w1575) -> (x+y=w1574:dbl)
              }
            }
          }
          frame True {
            w1629 = 0  # PID Sample Counter
            # "Leave Index unchanged\nDuring Mini DeGauss\nsequence"
            # "current sample index"
            # "Abs(AO_nf) + Abs(AO_on,last)"
            # "Null Flux AO"
            # "NO PID sequence. DeGaussing Sequence"
            n634 = case "Mini DeGauss Updated AO?" shown="True" w1622 {
              tunnel: w1624 -> [_ w1648]
              tunnel: [w1632 w1646] -> w1623
              tunnel: [w1634 w1647] -> w1621
              tunnel: w1620 -> [w1633 _]
              tunnel: w1617 -> [_ w1645]
              tunnel: w1618 -> [w1632 w1639]
              tunnel: w1616 -> [w1630 w1641]
              tunnel: w1615 -> [w1631 w1643]
              tunnel: [w1631 w1643] -> w1614
              tunnel: [w1630 w1642] -> w1613
              tunnel: w1612 -> [_ w1640]
              tunnel: w1611 -> [_ w1637]
              frame False {
                n635 = Increment "Increment\nto next\nindex"(x=w1633) -> (x+1=w1634:i32)
              }
              frame True {
                w1647 = 0  # Reset Mini DeGausss Sample Counter
                # "No PID Control/DeGauss\nwhen control sequence is exceeded 3/31/2018"
                # "Removed the offset\nand kept amplitude the same"
                # "Take the value once every 15 samples\nInitial curve is sampled at a lot more to \nminimize aliasing of the proper waveform"
                n636 = Index Array "Mini-DeGauss \nON/OFF Status?"(array=w1648, index=w1645) -> (element=w1638:dbl)
                n637 = Subtract "Reset"(x=w1645, y=w1643) -> (x-y=w1644:i32)
                n638 = Greater Or Equal? "Index of Cut off"(x=w1644, y=w1640) -> (x >= y?=w1635:bool)
                n639 = case "Control Sequence Exceeded?" shown="True" w1637 {
                  tunnel: [w1649 TRUE] -> w1636
                  tunnel: w1635 -> [w1649 _]
                  frame False {
                  }
                  frame True {
                    # "No PID Control"
                  }
                }
                n640 = case shown="True" w1636 {
                  tunnel: [w1652 w1654] -> w1646
                  tunnel: w1639 -> [_ w1654]
                  tunnel: w1638 -> [w1652 _]
                  tunnel: [w1651 w1653] -> w1642
                  tunnel: w1641 -> [w1651 w1653]
                  frame False {
                  }
                  frame True {
                  }
                }
              }
            }
            n641 = Replace Array Subset "Reset Flux Array \nfed to PID"(array=w1626, new element=w1625, index=0) -> (w1627:dbl[])
          }
        }
        n642 = shared-variable ".\\Kopco PS Project Target Variables Library.lvlib\\Data RT Exposure"(w1480) -> ()  [unwired: 1 in, 1 out]
        n643 = shared-variable ".\\Kopco PS Project Target Variables Library.lvlib\\Data RT Flux"(w1521) -> ()  [unwired: 1 in, 1 out]
        n644 = case shown="False" w1484 {
          tunnel: [w1656 w1658] -> w1479
          tunnel: w1503 -> [w1656 w1659]
          tunnel: [w1655 w1657] -> w1491
          tunnel: w1490 -> [w1655 w1657]
          frame False {
          }
          frame True {
            (unwired) FALSE ("y")
            # "A Toggle fixed the problem!"
            n645 = case shown="False" w1657 {
              tunnel: [0.0 ("output") w1661] -> w1658
              tunnel: w1659 -> [_ w1661]
              frame False {
                # "Reset AO at the end"
              }
              frame True {
                # "Keep Flux the same"
              }
            }
          }
        }
        n646 = call-poly <vilib>:"DAQmx Write.vi"("task/channels in"=w1533, "data"=w1479, "error in"=w1532) -> ("task out"=w1517:refnum<k21>, "error out"=w1518:errorcluster)  [unwired: 10 in, 1 out]
        n647 = shared-variable ".\\Kopco PS Project Target Variables Library.lvlib\\Data RT Current"(w1479) -> ()  [unwired: 1 in, 1 out]
        n648 = case shown="True" w1484 {
          tunnel: [FALSE w1536] -> w1486
          frame False {
          }
          frame True {
            n649 = shared-variable ".\\Kopco PS Project Target Variables Library.lvlib\\Data Upload"() -> (w1535:bool)  [unwired: 1 in, 1 out]
            n650 = Not "No longer uploading"(x=w1535) -> (.not. x?=w1536:bool)
          }
        }
        n651 = Unbundle By Name(w1518) -> ("status"=w1494:bool)  [unwired: 2 out]
        n652 = Not(x=w1486) -> (.not. x?=w1487:bool)
        n653 = Not(x=w1494) -> (.not. x?=w1488:bool)
        n654 = And(x=w1488, y=w1487) -> (x .and. y?=w1493:bool)
        n655 = shared-variable ".\\Kopco PS Project Target Variables Library.lvlib\\Last Current AO"(w1479) -> ()  [unwired: 1 in, 1 out]
        n656 = node-c288() -> ()  [unwired: 1 in, 1 out]
      }
      n657 = node-c288(w1423) -> (w1408:errorcluster)
      n658 = Flush Stream(8:w1376, 10:w1415, 11:w1377) -> (0:w1416:errorcluster, 3:w1417:refnum<k21>)  [unwired: 1 in, 1 out]
      n659 = Destroy Stream Endpoint(8:w1416, 11:w1417) -> (0:w1412:errorcluster)
      n660 = node-c288(w1441) -> (w1414:errorcluster)
      n661 = shared-variable "NI-GenericDesktopPC-3A84958E\\Kopco PS Project Target Variables Library.lvlib\\Null Flux Running End"(w1387) -> ()  [unwired: 1 in, 1 out]
      n662 = Merge Errors(w1414, w1413, w1408, w1412) -> (w1411:errorcluster)
      "# of Data Points" <- w1378
    }
    frame #21 {
      # "Bound to \"Null Flux Running End\""
      n663 = call <vilib>:"DAQmx Stop Task.vi"("task/channels in"=w1670, "error in"=w1669) -> ("task out"=w1676:refnum<k21>, "error out"=w1675:errorcluster)  [unwired: 12 in]
      n664 = call <vilib>:"DAQmx Clear Task.vi"("task in"=w1676, "error in"=w1675) -> ("error out"=w1672:errorcluster)  [unwired: 13 in]
      n665 = call <vilib>:"DAQmx Stop Task.vi"("task/channels in"=w1671, "error in"=w1672) -> ("task out"=w1674:refnum<k21>, "error out"=w1673:errorcluster)  [unwired: 12 in]
      n666 = call <vilib>:"DAQmx Clear Task.vi"("task in"=w1674, "error in"=w1673) -> ()  [unwired: 13 in, 1 out]
    }
  }
